vi "working_wendy.vi"() -> ()   [LabVIEW 2015]
doc: "This is the interface, the one VI which loads all the others. Run this one first.\n\n(the line below ensures settings are saved)\n[Red Tweezers Save Settings]"
uses:
  subvis/line_trapping.ctl
  subvis/spot.ctl
  <vilib>/userdefined/High Color/IMAQdx.ctl
  subvis/selection_element.ctl
  subvis/mouse_info.ctl
  <vilib>/imath/engines/lvmath/Plug In/_Char/NIMS_CH_character datatype.ctl
  <vilib>/Analysis/baseanly.llb/Real A x B.vi
  subvis/red_tweezers_globals_INTERNAL_VOLATILE.vi
  subvis/red_tweezers_globals.vi
  <vilib>/imath/engines/lvmath/Plug In/_Char/NIMS_CH_Character RV to String.vi
  <vilib>/imath/engines/lvmath2/RunTimeEngine/BuiltInFunctions/title/NIMS_title.vi
  <vilib>/imathl/engines/lvmath/Functions/Error Handling/Create Error.vi
  <vilib>/imath/engines/lvmath2/RunTimeEngine/BuiltInFunctions/xlimit/NIMS_xlimit.vi
  <vilib>/imath/engines/lvmath2/RunTimeEngine/BuiltInFunctions/ylimit/NIMS_ylimit.vi
  <vilib>/imath/engines/lvmath2/RunTimeEngine/IndexRead/NIMS M($,S).vi
  <instcachedir>/0/NIMS M($,S)_3E5749BBB62E49528D4765A77F1F6D98.lvgen/NIMS M($,S)_3E5749BBB62E49528D4765A77F1F6D98_000.vi
  <vilib>/imath/engines/lvmath2/RunTimeEngine/BuiltInFunctions/plot/NIMS_plot(RM, RM, Str).vi
  <vilib>/imath/engines/lvmath2/RunTimeEngine/ErrorHandling/NIMS_Finalize Error.vi
  <vilib>/Analysis/NI_AALBase.lvlib
  <vilib>/vision/driver/NI_Vision_Acquisition_Software.lvlib
  <vilib>/vision/NI_Vision_Development_Module.lvlib
panel:
  out "Spot Storage":T1[](array[typedef]) {"Amplitude Correction" step=0.1; "Line Trapping"."Phase Gradient" step=0.05; "Line Trapping"."Vector"."x" step=1e-06 format="%#_6p"; "Line Trapping"."Vector"."y" step=1e-06 format="%#_6p"; "Line Trapping"."Vector"."z" step=1e-06 format="%#_6p"; "NA Position"."r" step=1e-06; "NA Position"."y" step=1e-06; "NA Position"."x" step=1e-06; "Position"."z" step=1e-06; "Position"."y" step=1e-06; "Position"."x" step=1e-06; "Phase" step=0.7753; "Intensity" step=0.1}
  out "# selected":i16
  out "Last Pattern":T1[](array[typedef]) {"Amplitude Correction" step=0.1; "Line Trapping"."Phase Gradient" step=0.05; "Line Trapping"."Vector"."x" step=1e-06 format="%#_6p"; "Line Trapping"."Vector"."y" step=1e-06 format="%#_6p"; "Line Trapping"."Vector"."z" step=1e-06 format="%#_6p"; "NA Position"."r" step=1e-06; "NA Position"."y" step=1e-06; "NA Position"."x" step=1e-06; "Position"."z" step=1e-06; "Position"."y" step=1e-06; "Position"."x" step=1e-06; "Phase" step=0.7753; "Intensity" step=0.1}
  out "Plugins":T3(array[cluster])=[{"Name"="ASI Stage", "Folder"=path "C:/Users/Richard Bowman/Dropbox/red_tweezers_1_4_rc4/plugins/ASI Stage.llb", "vi reference"=refnum, "Needs to be run"=TRUE, "Error"={"status"=FALSE, "code"=0, "source"=""}}, {"Name"="iTweezers", "Folder"=path "C:/Users/Richard Bowman/Dropbox/red_tweezers_1_4_rc4/plugins/iTweezers.llb", "vi reference"=refnum, "Needs to be run"=TRUE, "Error"={"status"=FALSE, "code"=0, "source"=""}}, {"Name"="MightexLED", "Folder"=path "C:/Users/Richard Bowman/Dropbox/red_tweezers_1_4_rc4/plugins/MightexLED.llb", "vi reference"=refnum, "Needs to be run"=TRUE, "Error"={"status"=FALSE, "code"=0, "source"=""}}]
  in  "Tab":T4(tab)
  out "Y":dbl
  out "X":dbl
  in  "O Button":bool
  in  "OK Button":bool
  in  "Bubble Size":dbl=50.0002
  out "Hit Indicator":bool
  in  "On":bool
  out "Induce check":bool
  out "Area+ Buffer":dbl
  in  "Area to check":dbl=0.00025
  out "Prev Current Spot":dbl
  out "spots selected 2":i32=4
  out "Spot # Check":dbl
  out "Orig Y SC":dbl
  out "Orig X SC":dbl
  out "ID num check":dbl
  out "Value Check":dbl
  out "ID":dbl[](array[numeric])
  out "Null array":dbl[](array[numeric])
  out "Potential Collisions":dbl
  out "What to Check":dbl[](array[numeric])
  out "String counter":dbl
  out "Counter for String":dbl
  out "Numeric 4":dbl
  out "LCounter":dbl
  out "Numeric 3":dbl
  out "Num":dbl
  out "Old Y":dbl
  out "Old X":dbl
  out "init":dbl
  out "Looper":bool
  in  "Output to SLM":bool
  out "Maximum":dbl
  out "Projected Distance":dbl
  out "Previous Distance":dbl
  out "Group ID #":dbl
  in  "Buffer Zone":dbl=7e-05
  out "# of Spots":dbl
  out "Distance":dbl
  out "Hit":bool
  out "Y Displacement":dbl
  out "X Displacement":dbl
  out "Current Spot #":dbl
  out "spots selected":i32=4
  in  "lock aspect ratio":bool=TRUE
  in  "Size":cluster{"x":dbl, "y":dbl, "z":dbl} {"z" step=1e-06 format="%#_4p"; "y" step=1e-06 format="%#_4p"; "x" step=1e-06 format="%#_4p"}
  in  "Position":cluster{"x":dbl, "y":dbl, "z":dbl}={"x"=1e-06, "y"=-6.3e-06, "z"=0.0} {"z" step=1e-06 format="%#_4p"; "y" step=1e-06 format="%#_4p"; "x" step=1e-06 format="%#_4p"}
  in  "phase":dbl step=0.7753
  in  "Vortex Charge":i8
  in  "Intensity":dbl=1.0 step=0.1
  in  "add to selection":bool
  in  "random position":bool
  in  "new spot":bool
  in  "delete":bool
  in  "rotate":bool
  in  "Rotation Axis":u16(ring)=2 items=["Z", "X", "Y", "Custom"]
  in  "Angle (degrees)":dbl=2.0
  in  "Custom Axis":cluster{dbl, dbl, dbl}
  in  "Spot Shape":enum32{"Normal", "Line", "NA", "Mixed"}(tab)=enum."Mixed"
  in  "Line Trapping":T2 {"Phase Gradient" step=0.05; "Vector"."x" step=1e-06 format="%#_4p"; "Vector"."y" step=1e-06 format="%#_4p"; "Vector"."z" step=1e-06 format="%#_4p"}
  in  "Scale back aperture":dbl=1.1 step=0.1
  in  "Scale BA":bool
  in  "Position on back aperture":cluster{"x":dbl, "y":dbl}={"x"=-5.84327907697451e-18, "y"=0.0} {"y" step=0.1 format="%#_4p"; "x" step=0.1 format="%#_4p"}
  in  "Radius on back aperture":dbl=1.1 step=0.1
  in  "Generate":bool
  in  "Pattern":T5(tab)
  in  "Spots across centre":i32=5
  in  "Reference Array?":bool
  in  "Fraction of SLM":dbl=1.0
  in  "Spots across centre":i32=5
  in  "N":cluster{i32, i32}
  in  "spacing/m":dbl=2.0
  in  "Iterations":i32=10
  out "non-uniformity":dbl(slide)=0.031119223416512406 scale=0.0..0.2
  out "efficiency":dbl(slide)=0.8985936267644501 scale=0.0..1.0
  in  "Optimise":bool
  in  "Reset Phase/Amplitude":bool
  in  "Fall-off/m":dbl=0.00025 min=0.0 step=1e-06 format="%#_4p"
  in  "Abort Plugin":bool
  in  "Plugin:":u16(ring)=1 items=["ASI Stage", "iTweezers", "MightexLED"]
  in  "Save Video":bool
  in  "Global ROI (requires restart)":i32[](array[numeric])=[0, 0, 1280, 512]
  in  "Zoom":bool
  in  "Draw ROI":bool
  in  "Zoom to Fit":bool
  out "Image Information":string="640x480 1.93X 8-bit image 255    (0,0)"
  in  "Camera":T6
  in  "Time per Frame (ms)":dbl
  in  "Edit Sequence Mode":bool
  in  "Manual Edit":bool
  in  "Bubble ID to Empty":dbl
  in  "Clearance Button":bool
  in  "Manual Sequence":bool
  in  "Play Sequence":bool
  in  "Reset":bool
  out "Sequence Instances":dbl
  out "Counter":dbl
  in  "Save State":bool
  out "Sequence On?":bool
  in  "Sequence Order":dbl
  out "Selection/Group":T7[](array[typedef])
  in  "Sequence Storer":T1[][](array[typedef]) {"Amplitude Correction" step=0.1; "Line Trapping"."Phase Gradient" step=0.05; "Line Trapping"."Vector"."x" step=1e-06 format="%#_6p"; "Line Trapping"."Vector"."y" step=1e-06 format="%#_6p"; "Line Trapping"."Vector"."z" step=1e-06 format="%#_6p"; "NA Position"."r" step=1e-06; "NA Position"."y" step=1e-06; "NA Position"."x" step=1e-06; "Position"."z" step=1e-06; "Position"."y" step=1e-06; "Position"."x" step=1e-06; "Phase" step=0.7753; "Intensity" step=0.1}
  in  "Rates":bool
  out "Rates":dbl
  out "LCS":dbl
  in  "Add Additional Frames":bool
  in  "Frame Location":dbl
  in  "Additional Frames Wanted":dbl
  in  "Initiate Creation":bool
  in  "Number of Planned Sequence Frames":dbl
  in  "Max Number of Bubbles":dbl
  in  "Tab Control":enum32{"Line", "Arc"}(tab)
  out "X Rate":dbl
  out "Y Rate":dbl
  out "Degree Rate":dbl
  out "Radians":dbl
  out "Center Y":dbl
  out "Center X":dbl
  in  "Radius X":dbl
  in  "Theta":dbl
  in  "Lock Current Spot":bool
  out "Locked Current Spot":dbl
  out "Numeric":dbl
  out "probe":dbl
  in  "Insert":bool
  in  "Start at Which Frame?":dbl
  out "Original Y":dbl
  out "Original X":dbl
  in  "Mark Original Position":bool
  in  "How Many Frames?":dbl
  out "New Y":dbl
  out "New X":dbl
  out "Spot Storage 2":T1[](array[typedef]) {"Amplitude Correction" step=0.1; "Line Trapping"."Phase Gradient" step=0.05; "Line Trapping"."Vector"."x" step=1e-06 format="%#_6p"; "Line Trapping"."Vector"."y" step=1e-06 format="%#_6p"; "Line Trapping"."Vector"."z" step=1e-06 format="%#_6p"; "NA Position"."r" step=1e-06; "NA Position"."y" step=1e-06; "NA Position"."x" step=1e-06; "Position"."z" step=1e-06; "Position"."y" step=1e-06; "Position"."x" step=1e-06; "Phase" step=0.7753; "Intensity" step=0.1}
  in  "Save":bool
  in  "Load":bool
  in  "Camera Capture":bool
  out "Bubble y":dbl
  out "Bubble x":dbl
  out "Number of Matches Returned":dbl
  out "bottomry":dbl
  out "toply":dbl
  out "bottomrx":dbl
  out "toplx":dbl
  in  "Send Data":bool
  out "Camera 2":T8(plugin-control)
  out "Circles":T9(array[cluster]) {"Position"."Y" format="%.2f"; "Position"."X" format="%.2f"}
  out "Video Frame Rate":dbl(knob)=50.00000000000003 scale=0.0..100.0 scale format="%.1f"
  out "Interface Frame Rate":dbl(knob)=97.23240312927678 scale=0.0..100.0 scale format="%.1f"
  in  "stop":bool=TRUE
  out "1 for original positon":dbl
  out "MOP pressed":bool
  out "MOP pressed After":bool
  out "X Pos every 10 sec":dbl
  out "Elapsed Time":dbl
  out "Sequence Frames To Check":string
  out "Position Indicator":string
  in  "Clear String":bool
  out "String 2":string
  out "Collision Detector":string
  out "Array":dbl[](array[numeric])
  out "Spot Checker":T1[](array[typedef]) {"Amplitude Correction" step=0.1; "Line Trapping"."Phase Gradient" step=0.05; "Line Trapping"."Vector"."x" step=1e-06 format="%#_6p"; "Line Trapping"."Vector"."y" step=1e-06 format="%#_6p"; "Line Trapping"."Vector"."z" step=1e-06 format="%#_6p"; "NA Position"."r" step=1e-06; "NA Position"."y" step=1e-06; "NA Position"."x" step=1e-06; "Position"."z" step=1e-06; "Position"."y" step=1e-06; "Position"."x" step=1e-06; "Phase" step=0.7753; "Intensity" step=0.1}
  out "Image":T8(plugin-control)
  # "Notes:\n\nIf you are doing non-sequence controls,\nthe delete function can be used as intended.\nHowever, do not use the delete function after\nrunning a sequence! Using it will prevent\nthe bubbles from appearing as the\nnumber of spots will change, which is\nessential for the sequence to work (it would\nbe displaying the maximum number of\nbubbles). \n\nIf you happen to delete a bubble, it can be \nrestored by inserting a new spot. Once enough\nspots have been restored, click on manual edit\nto correct the # of spots tracker. It should \nbe restored to where it originally was."
  # "The SLM can be used to shape spots; here you can restrict the NA of a spot (so it comes only from part of the back aperture), or create a line-trap"
  # "The traps do not have any spot-shaping applied (so they should just be diffraction-limited focal spots)."
  # "This shapes the amplitude (and phase) of the beam to create extended line traps.  The \"Phase Gradient\" control allows the Poynting vector to push things along the line.  Unfortunately, some work is needed on the scaling factors so the phase gradient control will need tweaking if the line trap has a nonzero z component."
  # "By default,each spot comes from the whole back aperture.  Here, you can limit a spot to come from a specific part of the back aperture."
  # "The control below allows you to scale the whole back aperture (i.e. the position and size of all the apertures).  It's a one-time operation, i.e. only changes things when you push \"ok\"."
  # "A Combination of line-trapping and NA restriction has been applied to these traps.  You can get at the line trap or NA parameters on the other tabs, switching to the NA tab does not delete the line-trap settings."
  # "This tab generates Shack-Hartmann type holograms, which are often useful when aligning the system, and arrays of spots."
  # "The controls above only work when using the \"IMAQdx with ROI Buttons\" case in the bottom loop.  You can save video regardless of camera code though."
  # "Manual Edit allows a user to\ngo to a specific sequence frame."
  # "To clear the sequence, you must\nclear the array. Right click on sequence\nstorer to do this."
  # "Use this to \"clear\" a \nspecific bubble. If\nworking on a sequence,\nuse this as your delete\nbutton! You can update\nthe view by using manual edit."
  # "Use the reset button\nto clear counter.\nIt becomes necessary\nwhen you clear the array,\nespecially in manual mode."
  # "Use the sequence creator tab to specify the\nnumber of bubbles you want along with\nthe number of frames.\n\nTo save at a specific interval, the sequence\norder can be used to place the state. If used\nto correct something, it will replace the\nentire sequence frame.\n\n\"Sequence On?\" is only used in auto mode."
  # "Frame Location must be\nwhere you want to add\nthe frames to (ie having \n4 as an input would have\nthe additional frames\nstart at array row 5."
  # "Multiple bubbles can  be done with the\nline function. One bubble at a time for the arc\nfunction."
  # "Using the Load/Save function:\n\nRed Tweezers itself is unable to save long \nsequences, but a separate program is able to\naccomplish this. To do this, follow these\nsteps:\n\n1. After creating your sequence, press the save\nbutton below.\n\n2. Then, go to the subvi folder and find\nSequenceSaver.vi.\n\n3. At the control \"Sequence Storer,\" right-click\nthe dimensions part of the array and go to\ndata operations.\n\n4. Press \"Make Current Values Default\" and save\nthe sequence.\n\n5. The next time you load the program, simply\npress load to re-acquire the sequence. You\nwill need to insert the bubbles again, but after\nthe first frame can be recovered by using\nSequenceControl.vi."
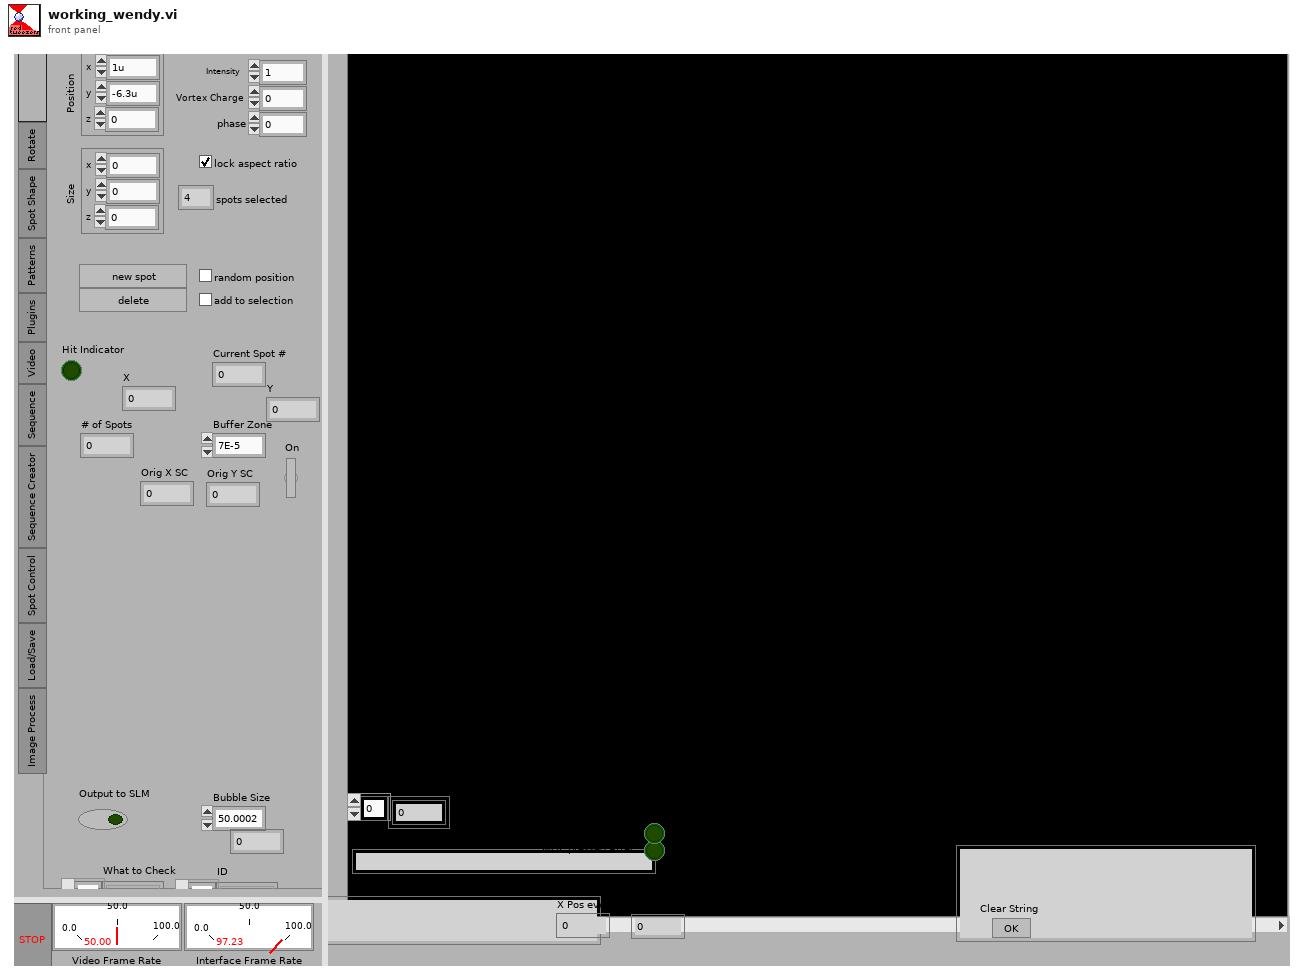
[diagram p1: front panel]
types:
  T1 = typedef "spot.ctl" = cluster{"Position":cluster{"x":dbl, "y":dbl, "z":dbl}, "Intensity":dbl, "Vortex Charge":i8, "Phase":dbl, "NA Position":cluster{"x":dbl, "y":dbl, "r":dbl}, "Line Trapping":T2, "Amplitude Correction":dbl}
  T2 = typedef "line_trapping.ctl" = cluster{"Vector":cluster{"x":dbl, "y":dbl, "z":dbl}, "Phase Gradient":dbl}
  T3 = cluster{"Name":string, "Folder":path, "vi reference":refnum<vi>, "Needs to be run":bool, "Error":errorcluster}[]
  T4 = enum32{"Current Spot", "Rotate", "Spot Shape", "Patterns", "Plugins", "Video", "Sequence", "Sequence Creator", "Spot Control", "Load/Save", "Image Process"}
  T5 = enum32{"HCP Shack-Hartmann", "Square Shack-Hartmann", "Rectangular Grid"}
  T6 = typedef "IMAQdx.ctl" = refnum<k21>
  T7 = typedef "selection_element.ctl" = cluster{"Group ID":i32, "Selected":bool}
  T8 = typedef "IMAQ Image.ctl" = refnum<image>
  T9 = cluster{"Position":cluster{"X":sgl, "Y":sgl}, "Radius":dbl, "Score":dbl}[]
  T10 = typedef "mouse_info.ctl" = cluster{"Button Down":bool, "Dragging":bool, "Position (Image Pixels)":cluster{"X":dbl, "Y":dbl}, "Previous Position (Image Pixels)":cluster{"X":dbl, "Y":dbl}, "Button":u16, "Mods":cluster{"Double Click":bool, "Menu Key":bool}, "PlatMods":cluster{"Shift":bool, "Ctrl":bool, "Alt":bool, "Cmd":bool, "Opt":bool}}
  T11 = typedef "NIMS_CH_character datatype.ctl" = cluster{"Numeric":u8}
  T12 = cluster{"Position":cluster{"x":dbl, "y":dbl, "z":dbl}, "Intensity":dbl, "Vortex Charge":i8, "Phase":dbl, "NA Position":cluster{"x":dbl, "y":dbl, "r":dbl}, "Line Trapping":T2, "Amplitude Correction":dbl}
  T13 = enum16{"Set guide visibility", "Set grid visibility", "Show front panel", "Render on image"}
  T14 = enum32{"Current Spot", "Rotate", "Spot Shape", "Patterns", "Plugins", "Video"}
  T15 = enum16{"Left Button", "Center Button", "Right Button", "Window Close"}
  T16 = typedef "Image Type" = u32
  T17 = cluster{"number: 0 to 1":dbl, "number: 0 to 1":dbl}
  T18 = typedef "NI_Matrix.lvlib/RealMatrix.ctl" = dbl[][]
  T19 = typedef "overlay_element.ctl" = cluster{"Tool":enum16{"Lines", "Oval", "Rectangle", "Text"}, "Points":cluster{"X":dbl, "Y":dbl}[], "Drawing Mode":u32, "Color":u32, "String":string}
  T20 = enum32{"Current Spot", "Rotate", "Spot Shape", "Patterns", "Plugins", "Video", "Particle Tracking", "Clamping", "Blank"}[]
  T21 = typedef "LVMenuShortCut.ctl" = cluster{"include Shift key?":bool, "include Ctrl key?":bool, "shortcut key":string}
  T22 = typedef "LVPoint32TypeDef.ctl" = cluster{"Horizontal":i32, "Vertical":i32}
  T23 = cluster{"Shift":bool, "Ctrl":bool, "Alt":bool, "Cmd":bool, "Opt":bool}
  T24 = cluster{"Button Down":bool, "Dragging":bool, "Mouse Coords (image pixels)":cluster{dbl, dbl}, "Mouse Coords (image pixels)":cluster{dbl, dbl}, "Button":u16, "Mods":cluster{"Double Click":bool, "Menu Key":bool}, "PlatMods":cluster{"Shift":bool, "Ctrl":bool, "Alt":bool, "Cmd":bool, "Opt":bool}}
  T25 = cluster{"Position":cluster{"X":sgl, "Y":sgl}, "Radius":dbl, "Score":dbl}
  T26 = cluster{"[0]":dbl, "[1]":dbl, "[2]":dbl, "[3]":dbl}
  T27 = cluster{"Average Frame Time":dbl, "millisecond timer value":u32}
  T28 = cluster{"Position":cluster{"x":dbl, "y":dbl, "z":dbl}, "Intensity":dbl, "Vortex Charge":i8, "Phase":dbl, "NA Position":cluster{"x":dbl, "y":dbl, "r":dbl}, "Line Trapping":T2, "Amplitude Correction":dbl}[]
  T29 = enum32{"Bad", "Idle", "Run top level", "Running"}
  T30 = typedef "AviRefnum.ctl" = refnum<k1>
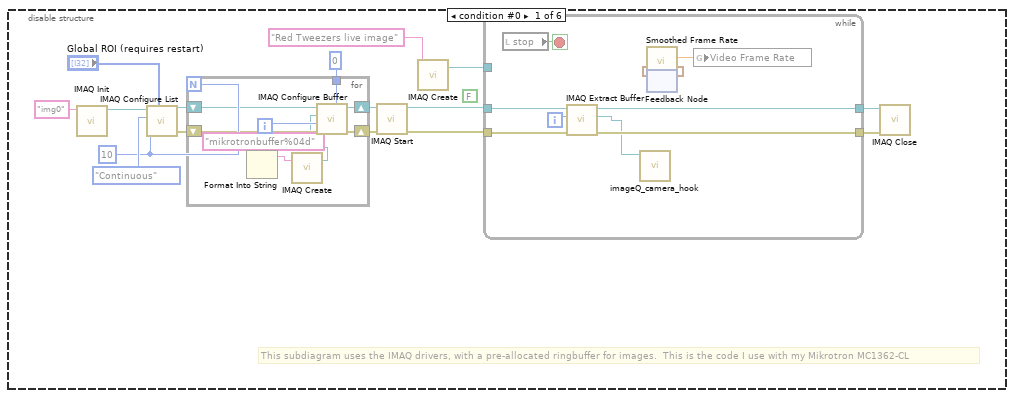
[diagram p3: hidden frame]
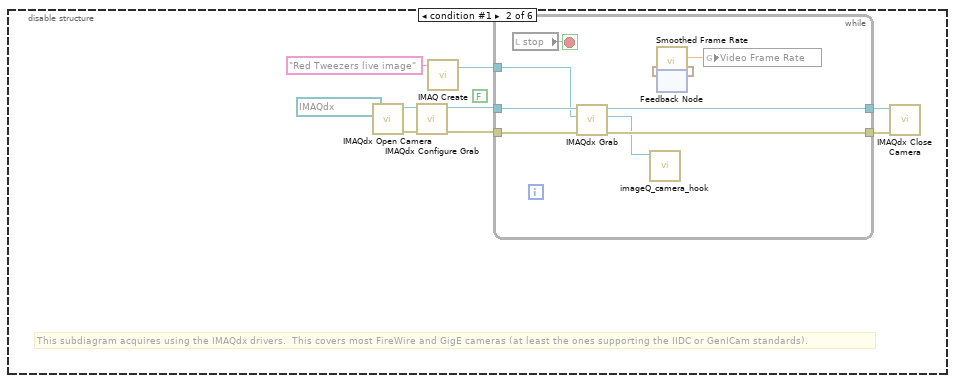
[diagram p4: hidden frame]
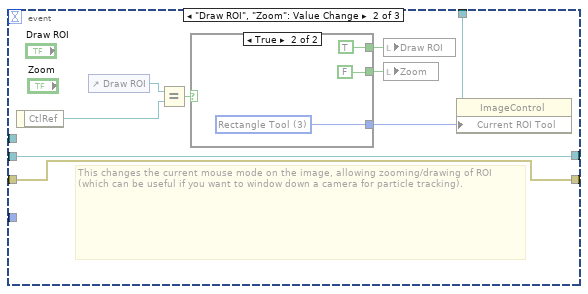
[diagram p5: hidden frame]
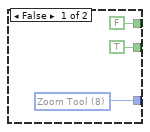
[diagram p6: hidden frame]
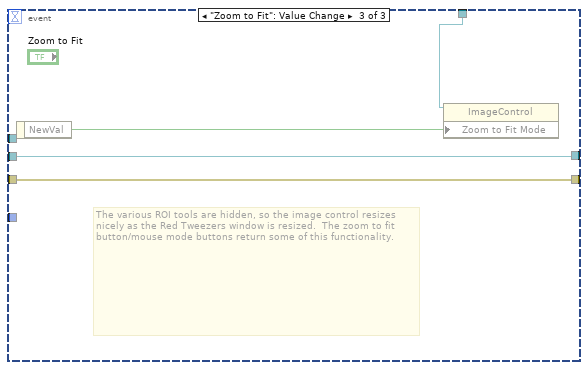
[diagram p7: hidden frame]
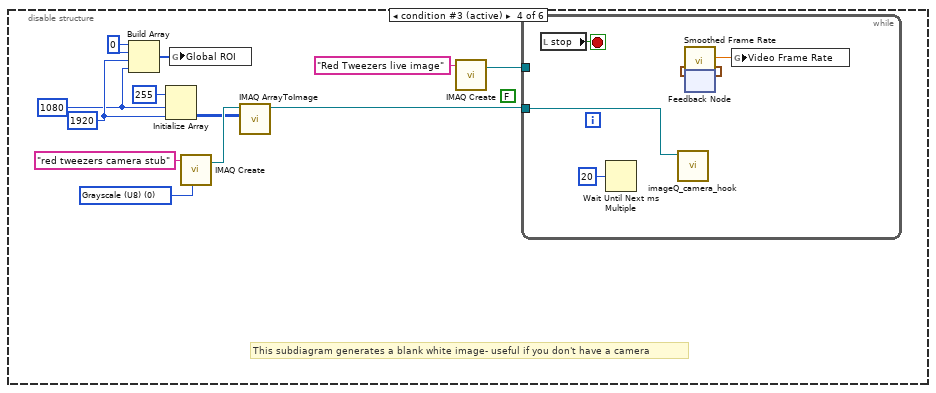
[diagram p8: hidden frame]
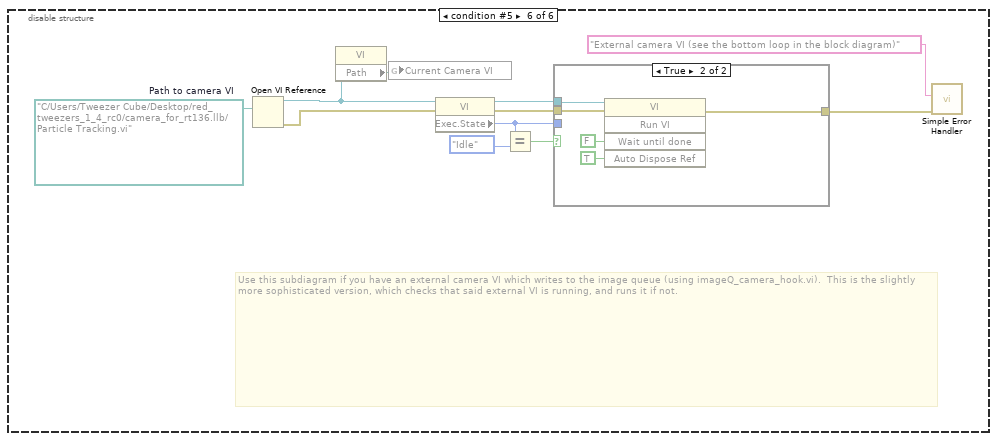
[diagram p10: hidden frame]
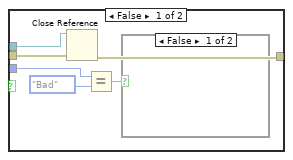
[diagram p11: hidden frame]
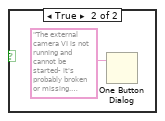
[diagram p12: hidden frame]
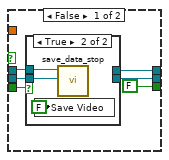
[diagram p13: hidden frame]
diagram:
  w11 = "red_tweezers_display_imageQ" ("Queue Name")
  w23 = T10 {"Button Down"=FALSE, "Dragging"=FALSE, "Position (Image Pixels)"={"X"=0.0, "Y"=0.0}, "Previous Position (Image Pixels)"={"X"=0.0, "Y"=0.0}, "Button"=0, "Mods"={"Double Click"=FALSE, "Menu Key"=FALSE}, "PlatMods"={"Shift"=FALSE, "Ctrl"=FALSE, "Alt"=FALSE, "Cmd"=FALSE, "Opt"=FALSE}}  # Mouse Information
  w24 = refnum<vi> refnum  # Image
  # "The funny looking feedback-node structure is deliberate (if odd).  We want to reload settings from the last used file (stored in the registry) only if this program has not been run since it was last loaded from file/recompiled.  That's why I use an uninitialised shift register: every time the program runs, it increments.  So, if it is zero, this is our first run (or we've been recently recompiled)."
  # "This loop handles the video that is displayed on-screen and saved to file."
  # "Initially, we only register to be told when the user clicks the image"
  # "This is the actual image control"
  # "This is a generic reference.\nIt is just a placeholder, so we can register for events later."
  # "This version of red tweezers uses two coordinate systems: \n1. Real Coordinates - corresponding to physical distances in 3D in microns\n2. Image Coordinates - position on the camera image, relative to the top left of the CURRENT ROI, measured in pixels. If the ROI changes, the relationship between \"real units\" and \"image pixels\" may change, so all values should be stored and presented to the user in REAL units unless there is a good reason to do otherwise."
  n1 = control-ref of="Plugin Pnl"() -> (w20:refnum<vi>)
  n2 = flat-sequence {
    tunnel: [w27] -> w6
    tunnel: w4 -> [_]
    frame #0 {
      n3 = vi-ref "red_tweezers_globals_INTERNAL.vi"() -> (w28:refnum<vi>)
      n4 = property class="VI"(reference=w28) -> ("Path"=w27:path)  [unwired: 1 in, 2 out]
      n5 = global write "red_tweezers_globals_INTERNAL_VOLATILE.vi" "Current Camera VI"(w27) -> ()
    }
  }
  n6 = control-ref of="Plugin:"() -> (w21:refnum<vi>)
  n7 = feedback #1() -> (w14:dbl)  [unwired: 1 in]
  n8 = Equal To 0?(x=w14) -> (x = 0?=w13:bool)
  n9 = Increment(x=w14) -> (x+1=w12:dbl)
  n10 = feedback-in #1(w12) -> ()
  n11 = call "plugins_load.vi"("Sub Panel"=w20, "Plugin Chooser"=w21) -> ("error out"=w15:errorcluster, "Plugins"=w17:T3)  [unwired: 2 in, 2 out]
  "Plugins" <- w17
  n12 = control-ref of="Image"() -> (w5:refnum<vi>)
  n13 = case shown="True" w13 {
    tunnel: w15 -> [_ w29]
    tunnel: [_ w29] -> w4
    frame False {
    }
    frame True {
      n14 = call "settings_load_default_file.vi"("error out"=w29) -> ()
    }
  }
  n15 = flat-sequence {
    tunnel: w4 -> [_]
    tunnel: w2 -> [w31]
    frame #0 {
      # "ensure we don't accidentally start saving video, and run UDP Sender to set up the hologram window."
      n16 = local write "Save Video"(FALSE ("background subtraction")) -> ()
      n17 = call "UDP Sender generic_2.vi"("Spots"=w31) -> ()  [unwired: 2 in, 1 out]
    }
  }
  n18 = global read "red_tweezers_globals.vi" "Selection/Group"() -> (w22:T7[])
  n19 = register-events(w5, w24, w24, w24) -> (reference out=w25:refnum<event-registration>)  [unwired: 2 in, 1 out]
  n20 = global read "red_tweezers_globals.vi" "Spots"() -> (w2:T1[])
  n21 = local write "stop"(FALSE ("STOP")) -> ()
  n22 = call "ensure_selection_matches_spots.vi"("Selection and Groups in"=w22, "Spots"=w2) -> ("Selection and Groups out"=w26:T7[], "Spots (duplicate)"=w1:T1[])  [unwired: 4 in]
  n23 = call "IMAQ Create"("Image Name"=w11) -> ("New Image"=w9:T8)  [unwired: 4 in, 1 out]
  n24 = call "imageQ_create_return_queue.vi"("Queue Name"=w11) -> ("queue out"=w10:refnum<queue>)
  n25 = while {
    shift-right: [w119] -> _
    shift-left: w1 -> [w139]
    shift-right: [w138] -> _
    shift-left: w26 -> [w137]
    shift-right: [w141] -> _
    shift-left: _ -> [w132]
    shift-right: [w140] -> _
    shift-left: _ -> [w131]
    tunnel: w5 -> [w136]
    shift-right: [w130] -> _
    shift-left: w23 -> [w129]
    shift-right: [w133] -> _
    shift-left: w25 -> [w134]
    border: errorcluster {"status"=FALSE, "code"=0, "source"=""} ("error out") -> [_]
    tunnel: [errorcluster {"status"=FALSE, "code"=0, "source"=""} ("error in (no error)")] -> w18
    border: w17 -> [_]
    tunnel: w1 -> [w120]
    stop <- w121 stop-if-true
    w34 = 1
    w43 = 7 items=["Red", "Green", "Blue", "Hue", "Saturation", "Luminance", "Value", "Intensity"] ("Color Plane")
    w47 = T16 0 items=["Grayscale (U8)", "Grayscale (I16)", "Grayscale (SGL)", "Complex (CSG)", "RGB (U32)", "HSL (U32)", "RGB (U64)", "Grayscale (U16)"] ("Image Type")
    # "Don't Need. For Matlab Part."
    # "The function inserts the newly generated sequence for the automatic sequence generator. It also contains the code\nthe code necessary to check whether the bubbles will intersect with each other in the sequence."
    # "This calculates the size of the area including the buffer zone length.\nThe bubble diameter will also be included in the near future."
    # "The statement to the right controls the area that are being chcecked and checks\nwhich bubbles need to be checked.  There are two instances where this activates\nin this case:\n\nWhen a new bubble is selected\nWhen a bubble is deselected, reverting to the last current spot #\n\nThe other case, when the bubble moves out of the area specified, is located\ninside the while loop controlling the bubble movement with a mouse."
    # "Timer function example"
    # "These functions help with the calculations for the sequence generator."
    # "This loads the sequence from the \"saver\" VI. The save function below \"saves\" the sequence into the saver VI."
    # "The VI above is SequenceSaver.vi which contains the\ncode necessary to create a sequence."
    # "This case structure is the Save State structure. This stores\nthe current state of the bubbles (ie position)."
    # "Reset sets the counter back to zero. This is particularly useful \nwhen using the manual sequence."
    # "This case structure helps to continue the sequence.\nThis takes the true case of the Sequence On? function\nor the true case for the Manual Sequence function\nin order to go to the next sequence frame."
    # "This case structure allows for the playing of the sequence.\nThe amount of time it takes to go through the sequence\ncan be edited on the current spot menu."
    # "We only write to the image overlay when we are in one of the tabs, to prevent it disappearing when we are (for example) using the mouse."
    # "These wires control saving undo info. See the VI below's tip strips for details."
    # "Setting these wires to false means:\n(1) dragging moves the selection\n(2) clicking spots changes selection\nset them to true to stop the default mouse behaviour, don't wire them straight through!"
    n26 = event shown="[6] <Image>: Mouse Move" {
      selector: w134 -> [w679 w1351 w1356 w1578 w1606 w1623 w1720 _]
      dyn-events: [w679 w1350 w1356 w1576 w1603 w1624 w1720 _] -> w133
      timeout: 0 -> [_ _ _ _ _ _ _ _]
      tunnel: [w687 _ w1358 w1573 w1608 w1615 w1707 _] -> w141
      tunnel: [w686 _ w1357 w1572 w1607 w1614 w1711 _] -> w140
      tunnel: [w685 _ _ _ _ _ _ _] -> w92
      tunnel: w139 -> [w684 w1346 w1363 w1568 w1601 w1620 w1715 w2038]
      tunnel: [w683 w1346 w1361 w1568 w1601 w1611 w1713 w2038] -> w127
      tunnel: [w682 w1345 w1360 w1557 w1600 w1621 w1703 w2037] -> w126
      tunnel: w137 -> [w681 w1345 w1362 w1557 w1600 w1619 w1714 w2037]
      tunnel: w136 -> [w680 w1347 w1353 w1567 w1604 w1622 w1716 _]
      tunnel: [w678 _ w1355 w1577 T10 {"Button Down"=FALSE, "Dragging"=FALSE, "Position (Image Pixels)"={"X"=0.0, "Y"=0.0}, "Previous Position (Image Pixels)"={"X"=0.0, "Y"=0.0}, "Button"=0, "Mods"={"Double Click"=FALSE, "Menu Key"=FALSE}, "PlatMods"={"Shift"=FALSE, "Ctrl"=FALSE, "Alt"=FALSE, "Cmd"=FALSE, "Opt"=FALSE}} T10 {"Button Down"=FALSE, "Dragging"=FALSE, "Position (Image Pixels)"={"X"=0.0, "Y"=0.0}, "Previous Position (Image Pixels)"={"X"=0.0, "Y"=0.0}, "Button"=0, "Mods"={"Double Click"=FALSE, "Menu Key"=FALSE}, "PlatMods"={"Shift"=FALSE, "Ctrl"=FALSE, "Alt"=FALSE, "Cmd"=FALSE, "Opt"=FALSE}} w1719 _] -> w130
      tunnel: w129 -> [w678 _ w1355 _ _ w1618 w1710 _]
      tunnel: w132 -> [_ _ w1358 w1573 w1608 w1615 w1707 _]
      tunnel: w131 -> [_ _ w1357 w1572 w1607 w1614 w1711 _]
      tunnel: [w677 _ _ _ _ _ _ _] -> w128
      tunnel: [_ _ w1354 _ _ _ TRUE _] -> w125
      tunnel: [_ _ _ TRUE TRUE TRUE FALSE _] -> w124
      tunnel: [TRUE _ _ _ _ _ _ _] -> w122
      tunnel: [_ _ _ _ _ _ _ "stop"] -> w121
      tunnel: w120 -> [_ _ _ _ _ _ w1704 _]
      event Timeout {
        n27 = event-data() -> ()  [unwired: 1 in, 1 out]
        n28 = case shown="\"Current Spot\", Default" "Tab" {
          tunnel: [w703 w971 w1118 w1220 w1301 w1339] -> w683
          tunnel: w684 -> [w700 w973 w1119 w1222 w1301 w1339]
          tunnel: w681 -> [w689 w972 w1116 w1221 w1300 w1338]
          tunnel: [w702 w970 w1117 w1219 w1300 w1338] -> w682
          tunnel: [w690 _ TRUE _ _ _] -> w687
          tunnel: [w690 _ _ _ _ _] -> w686
          tunnel: [_ _ _ FALSE _ _] -> w685
          tunnel: w680 -> [_ _ _ _ _ w1335]
          tunnel: w678 -> [_ _ w1098 _ _ _]
          tunnel: [_ _ w1100 _ _ _] -> w677
          frame "Current Spot", Default {
            w690 = FALSE
            # "The function below contains the code necessary to use the automatic sequence generator to create specific movements. It also helps translate cases where the point is entered in not dragged.\nThis prevents bubbles from intersecting if the bubble is told not to intersect."
            # "If it's out of date, update front panel"
            n29 = call "find_centroid.vi"("Selection and Groups"=w689, "Spots"=w700) -> ("Mean Values"=w698:T1, "size"=w692:cluster{"x":dbl, "y":dbl, "z":dbl}, "centroid"=w693:cluster{"x":dbl, "y":dbl, "z":dbl}, "# selected"=w691:i16)  [unwired: 2 in, 1 out]
            n30 = stacked-sequence {
              tunnel: w691 -> [_ w705]
              frame #0 {
                n31 = local read "spots selected"() -> (→"spots selected 2":i32)
              }
              frame #1 {
                "spots selected" <- w705
              }
            }
            n32 = feedback-in #2(w698) -> ()
            n33 = feedback #2() -> (w699:T1)  [unwired: 1 in]
            n34 = feedback #3() -> (w697:cluster{"x":dbl, "y":dbl, "z":dbl})  [unwired: 1 in]
            n35 = feedback-in #3(w692) -> ()
            n36 = Not Equal?(x=w699, y=w698) -> (x != y?=w696:bool)
            n37 = Not Equal?(x=w697, y=w692) -> (x != y?=w695:bool)
            n38 = Or(x=w696, y=w695) -> (x .or. y?=w694:bool)
            n39 = case shown="True" w694 {
              tunnel: w698 -> [_ w711]
              tunnel: w692 -> [_ w707]
              frame False {
              }
              frame True {
                n40 = Unbundle By Name(w711) -> ("Position"=w706:cluster{"x":dbl, "y":dbl, "z":dbl}, "Intensity"=w709:dbl, "Vortex Charge"=w708:i8, "Phase"=w710:dbl)
                n41 = local write "Size"(w707) -> ()
                n42 = local write "Vortex Charge"(w708) -> ()
                n43 = local write "Intensity"(w709) -> ()
                n44 = local write "Position"(w706) -> ()
                n45 = local write "phase"(w710) -> ()
                n46 = Unbundle By Name(w706) -> ()  [unwired: 2 out]
              }
            }
            n47 = local write "Selection/Group"(w689) -> ()
            n48 = event shown="[3] \"Position\": Value Change" {
              selector: _ -> [_ _ _ _ _ _ _ _]
              dyn-events: _ -> [_ _ _ _ _ _ _ _]
              timeout: 10 -> [_ _ _ _ _ _ _ _]
              tunnel: w700 -> [w713 w717 w731 w754 w858 w903 w929 w952]
              tunnel: w689 -> [w712 w716 w734 w761 w845 w900 w926 w950]
              tunnel: [w713 w715 w732 w753 w846 w901 w927 w951] -> w703
              tunnel: [w712 w714 w733 w761 w845 w900 w926 w950] -> w702
              tunnel: w693 -> [_ _ _ _ w857 _ _ _]
              event Timeout {
                n49 = event-data() -> ()  [unwired: 3 out]
              }
              event "delete": Value Change {
                n50 = event-data() -> ()  [unwired: 7 out]
                n51 = call "delete_selected_spots.vi"("Selection/Group 3"=w716, "Spots 3"=w717) -> ("Selection/Group 2"=w714:T7[], "Spots 2"=w715:T1[])  [unwired: 4 in]
              }
              event "new spot": Value Change {
                # "If we're not adding it to the selection, de-select all the other spots"
                n52 = event-data() -> ()  [unwired: 7 out]
                n53 = call "coords_ROI_currentimage.vi"() -> ("Mono ROI"=w718:i32[])
                n54 = case shown="False" "add to selection" {
                  tunnel: w734 -> [w747 w752]
                  tunnel: [w746 w752] -> w729
                  frame False {
                    n55 = for {
                      tunnel: w747 -> [w750] mode=indexing
                      tunnel: [w751] -> w746 mode=indexing
                      n56 = Unbundle(w750) -> ("Group ID"=w749:i32)  [unwired: 1 out]
                      n57 = Bundle(cluster=w750, "Group ID"=w749, "Selected"=FALSE ("Label.Visible")) -> (w751:T7)
                    }
                  }
                  frame True {
                  }
                }
                n58 = Index Array(array=w718) -> (element #1=w724:i32, element #2=w725:i32, element #3=w723:i32, element #4=w722:i32)  [unwired: 4 in]
                n59 = Bundle("Numeric"=w724, "Numeric"=w725) -> (w719:cluster{"Numeric":i32, "Numeric":i32})  [unwired: 1 in]
                n60 = Bundle("Numeric"=w723, "Numeric"=w722) -> (w721:cluster{"Numeric":i32, "Numeric":i32})  [unwired: 1 in]
                n61 = Subtract(x=w721, y=w719) -> (x-y=w720:cluster{"Numeric":i32, "Numeric":i32})
                n62 = case shown="True" "random position" {
                  tunnel: [w736 w742] -> w727
                  tunnel: w720 -> [_ w738]
                  tunnel: w719 -> [_ w737]
                  frame False {
                    n63 = call "replace_position.vi"("Position"=cluster{"x":dbl, "y":dbl, "z":dbl} {"x"=0.0, "y"=0.0, "z"=0.0}) -> ("Spot"=w736:T1)  [unwired: 1 in, 2 out]
                  }
                  frame True {
                    n64 = Random Number (0-1)() -> (number: 0 to 1=w744:dbl)
                    n65 = Random Number (0-1)() -> (number: 0 to 1=w745:dbl)
                    n66 = Bundle("number: 0 to 1"=w745, "number: 0 to 1"=w744) -> (w743:T17)  [unwired: 1 out]
                    n67 = Multiply(x=w743, y=w738) -> (x*y=w740:cluster{dbl, dbl})
                    n68 = Add(x=w740, y=w737) -> (x+y=w739:cluster{dbl, dbl})
                    n69 = call "coords_image_to_real_currentimage.vi"("Position (pixels on image)"=w739) -> ("Position (real coords)"=w741:cluster{dbl, dbl, "Z":dbl})  [unwired: 9 in]
                    n70 = call "replace_position.vi"("Position"=w741) -> ("Spot"=w742:T1)  [unwired: 1 in, 2 out]
                  }
                }
                n71 = Build Array (concatenate)(w731, w727) -> (w732:T1[])
                n72 = Build Array (concatenate)(w729, cluster{i32, "Label.Visible":bool} {0, "Label.Visible"=TRUE}) -> (w733:T7[])
              }
              event "Position": Value Change {
                # "If the position has changed, translate the spots"
                n73 = event-data() -> ("OldVal"=w759:cluster{"x":dbl, "y":dbl, "z":dbl}, "NewVal"=w760:cluster{"x":dbl, "y":dbl, "z":dbl})  [unwired: 5 out]
                n74 = flat-sequence {
                  tunnel: w761 -> [w765]
                  tunnel: w758 -> [w764]
                  tunnel: w754 -> [w763]
                  tunnel: [w762] -> w755
                  frame #0 {
                    n75 = for {
                      tunnel: w763 -> [w770] mode=indexing
                      tunnel: w765 -> [w767] mode=indexing
                      tunnel: [w769] -> w762 mode=indexing
                      tunnel: w764 -> [w768]
                      n76 = Unbundle(w767) -> ("Selected"=w766:bool)  [unwired: 1 out]
                      n77 = case shown="True" w766 {
                        tunnel: w770 -> [w771 w776]
                        tunnel: [w771 w775] -> w769
                        tunnel: w768 -> [_ w772]
                        frame False {
                        }
                        frame True {
                          n78 = call "extract_position.vi"("Spot"=w776) -> ("Position"=w773:cluster{"x":dbl, "y":dbl, "z":dbl})
                          n79 = Add(x=w773, y=w772) -> (x+y=w774:cluster{"x":dbl, "y":dbl, "z":dbl})
                          n80 = call "replace_position.vi"("Position"=w774, "Spot in"=w776) -> ("Spot"=w775:T1)  [unwired: 2 out]
                        }
                      }
                    }
                  }
                }
                n81 = Subtract(x=w760, y=w759) -> (x-y=w758:cluster{"x":dbl, "y":dbl, "z":dbl})
                n82 = local read "# of Spots"() -> (w757:dbl)
                n83 = stacked-sequence {
                  tunnel: w754 -> [_ w781 _]
                  tunnel: w755 -> [_ w780 _]
                  tunnel: w757 -> [_ w779 _]
                  tunnel: [_ _ w828] -> w756
                  tunnel: w755 -> [_ _ w827]
                  tunnel: w754 -> [_ _ w826]
                  tunnel: [_ _ w825] -> w753
                  frame #0 {
                    n84 = local write "Looper"(FALSE) -> ()
                    "init" <- 0
                  }
                  frame #1 {
                    n85 = for {
                      N: w779 -> [_]
                      tunnel: w781 -> [w786]
                      tunnel: w780 -> [w791]
                      stop <- w792 stop-if-true
                      n86 = local read "init"() -> (w785:dbl)
                      n87 = Index Array(array=w791, index=w785) -> (element=w790:T1)
                      n88 = Index Array(array=w786, index=w785) -> (element=w784:T1)
                      n89 = Unbundle By Name(w790) -> ("Position.x"=w789:dbl, "Position.y"=w788:dbl)
                      n90 = local read "# of Spots"() -> (w787:dbl)
                      n91 = Unbundle By Name(w784) -> ("Position.x"=→"Old X":dbl, "Position.y"=→"Old Y":dbl)
                      n92 = local write "New X"(w789) -> ()
                      n93 = local write "New Y"(w788) -> ()
                      n94 = stacked-sequence {
                        tunnel: w786 -> [w797 _]
                        tunnel: w789 -> [w796 _]
                        tunnel: w788 -> [w795 _]
                        tunnel: w787 -> [w794 _]
                        tunnel: w785 -> [w793 _]
                        frame #0 {
                          n95 = for {
                            N: w794 -> [_]
                            tunnel: w797 -> [w819]
                            tunnel: w796 -> [w818]
                            tunnel: w795 -> [w816]
                            tunnel: w793 -> [w801]
                            i -> [w803]
                            stop <- w802 stop-if-true
                            n96 = Index Array(array=w819, index=w803) -> (element=w820:T1)
                            n97 = Unbundle By Name(w820) -> ("Position.x"=w817:dbl, "Position.y"=w815:dbl)
                            n98 = Subtract(x=w818, y=w817) -> (x-y=w814:dbl)
                            n99 = Subtract(x=w816, y=w815) -> (x-y=w813:dbl)
                            n100 = Square(x=w814) -> (x^2=w812:dbl)
                            n101 = Square(x=w813) -> (x^2=w811:dbl)
                            n102 = local read "# of Spots"() -> (w805:dbl)
                            n103 = Add(x=w812, y=w811) -> (x+y=w810:dbl)
                            n104 = local read "Buffer Zone"() -> (w800:dbl)
                            n105 = Square Root(x=w810) -> (sqrt(x)=w809:dbl)
                            n106 = Multiply(x=2, y=w800) -> (x*y=w798:dbl)
                            n107 = Less?(x=w809, y=w798) -> (x < y?=w807:bool)
                            n108 = Not Equal?(x=w801, y=w803) -> (x != y?=w806:bool)
                            n109 = Equal?(x=w805, y=w803) -> (x = y?=w808:bool)
                            n110 = And(x=w806, y=w807) -> (x .and. y?=w804:bool)
                            "Looper" <- w804
                            n111 = Or(x=w804, y=w808) -> (x .or. y?=w802:bool)
                          }
                        }
                        frame #1 {
                          n112 = local read "Looper"() -> (w821:bool)
                          n113 = case shown="False" w821 {
                            frame False {
                              n114 = local read "init"() -> (w822:dbl)
                              n115 = Add(x=w822, y=1) -> (x+y=w824:dbl)
                              n116 = local write "init"(w824) -> ()
                            }
                            frame True {
                            }
                          }
                        }
                      }
                      n117 = local read "Looper"() -> (w792:bool)
                    }
                  }
                  frame #2 {
                    n118 = local read "Looper"() -> (w829:bool)
                    n119 = case shown="False" w829 {
                      tunnel: w827 -> [w833 _]
                      tunnel: w826 -> [_ w841]
                      tunnel: ["This is an acceptable entry." "ERROR: A bubble will intersect the buffer zone."] -> w828
                      tunnel: [w833 w841] -> w825
                      frame False {
                        n120 = local write "Looper"(FALSE) -> ()
                        n121 = local read "Current Spot #"() -> (w834:dbl)
                        n122 = Index Array(array=w833, index=w834) -> (element=w832:T1)
                        n123 = Unbundle By Name(w832) -> ("Position.x"=w831:dbl, "Position.y"=w830:dbl)
                        n124 = local write "New Y"(w830) -> ()
                        n125 = local write "New X"(w831) -> ()
                      }
                      frame True {
                        # "Restore original position"
                        n126 = local write "Looper"(FALSE) -> ()
                        n127 = local read "Old Y"() -> (w838:dbl)
                        n128 = local read "Old X"() -> (w839:dbl)
                        n129 = local read "Position"() -> (w837:cluster{"x":dbl, "y":dbl, "z":dbl})
                        n130 = Bundle By Name(cluster=w837, "x"=w839, "y"=w838) -> (w840:cluster{"x":dbl, "y":dbl, "z":dbl})
                        n131 = local write "Position"(w840) -> ()
                      }
                    }
                  }
                }
                "Position Indicator" <- w756
              }
              event "Size": Value Change {
                # "If we were constraining the aspect ratio, or preventing a divide by zero, the size control on the FP may be incorrect.  We refresh it in here to stop it displaying a wrong value."
                # "If the size has changed, scale the spots"
                n132 = event-data() -> ("OldVal"=w850:cluster{"x":dbl, "y":dbl, "z":dbl}, "NewVal"=w856:cluster{"x":dbl, "y":dbl, "z":dbl})  [unwired: 5 out]
                n133 = Not Equal?(x=w850, y=w856) -> (x != y?=w849:cluster{"x":bool, "y":bool, "z":bool})
                n134 = Divide(x=w856, y=w850) -> (x/y=w855:cluster{"x":dbl, "y":dbl, "z":dbl})
                n135 = Not Equal To 0?(x=w850) -> (x != 0?=w848:cluster{"x":bool, "y":bool, "z":bool})
                n136 = And(x=w849, y=w848) -> (x .and. y?=w847:cluster{"x":bool, "y":bool, "z":bool})
                n137 = Cluster To Array(cluster=w847) -> (array=w854:bool[])
                n138 = Cluster To Array(cluster=w855) -> (array=w853:dbl[])
                n139 = case shown="True" "lock aspect ratio" {
                  tunnel: w854 -> [w862 w879]
                  tunnel: w853 -> [w861 w877]
                  tunnel: [w859 w869] -> w852
                  frame False {
                    # "We are not constraining the aspect ratio here, so just check we're not introducing NAs"
                    n140 = for {
                      tunnel: w862 -> [w868] mode=indexing
                      tunnel: w861 -> [w864] mode=indexing
                      tunnel: [w866] -> w860 mode=indexing
                      n141 = Not A Number/Path/Refnum?(number/path/refnum=w864) -> (NaN/Path/Refnum?=w865:bool)
                      n142 = Compound Arithmetic op=AND(w868, invert w865) -> (w867:bool)
                      n143 = Select(t=w864, s=w867, f=1.0) -> (s? t:f=w866:dbl)
                    }
                    n144 = Array To Cluster(array=w860) -> (cluster=w859:cluster{"[0]":dbl, "[1]":dbl, "[2]":dbl})
                  }
                  frame True {
                    # "Pick the first element that changed and use it.  Also need to make sure (1) an element did change and (2) everything's valid (no divide by zeros)"
                    n145 = Search 1D Array(1D array=w879, element=TRUE) -> (index of element=w876:i32)  [unwired: 1 in]
                    n146 = Index Array(array=w877, index=w876) -> (element=w872:dbl)
                    n147 = Not A Number/Path/Refnum?(number/path/refnum=w872) -> (NaN/Path/Refnum?=w875:bool)
                    n148 = Less Than 0?(x=w876) -> (x < 0?=w874:bool)
                    n149 = Or(x=w875, y=w874) -> (x .or. y?=w873:bool)
                    n150 = Select(t=1.0, s=w873, f=w872) -> (s? t:f=w870:dbl)
                    n151 = Bundle("x"=w870, "x"=w870, "x"=w870) -> (w869:cluster{"x":dbl, "x":dbl, "x":dbl})  [unwired: 1 in]
                  }
                }
                n152 = for {
                  tunnel: w858 -> [w885] mode=indexing
                  tunnel: w845 -> [w882] mode=indexing
                  tunnel: [w884] -> w846 mode=indexing
                  tunnel: w852 -> [w883]
                  tunnel: w857 -> [w880]
                  n153 = Unbundle(w882) -> ("Selected"=w881:bool)  [unwired: 1 out]
                  n154 = case shown="True" w881 {
                    tunnel: w885 -> [w886 w894]
                    tunnel: [w886 w893] -> w884
                    tunnel: w883 -> [_ w892]
                    tunnel: w880 -> [_ w888]
                    frame False {
                    }
                    frame True {
                      n155 = call "extract_position.vi"("Spot"=w894) -> ("Position"=w890:cluster{"x":dbl, "y":dbl, "z":dbl})
                      n156 = Subtract(x=w890, y=w888) -> (x-y=w891:cluster{"x":dbl, "y":dbl, "z":dbl})
                      n157 = Multiply(x=w891, y=w892) -> (x*y=w889:cluster{"x":dbl, dbl, dbl})
                      n158 = Add(x=w888, y=w889) -> (x+y=w887:cluster{"x":dbl, dbl, dbl})
                      n159 = call "replace_position.vi"("Position"=w887, "Spot in"=w894) -> ("Spot"=w893:T1)  [unwired: 2 out]
                    }
                  }
                }
                n160 = call "find_centroid.vi"("Selection and Groups"=w845, "Spots"=w846) -> ("size"=w844:cluster{"x":dbl, "y":dbl, "z":dbl})  [unwired: 2 in, 4 out]
                n161 = local write "Size"(w844) -> ()
              }
              event "Intensity": Value Change {
                # "When  the user changes intensity, scale all the spots selected so the new mean is correct but keep the ratio between the selected spots.\n\nThe exception to this is when the mean intensity is zero, in which case multiplying makes no sense- in that case we just replace with the new value."
                n162 = event-data() -> ("NewVal"=w895:dbl, "OldVal"=w902:dbl)  [unwired: 5 out]
                n163 = Equal To 0?(x=w902) -> (x = 0?=w898:bool)
                n164 = Not A Number/Path/Refnum?(number/path/refnum=w902) -> (NaN/Path/Refnum?=w897:bool)
                n165 = Or(x=w898, y=w897) -> (x .or. y?=w896:bool)
                n166 = Divide(x=w895, y=w902) -> (x/y=w899:dbl)
                n167 = for {
                  tunnel: w903 -> [w908] mode=indexing
                  tunnel: w900 -> [w910] mode=indexing
                  tunnel: [w907] -> w901 mode=indexing
                  tunnel: w899 -> [w906]
                  tunnel: w896 -> [w905]
                  tunnel: w895 -> [w904]
                  n168 = Unbundle(w910) -> ("Selected"=w909:bool)  [unwired: 1 out]
                  n169 = case shown="True" w909 {
                    tunnel: w908 -> [w911 w918]
                    tunnel: [w911 w915] -> w907
                    tunnel: w906 -> [_ w914]
                    tunnel: w905 -> [_ w913]
                    tunnel: w904 -> [_ w912]
                    frame False {
                    }
                    frame True {
                      n170 = Unbundle By Name(w918) -> ("Intensity"=w916:dbl)
                      n171 = case shown="True" w913 {
                        tunnel: [w921 w922] -> w917
                        tunnel: w916 -> [w920 _]
                        tunnel: w914 -> [w919 _]
                        tunnel: w912 -> [_ w922]
                        frame False {
                          n172 = Multiply(x=w920, y=w919) -> (x*y=w921:dbl)
                        }
                        frame True {
                        }
                      }
                      n173 = Bundle By Name(cluster=w918, "Intensity"=w917) -> (w915:T1)
                    }
                  }
                }
              }
              event "phase": Value Change {
                # "When  the user changes phase, translate the phase of all spots selectedd"
                n174 = event-data() -> ("NewVal"=w924:dbl, "OldVal"=w928:dbl)  [unwired: 5 out]
                n175 = Not A Number/Path/Refnum?(number/path/refnum=w928) -> (NaN/Path/Refnum?=w923:bool)
                n176 = Subtract(x=w924, y=w928) -> (x-y=w925:dbl)
                n177 = for {
                  tunnel: w929 -> [w934] mode=indexing
                  tunnel: w926 -> [w936] mode=indexing
                  tunnel: [w933] -> w927 mode=indexing
                  tunnel: w925 -> [w932]
                  tunnel: w923 -> [w931]
                  tunnel: w924 -> [w930]
                  n178 = Unbundle(w936) -> ("Selected"=w935:bool)  [unwired: 1 out]
                  n179 = case shown="False" w935 {
                    tunnel: w934 -> [w937 w944]
                    tunnel: [w937 w941] -> w933
                    tunnel: w932 -> [_ w940]
                    tunnel: w931 -> [_ w939]
                    tunnel: w930 -> [_ w938]
                    frame False {
                    }
                    frame True {
                      n180 = Unbundle By Name(w944) -> ("Phase"=w942:dbl)
                      n181 = case shown="False" w939 {
                        tunnel: [w947 w948] -> w943
                        tunnel: w942 -> [w946 _]
                        tunnel: w940 -> [w945 _]
                        tunnel: w938 -> [_ w948]
                        frame False {
                          n182 = Add(x=w946, y=w945) -> (x+y=w947:dbl)
                        }
                        frame True {
                        }
                      }
                      n183 = Bundle By Name(cluster=w944, "Phase"=w943) -> (w941:T1)
                    }
                  }
                }
              }
              event "Vortex Charge": Value Change {
                # "When  the user changes l, just set all selected spots to have that value of l."
                n184 = event-data() -> ("NewVal"=w949:i8)  [unwired: 6 out]
                n185 = for {
                  tunnel: w952 -> [w955] mode=indexing
                  tunnel: w950 -> [w957] mode=indexing
                  tunnel: [w954] -> w951 mode=indexing
                  tunnel: w949 -> [w953]
                  n186 = Unbundle(w957) -> ("Selected"=w956:bool)  [unwired: 1 out]
                  n187 = case shown="True" w956 {
                    tunnel: w955 -> [w958 w961]
                    tunnel: [w958 w960] -> w954
                    tunnel: w953 -> [_ w959]
                    frame False {
                    }
                    frame True {
                      n188 = Bundle By Name(cluster=w961, "Vortex Charge"=w959) -> (w960:T1)
                    }
                  }
                }
              }
            }
          }
          frame "Spot Shape" {
            # "We update the spot shape tab only when spots have changed OUTSIDE this tab.  This avoids unnecessary jumping about of the tab control."
            n189 = call "find_centroid.vi"("Selection and Groups"=w972, "Spots"=w973) -> ("Mean Values"=w968:T1)  [unwired: 2 in, 4 out]
            n190 = Wait (ms)(milliseconds to wait=u32 10) -> ()  [unwired: 1 out]
            n191 = call "spots_shape.vi"("Selection and Groups"=w972, "Spots"=w973) -> ("Spot Shape"=w975:enum32{"Normal", "Line", "NA", "Mixed"})  [unwired: 7 in]
            n192 = feedback-in #4(w968) -> ()
            n193 = feedback #4() -> (w969:T1)  [unwired: 1 in]
            n194 = Not Equal?(x=w969, y=w968) -> (x != y?=w974:bool)
            n195 = feedback #5() -> (w964:enum32{"Normal", "Line", "NA", "Mixed"})  [unwired: 1 in]
            n196 = feedback #6() -> (w966:T1)  [unwired: 1 in]
            n197 = Not Equal?(x=w966, y=w968) -> (x != y?=w965:bool)
            n198 = case shown="False" w965 {
              tunnel: w975 -> [_ w1094]
              tunnel: ["Spot Shape" w1094] -> w963
              frame False {
              }
              frame True {
                n199 = local write "Spot Shape"(w1094) -> ()
              }
            }
            n200 = feedback-in #5(w963) -> ()
            n201 = Not Equal?(x=w963, y=w964) -> (x != y?=w962:bool)
            n202 = case shown="\"Normal\", Default" w963 {
              tunnel: w973 -> [w979 w996 w1022 w1092]
              tunnel: w972 -> [w978 w995 w1021 w1091]
              tunnel: [w978 w994 w1019 w1091] -> w970
              tunnel: [w977 w993 w1020 w1092] -> w971
              tunnel: w968 -> [_ w992 w1018 _]
              tunnel: w974 -> [_ w991 w1017 _]
              tunnel: w962 -> [_ w989 w1015 _]
              frame "Normal", Default {
                # "If \"normal\" is selected, don't allow any NA or line-trapping stuff"
                n203 = for {
                  tunnel: w979 -> [w982] mode=indexing
                  tunnel: w978 -> [w981] mode=indexing
                  tunnel: [w983] -> w977 mode=indexing
                  n204 = Unbundle(w981) -> ("Selected"=w980:bool)  [unwired: 1 out]
                  n205 = case shown="True" w980 {
                    tunnel: [w984 w988] -> w983
                    tunnel: w982 -> [w984 w987]
                    frame False {
                    }
                    frame True {
                      n206 = Bundle By Name(cluster=w987, "NA Position"=cluster{"x":dbl, "y":dbl, "r":dbl} {"x"=0.0, "y"=0.0, "r"=1.0} ("x"), "Line Trapping"=T2 {"Vector"={"x"=0.0, "y"=0.0, "z"=0.0}, "Phase Gradient"=0.0}) -> (w988:T1)
                    }
                  }
                }
              }
              frame "Line" {
                # "If it's out of date, update front panel"
                n207 = Or(x=w991, y=w989) -> (x .or. y?=w990:bool)
                n208 = case shown="True" w990 {
                  tunnel: w992 -> [_ w999]
                  frame False {
                  }
                  frame True {
                    n209 = Unbundle By Name(w999) -> ("Line Trapping"=w998:T2)
                    n210 = local write "Line Trapping"(w998) -> ()
                  }
                }
                n211 = event shown="[1] \"Line Trapping\": Value Change" {
                  selector: _ -> [_ _]
                  dyn-events: _ -> [_ _]
                  timeout: 10 -> [_ _]
                  tunnel: w996 -> [w1001 w1005]
                  tunnel: w995 -> [w1000 w1003]
                  tunnel: [w1001 w1004] -> w993
                  tunnel: [w1000 w1003] -> w994
                  event Timeout {
                    n212 = event-data() -> ()  [unwired: 3 out]
                  }
                  event Value Change {
                    # "If the line vector has changed, update it"
                    n213 = event-data() -> ("NewVal"=w1002:T2)  [unwired: 6 out]
                    n214 = for {
                      tunnel: w1005 -> [w1010] mode=indexing
                      tunnel: w1003 -> [w1007] mode=indexing
                      tunnel: [w1009] -> w1004 mode=indexing
                      tunnel: w1002 -> [w1008]
                      n215 = Unbundle(w1007) -> ("Selected"=w1006:bool)  [unwired: 1 out]
                      n216 = case shown="True" w1006 {
                        tunnel: w1010 -> [w1011 w1013]
                        tunnel: [w1011 w1014] -> w1009
                        tunnel: w1008 -> [_ w1012]
                        frame False {
                        }
                        frame True {
                          n217 = Bundle By Name(cluster=w1013, "Line Trapping"=w1012) -> (w1014:T1)
                        }
                      }
                    }
                  }
                }
              }
              frame "NA" {
                n218 = Or(x=w1015, y=w1017) -> (x .or. y?=w1016:bool)
                n219 = case shown="True" w1016 {
                  tunnel: w1018 -> [_ w1027]
                  frame False {
                  }
                  frame True {
                    n220 = Unbundle By Name(w1027) -> ("NA Position"=w1026:cluster{"x":dbl, "y":dbl, "r":dbl})
                    n221 = call "xyz_to_xy.vi"("Position"=w1026) -> ("Position (2D)"=w1025:cluster{"x":dbl, "y":dbl}, "z"=w1024:dbl)  [unwired: 6 out]
                    n222 = local write "Position on back aperture"(w1025) -> ()
                    n223 = local write "Radius on back aperture"(w1024) -> ()
                  }
                }
                n224 = event shown="[3] \"Scale BA\": Value Change" {
                  selector: _ -> [_ _ _ _]
                  dyn-events: _ -> [_ _ _ _]
                  timeout: 10 -> [_ _ _ _]
                  tunnel: w1022 -> [w1029 w1035 w1056 w1078]
                  tunnel: w1021 -> [w1028 w1033 w1053 w1079]
                  tunnel: [w1029 w1034 w1054 w1076] -> w1020
                  tunnel: [w1028 w1033 w1053 w1079] -> w1019
                  event Timeout {
                    n225 = event-data() -> ()  [unwired: 3 out]
                  }
                  event "Position on back aperture": Value Change {
                    # "If the position has changed, translate the spots"
                    n226 = event-data() -> ("OldVal"=w1031:cluster{"x":dbl, "y":dbl}, "NewVal"=w1032:cluster{"x":dbl, "y":dbl})  [unwired: 5 out]
                    n227 = Subtract(x=w1032, y=w1031) -> (x-y=w1030:cluster{"x":dbl, "y":dbl})
                    n228 = for {
                      tunnel: w1035 -> [w1040] mode=indexing
                      tunnel: w1033 -> [w1037] mode=indexing
                      tunnel: [w1039] -> w1034 mode=indexing
                      tunnel: w1030 -> [w1038]
                      n229 = Unbundle(w1037) -> ("Selected"=w1036:bool)  [unwired: 1 out]
                      n230 = case shown="True" w1036 {
                        tunnel: w1040 -> [w1041 w1043]
                        tunnel: [w1041 w1044] -> w1039
                        tunnel: w1038 -> [_ w1045]
                        frame False {
                        }
                        frame True {
                          n231 = Unbundle By Name(w1043) -> ("NA Position"=w1047:cluster{"x":dbl, "y":dbl, "r":dbl})
                          n232 = call "xy_to_xyz.vi"("Position (2D)"=w1045) -> ("Position (3D)"=w1046:cluster{dbl, dbl, dbl})  [unwired: 1 in, 2 out]
                          n233 = Add(x=w1047, y=w1046) -> (x+y=w1042:cluster{dbl, dbl, dbl})
                          n234 = Bundle By Name(cluster=w1043, "NA Position"=w1042) -> (w1044:T1)
                        }
                      }
                    }
                  }
                  event "Radius on back aperture": Value Change {
                    # "When  the user changes intensity, scale all the spots selected so the new mean is correct but keep the ratio between the selected spots.\n\nThe exception to this is when the mean intensity is zero, in which case multiplying makes no sense- in that case we just replace with the new value."
                    n235 = event-data() -> ("NewVal"=w1048:dbl, "OldVal"=w1055:dbl)  [unwired: 5 out]
                    n236 = Equal To 0?(x=w1055) -> (x = 0?=w1051:bool)
                    n237 = Not A Number/Path/Refnum?(number/path/refnum=w1055) -> (NaN/Path/Refnum?=w1050:bool)
                    n238 = Or(x=w1051, y=w1050) -> (x .or. y?=w1049:bool)
                    n239 = Divide(x=w1048, y=w1055) -> (x/y=w1052:dbl)
                    n240 = for {
                      tunnel: w1056 -> [w1061] mode=indexing
                      tunnel: w1053 -> [w1063] mode=indexing
                      tunnel: [w1060] -> w1054 mode=indexing
                      tunnel: w1052 -> [w1059]
                      tunnel: w1049 -> [w1058]
                      tunnel: w1048 -> [w1057]
                      n241 = Unbundle(w1063) -> ("Selected"=w1062:bool)  [unwired: 1 out]
                      n242 = case shown="True" w1062 {
                        tunnel: w1061 -> [w1064 w1071]
                        tunnel: [w1064 w1068] -> w1060
                        tunnel: w1059 -> [_ w1067]
                        tunnel: w1058 -> [_ w1066]
                        tunnel: w1057 -> [_ w1065]
                        frame False {
                        }
                        frame True {
                          n243 = Unbundle By Name(w1071) -> ("NA Position.r"=w1069:dbl)
                          n244 = case shown="False" w1066 {
                            tunnel: [w1074 w1075] -> w1070
                            tunnel: w1069 -> [w1073 _]
                            tunnel: w1067 -> [w1072 _]
                            tunnel: w1065 -> [_ w1075]
                            frame False {
                              n245 = Multiply(x=w1073, y=w1072) -> (x*y=w1074:dbl)
                            }
                            frame True {
                            }
                          }
                          n246 = Bundle By Name(cluster=w1071, "NA Position.r"=w1070) -> (w1068:T1)
                        }
                      }
                    }
                  }
                  event "Scale BA": Value Change {
                    n247 = event-data() -> ()  [unwired: 7 out]
                    n248 = for {
                      tunnel: w1079 -> [w1084] mode=indexing
                      tunnel: w1078 -> [w1082] mode=indexing
                      tunnel: "Scale back aperture" -> [w1081]
                      tunnel: [w1080] -> w1076 mode=indexing
                      n249 = Unbundle(w1084) -> ("Selected"=w1083:bool)  [unwired: 1 out]
                      n250 = case shown="True" w1083 {
                        tunnel: w1082 -> [w1085 w1086]
                        tunnel: w1081 -> [_ w1089]
                        tunnel: [w1085 w1087] -> w1080
                        frame False {
                        }
                        frame True {
                          n251 = Unbundle By Name(w1086) -> ("NA Position"=w1090:cluster{"x":dbl, "y":dbl, "r":dbl})
                          n252 = Multiply(x=w1089, y=w1090) -> (x*y=w1088:cluster{"x":dbl, "y":dbl, "r":dbl})
                          n253 = Bundle By Name(cluster=w1086, "NA Position"=w1088) -> (w1087:T1)
                        }
                      }
                    }
                  }
                }
              }
              frame "Mixed" {
              }
            }
            n254 = call "find_centroid.vi"("Selection and Groups"=w970, "Spots"=w971) -> ("Mean Values"=w967:T1)  [unwired: 2 in, 4 out]
            n255 = feedback-in #6(w967) -> ()
          }
          frame "Rotate" {
            w1105 = u32 0 items=["Frame", "Fill", "Highlight"] ("Drawing Mode")
            w1104 = u32 0 ("Color")
            w1101 = i16 100 ("radius")
            # "It's necessary to check this has changed to stop us unintentionally \"spinning\" the spots..."
            # "Draw the centroid as a spot, then a large circle+cross"
            # "It's important that this loop doesn't go too fast- it hogs the CPU.  However, each tab can have a different loop speed."
            n256 = Unbundle By Name(w1098) -> ("Position (Image Pixels)"=w1114:cluster{"X":dbl, "Y":dbl}, "Previous Position (Image Pixels)"=w1113:cluster{"X":dbl, "Y":dbl}, "Dragging"=w1115:bool)
            n257 = feedback-in #7(w1098) -> ()
            n258 = feedback #7() -> (w1099:T10)  [unwired: 1 in]
            n259 = call "find_centroid.vi"("Selection and Groups"=w1116, "Spots"=w1119) -> ("centroid"=w1112:cluster{"x":dbl, "y":dbl, "z":dbl})  [unwired: 2 in, 4 out]
            n260 = Not Equal?(x=w1098, y=w1099) -> (x != y?=w1096:bool)
            n261 = Wait (ms)(milliseconds to wait=u32 10) -> ()  [unwired: 1 out]
            n262 = And(x=w1096, y=w1115) -> (x .and. y?=w1097:bool)
            n263 = call "coords_real_to_image_currentview.vi"("Position (real coords)"=w1112) -> ("Position (pixels, relative to the top left of the image)"=w1095:cluster{dbl, dbl})  [unwired: 7 in, 1 out]
            n264 = case shown="True" w1097 {
              tunnel: w1119 -> [w1128 w1172]
              tunnel: [w1130 w1171] -> w1118
              tunnel: w1116 -> [w1129 w1173]
              tunnel: [w1129 w1173] -> w1117
              tunnel: w1112 -> [w1127 w1164]
              tunnel: w1114 -> [_ w1163]
              tunnel: w1113 -> [_ w1162]
              tunnel: w1095 -> [_ w1161]
              frame False {
                n265 = event shown="[1] Timeout" {
                  selector: _ -> [_ _]
                  dyn-events: _ -> [_ _]
                  timeout: 10 -> [_ _]
                  tunnel: [w1143 w1160] -> w1130
                  tunnel: w1129 -> [w1142 _]
                  tunnel: w1128 -> [w1141 w1160]
                  tunnel: w1127 -> [w1137 _]
                  event "rotate": Value Change {
                    n266 = event-data() -> ()  [unwired: 6 out]
                    n267 = case shown="3" "Rotation Axis" {
                      tunnel: [cluster{dbl, dbl, dbl} {0.0, 0.0, 1.0} ("Custom Axis") cluster{dbl, dbl, dbl} {1.0, 0.0, 0.0} ("Custom Axis") cluster{dbl, dbl, dbl} {0.0, 1.0, 0.0} ("Custom Axis") "Custom Axis"] -> w1138
                      frame 0, Default {
                        # "Z"
                      }
                      frame 1 {
                        # "X"
                      }
                      frame 2 {
                        # "Y"
                      }
                      frame 3 {
                      }
                    }
                    n268 = call "normalise_3d_vector.vi"("Vector"=w1138) -> ("Unit Vector"=w1140:cluster{dbl, dbl, dbl})  [unwired: 3 out]
                    n269 = Divide(x=6.283185307179586, y=360.0) -> (x/y=w1135:dbl)
                    n270 = Multiply(x="Angle (degrees)", y=w1135) -> (x*y=w1132:dbl)
                    n271 = call "arb_rotation_matrix.vi"("Unit Vector"=w1140, "theta"=w1132) -> ("Real Matrix"=w1144:T18)
                    n272 = for {
                      tunnel: w1142 -> [w1154] mode=indexing
                      tunnel: w1141 -> [w1149] mode=indexing
                      tunnel: [w1150] -> w1143 mode=indexing
                      tunnel: w1137 -> [w1152]
                      tunnel: w1144 -> [w1151]
                      n273 = Unbundle(w1154) -> ("Selected"=w1153:bool)  [unwired: 1 out]
                      n274 = case shown="True" w1153 {
                        tunnel: w1152 -> [_ w1159]
                        tunnel: [w1155 w1158] -> w1150
                        tunnel: w1149 -> [w1155 w1157]
                        tunnel: w1151 -> [_ w1156]
                        frame False {
                        }
                        frame True {
                          n275 = call "apply_matrix_transformation_to_spots.vi"("Transform centre (i.e. transform about this point)"=w1159, "Transformation Matrix (3x3)"=w1156, "Spot In"=w1157) -> ("Spot Out"=w1158:T1)  [unwired: 5 out]
                        }
                      }
                    }
                  }
                  event Timeout {
                    n276 = event-data() -> ()  [unwired: 4 out]
                  }
                }
              }
              frame True {
                # "if the mouse has not moved, stuff will be NaN, so let's make like a leopard and not change our spots"
                # "the magnitude of the change in our direction vector gives the rotation angle in radians"
                # "If it's within 100px of the centroid, pretend the mouse is on the surface of a sphere, and synthesize Z accordingly (z^2=100^2-x^2-y^2).  This allows rotation in 3d :)  The output should always be a unit vector."
                n277 = Build Array(w1163, w1162) -> (w1178:cluster{"X":dbl, "Y":dbl}[])
                n278 = for {
                  tunnel: w1161 -> [w1211]
                  tunnel: w1178 -> [w1207] mode=indexing
                  tunnel: [w1197] -> w1177 mode=indexing
                  n279 = Subtract(x=w1207, y=w1211) -> (x-y=w1202:cluster{dbl, dbl})
                  n280 = Divide(x=w1202, y=100.0 ("x")) -> (x/y=w1203:cluster{dbl, dbl})
                  n281 = Square(x=w1203) -> (x^2=w1210:cluster{dbl, dbl})
                  n282 = Unbundle(w1210) -> (w1208:dbl, w1209:dbl)
                  n283 = Add(x=w1208, y=w1209) -> (x+y=w1199:dbl)
                  n284 = Subtract(x=1.0, y=w1199) -> (x-y=w1205:dbl)
                  n285 = Square Root(x=w1199) -> (sqrt(x)=w1200:dbl)
                  n286 = Greater Than 0?(x=w1205) -> (x > 0?=w1206:bool)
                  n287 = case shown="False" w1206 {
                    tunnel: w1205 -> [_ w1218]
                    tunnel: [0.0 w1217] -> w1196
                    tunnel: w1203 -> [w1215 w1216]
                    tunnel: w1200 -> [w1214 _]
                    tunnel: [w1213 w1216] -> w1198
                    frame False {
                      n288 = Divide(x=w1215, y=w1214) -> (x/y=w1213:cluster{dbl, dbl})
                    }
                    frame True {
                      n289 = Square Root(x=w1218) -> (sqrt(x)=w1217:dbl)
                    }
                  }
                  n290 = call "xy_to_xyz.vi"("z"=w1196, "Position (2D)"=w1198) -> ("Position (3D)"=w1197:cluster{dbl, dbl, dbl})  [unwired: 2 out]
                }
                n291 = Index Array(array=w1177) -> (element #1=w1176:cluster{dbl, dbl, dbl}, element #2=w1167:cluster{dbl, dbl, dbl})  [unwired: 2 in]
                n292 = Add(x=w1176, y=w1167) -> (x+y=w1166:cluster{dbl, dbl, dbl})
                n293 = Subtract(x=w1176, y=w1167) -> (x-y=w1165:cluster{dbl, dbl, dbl})
                n294 = call "cross_product.vi"("b"=w1166, "a"=w1165) -> ("a cross b"=w1175:cluster{dbl, dbl, dbl})
                n295 = call "normalise_3d_vector.vi"("Vector"=w1175) -> ("Unit Vector"=w1174:cluster{dbl, dbl, dbl})  [unwired: 3 out]
                n296 = call "normalise_3d_vector.vi"("Vector"=w1165) -> ("magnitude"=w1169:dbl)  [unwired: 3 out]
                n297 = Not Equal To 0?(x=w1169) -> (x != 0?=w1168:bool)
                n298 = call "arb_rotation_matrix.vi"("Unit Vector"=w1174, "theta"=w1169) -> ("Real Matrix"=w1170:T18)
                n299 = case shown="True" w1168 {
                  tunnel: w1173 -> [_ w1184]
                  tunnel: w1172 -> [w1179 w1183]
                  tunnel: [w1179 w1182] -> w1171
                  tunnel: w1170 -> [_ w1181]
                  tunnel: w1164 -> [_ w1180]
                  frame False {
                  }
                  frame True {
                    n300 = for {
                      tunnel: w1184 -> [w1190] mode=indexing
                      tunnel: w1183 -> [w1187] mode=indexing
                      tunnel: [w1186] -> w1182 mode=indexing
                      tunnel: w1181 -> [w1188]
                      tunnel: w1180 -> [w1185]
                      n301 = Unbundle(w1190) -> ("Selected"=w1189:bool)  [unwired: 1 out]
                      n302 = case shown="True" w1189 {
                        tunnel: [w1191 w1194] -> w1186
                        tunnel: w1187 -> [w1191 w1195]
                        tunnel: w1188 -> [_ w1192]
                        tunnel: w1185 -> [_ w1193]
                        frame False {
                        }
                        frame True {
                          n303 = call "apply_matrix_transformation_to_spots.vi"("Transform centre (i.e. transform about this point)"=w1193, "Transformation Matrix (3x3)"=w1192, "Spot In"=w1195) -> ("Spot Out"=w1194:T1)  [unwired: 5 out]
                        }
                      }
                    }
                  }
                }
              }
            }
            n304 = call "coords_real_to_image_currentview.vi"("Position (real coords)"=w1112) -> ("Position (pixels, relative to the top left of the image)"=w1107:cluster{dbl, dbl}, "z (real coords)"=w1111:dbl)  [unwired: 7 in]
            n305 = expression code="z*1e7+20"(w1111) -> (w1123:dbl)
            n306 = In Range and Coerce(upper limit=100.0, x=w1123, lower limit=2.0) -> (coerced(x)=w1110:dbl)  [unwired: 1 out]
            n307 = Bundle("upper limit"=w1110, "upper limit"=w1110) -> (w1103:cluster{"upper limit":dbl, "upper limit":dbl})  [unwired: 1 in]
            n308 = call "myoverlay_oval.vi"("Color"=w1104, "Drawing Mode"=w1105, "Size"=w1103, "Centre Position (pixels on image)"=w1107) -> ("Overlay Elements Out"=w1109:T19[])  [unwired: 5 in]
            n309 = Bundle("radius"=w1101, "radius"=w1101) -> (w1102:cluster{"radius":i16, "radius":i16})  [unwired: 1 in]
            n310 = call "myoverlay_oval.vi"("Color"=w1104, "Drawing Mode"=w1105, "Size"=w1102, "Centre Position (pixels on image)"=w1107, "Overlay Elements In"=w1109) -> ("Overlay Elements Out"=w1108:T19[])  [unwired: 4 in]
            n311 = Multiply(x=w1101, y=cluster{dbl, dbl}[] [{0.0, 0.0}, {1.0, 0.0}, {0.0, 0.0}, {0.0, 1.0}, {0.0, 0.0}, {-1.0, 0.0}, {0.0, 0.0}, {0.0, -1.0}, {0.0, 0.0}]) -> (x*y=w1120:cluster{dbl, dbl}[])
            n312 = Add(x=w1107, y=w1120) -> (x+y=w1106:cluster{dbl, dbl}[])
            n313 = call "myoverlay_lines.vi"("Color"=w1104, "Drawing Mode"=w1105, "Line Endpoints"=w1106, "Overlay Elements In"=w1108) -> ("Overlay Elements Out"=w1100:T19[])  [unwired: 5 in]
          }
          frame "Patterns" {
            n314 = event shown="[3] \"Optimise\": Value Change" {
              selector: _ -> [_ _ _ _ _]
              dyn-events: _ -> [_ _ _ _ _]
              timeout: u32 10 ("milliseconds to wait") -> [_ _ _ _ _]
              tunnel: [w1237 w1267 w1271 w1274 w1285] -> w1220
              tunnel: [w1236 w1268 w1270 w1277 w1286] -> w1219
              tunnel: w1222 -> [w1235 w1267 w1271 w1275 w1284]
              tunnel: w1221 -> [w1234 w1268 w1270 w1277 w1286]
              event "Generate": Value Change {
                # "If there were previous spots, centre the pattern on the spots"
                n315 = event-data() -> ()  [unwired: 1 in, 1 out]
                n316 = call "find_centroid.vi"("Selection and Groups"=w1234, "Spots"=w1235) -> ("size"=w1230:cluster{"x":dbl, "y":dbl, "z":dbl}, "centroid"=w1226:cluster{"x":dbl, "y":dbl, "z":dbl}, "# selected"=w1232:i16)  [unwired: 2 in, 2 out]
                n317 = Greater?(x=w1232, y=i16 1) -> (0:w1227:bool)
                n318 = case shown="False" w1227 {
                  tunnel: w1230 -> [_ w1253]
                  tunnel: [cluster{"x":dbl, "y":dbl, "z":dbl} {"x"=2e-05, "y"=2e-05, "z"=2e-05} ("size") w1253] -> w1229
                  frame False {
                  }
                  frame True {
                  }
                }
                n319 = case shown="\"HCP Shack-Hartmann\"" "Pattern" {
                  tunnel: [w1255 w1258 w1264] -> w1228
                  tunnel: w1229 -> [_ w1257 _]
                  frame "Square Shack-Hartmann" {
                    n320 = call "patterns_square_shack_hartmann.vi"("N"="Spots across centre") -> ("Spots"=w1255:T1[])
                  }
                  frame "HCP Shack-Hartmann" {
                    n321 = Unbundle By Name(w1257) -> ("x"=w1256:dbl)
                    n322 = call "pattern_hcp_shack_hartmann.vi"("Width"=w1256, "Reference Array?"="Reference Array?", "Fraction of SLM"="Fraction of SLM", "N"="Spots across centre") -> ("Shack-Hartmann Spots"=w1258:T1[])  [unwired: 7 in]
                  }
                  frame "Rectangular Grid" {
                    n323 = call "patterns_rectangular_grid.vi"("spacing/m"="spacing/m", "N"="N") -> ("Spots"=w1264:T1[])
                  }
                }
                n324 = local write "Generate"(FALSE ("Generate")) -> ()
                n325 = case shown="True" w1227 {
                  tunnel: w1228 -> [w1240 w1244]
                  tunnel: w1226 -> [_ w1246]
                  tunnel: [w1240 w1242] -> w1238
                  frame False {
                  }
                  frame True {
                    n326 = call "find_centroid.vi"("Spots"=w1244) -> ("centroid"=w1245:cluster{"x":dbl, "y":dbl, "z":dbl}, "# selected"=→"# selected":i16)  [unwired: 3 in, 3 out]
                    n327 = Subtract(x=w1246, y=w1245) -> (x-y=w1243:cluster{"x":dbl, "y":dbl, "z":dbl})
                    n328 = for {
                      tunnel: w1244 -> [w1249] mode=indexing
                      tunnel: w1243 -> [w1248]
                      tunnel: [w1247] -> w1242 mode=indexing
                      n329 = call "extract_position.vi"("Spot"=w1249) -> ("Position"=w1250:cluster{"x":dbl, "y":dbl, "z":dbl})
                      n330 = Add(x=w1250, y=w1248) -> (x+y=w1251:cluster{"x":dbl, "y":dbl, "z":dbl})
                      n331 = call "replace_position.vi"("Position"=w1251, "Spot in"=w1249) -> ("Spot"=w1247:T1)  [unwired: 2 out]
                    }
                  }
                }
                "Last Pattern" <- w1238
                n332 = call "ensure_selection_matches_spots.vi"("Select All (default: no)"=TRUE ("Select All (default: true)"), "Spots"=w1238) -> ("Selection and Groups out"=w1236:T7[], "Spots (duplicate)"=w1237:T1[])  [unwired: 4 in]
              }
              event "Spots across centre", "Fraction of SLM", "Reference Array?", "N", "spacing/m", "Spots across centre": Value Change {
                n333 = event-data() -> ()  [unwired: 1 in, 1 out]
                n334 = local read "Last Pattern"() -> (w1266:T1[])
                n335 = Equal?(x=w1267, y=w1266) -> (x = y?=w1265:bool)
                n336 = case shown="True" w1265 {
                  selector: w1265 -> [_ w1269]
                  frame False {
                  }
                  frame True {
                    n337 = property on="Generate" class="Bool (strict)"("Val(Sgnl)"=w1269) -> ()  [unwired: 2 in, 2 out]
                  }
                }
              }
              event Timeout {
                n338 = event-data() -> ()  [unwired: 1 in, 1 out]
              }
              event "Optimise": Value Change {
                n339 = event-data() -> ()  [unwired: 1 in, 1 out]
                n340 = for {
                  N: "Iterations" -> [_]
                  tunnel: 203 ("Optimisation Resolution") -> [w1281]
                  shift-right: [w1282] -> w1274
                  shift-left: w1275 -> [w1283]
                  tunnel: "Fall-off/m" -> [w1278]
                  n341 = call "do_gsw_step.vi"("Optimisation Resolution"=w1281, "Sinc Zero"=w1278, "Spots In"=w1283) -> ("non-uniformity"=→"non-uniformity":dbl, "efficiency"=→"efficiency":dbl, "Spots Out"=w1282:T1[])  [unwired: 6 in]
                }
              }
              event "Reset Phase/Amplitude": Value Change {
                n342 = event-data() -> ()  [unwired: 1 in, 1 out]
                n343 = for {
                  tunnel: [w1289] -> w1285 mode=indexing
                  tunnel: w1284 -> [w1290] mode=indexing
                  n344 = Bundle By Name(cluster=w1290, "Phase"=0.0, "Amplitude Correction"=0.0) -> (w1289:T1)
                }
              }
            }
          }
          frame "Plugins" {
            # "The local variable ensures the references are  correct when they make it through to the \"close plugins\" block."
            # "This is the error from loading/unloading VIs on the front panel"
            n345 = control-ref of="Plugin Pnl"() -> (w1294:refnum<vi>)
            n346 = Wait (ms)(milliseconds to wait=u32 10) -> ()  [unwired: 1 out]
            n347 = feedback #8() -> (w1293:T3)
            n348 = feedback #9() -> (w1295:errorcluster)
            n349 = event shown="[1] \"Plugin:\": Value Change" {
              selector: _ -> [_ _ _]
              dyn-events: _ -> [_ _ _]
              timeout: 10 -> [_ _ _]
              tunnel: "Abort Plugin" -> [w1302 _ _]
              tunnel: "Plugin:" -> [w1307 _ w1323]
              tunnel: w1295 -> [w1306 w1321 w1325]
              tunnel: [w1305 w1316 w1324] -> w1296
              tunnel: [w1304 w1317 w1327] -> w1292
              tunnel: w1293 -> [w1308 w1318 w1326]
              tunnel: w1294 -> [_ w1319 _]
              event Timeout {
                n350 = event-data() -> ()  [unwired: 1 in, 2 out]
                n351 = Not(x=w1302) -> (.not. x?=w1303:bool)
                n352 = case shown="True" w1303 {
                  tunnel: w1308 -> [w1310 w1315]
                  tunnel: w1307 -> [_ w1314]
                  tunnel: w1306 -> [w1309 w1313]
                  tunnel: [w1309 w1312] -> w1305
                  tunnel: [w1310 w1311] -> w1304
                  frame False {
                  }
                  frame True {
                    n353 = call "plugins_run.vi"("Error In"=w1313, "Plugin Index"=w1314, "Plugins In"=w1315) -> ("Error Out"=w1312:errorcluster, "Plugins"=w1311:T3)  [unwired: 7 in]
                  }
                }
              }
              event "Plugin:": Value Change {
                n354 = event-data() -> ("NewVal"=w1320:u16)  [unwired: 1 in]
                n355 = call "plugins_switch.vi"("error in"=w1321, "Plugin Pnl"=w1319, "Plugin Index"=w1320, "Plugins In"=w1318) -> ("error out"=w1316:errorcluster, "Plugins Out"=w1317:T3)  [unwired: 4 in]
              }
              event "Abort Plugin": Value Change {
                n356 = event-data() -> ("NewVal"=w1322:bool)  [unwired: 1 in]
                n357 = case shown="True" w1322 {
                  tunnel: [w1329 w1334] -> w1327
                  tunnel: w1326 -> [w1329 w1333]
                  tunnel: w1325 -> [w1328 w1332]
                  tunnel: [w1328 w1331] -> w1324
                  tunnel: w1323 -> [_ w1330]
                  frame False {
                  }
                  frame True {
                    n358 = call "plugins_abort.vi"("Error In"=w1332, "Plugin Index"=w1330, "Plugins In"=w1333) -> ("Error Out"=w1331:errorcluster, "Plugins Out"=w1334:T3)  [unwired: 7 in]
                  }
                }
              }
            }
            n359 = feedback-in #8(w1292) -> ()
            n360 = feedback-in #9(w1296) -> ()
            n361 = local write "Plugins"(w1292) -> ()
          }
          frame "Video" {
            # "All the controls on this tab are in the bottom (camera) loop."
            n362 = Wait (ms)(milliseconds to wait=u32 10) -> ()  [unwired: 1 out]
            n363 = property on="Property Node" class="ImageControl"(reference=w1335) -> ("Image Information String"=→"Image Information":string)  [unwired: 1 in, 2 out]
          }
        }
        n364 = case shown="True" "Clear String" {
          frame False {
          }
          frame True {
            w688 = ""
            n365 = local write "Sequence Frames To Check"(w688) -> ()
            n366 = local write "String 2"(w688) -> ()
          }
        }
      }
      event "Tab": Value Change {
        w1343 = T20 [enum."Video", enum."Particle Tracking"] items=["Current Spot", "Rotate", "Spot Shape", "Patterns", "Plugins", "Video", "Particle Tracking", "Clamping", "Blank"]
        w1348 = refnum<vi> refnum  # Image
        # "This allows us to disable custom mouse-handling for certain tabs.  It can also be done from within the \"mouse down\" event case."
        n367 = event-data() -> ("NewVal"=w1344:T4)  [unwired: 1 in, 3 out]
        n368 = Equal?(x=w1343, y=w1344) -> (x = y?=w1342:bool[])
        n369 = Or Array Elements(Boolean array=w1342) -> (logical OR=w1341:bool)
        n370 = Not(x=w1341) -> (.not. x?=w1340:bool)
        n371 = Select(t=w1347, s=w1340, f=w1348) -> (s? t:f=w1349:refnum<vi>)
        n372 = register-events(reference=w1351, w1349, w1348, w1348, w1348) -> (reference out=w1350:refnum<event-registration>)  [unwired: 1 in, 1 out]
      }
      event Menu Selection (User) {
        n373 = event-data() -> ("ItemTag"=w1359:string, "MenuRef"=w1352:refnum<k9>)  [unwired: 1 in]
        n374 = case shown="\"ToggleSavingData\"" w1359 {
          tunnel: w1363 -> [w1367 w1377 w1386 w1400 w1419 w1423 w1426 w1433 w1440 w1442 w1445 w1474 w1500 w1521 w1532 w1543 w1546 w1548 w1553 w1556]
          tunnel: w1362 -> [w1366 w1376 w1385 w1409 w1418 w1422 w1424 w1431 w1439 w1441 w1444 w1473 w1499 w1520 w1531 w1542 w1545 w1549 w1554 w1555]
          tunnel: [w1367 w1377 w1386 w1400 w1417 w1420 w1426 w1433 w1440 w1442 w1445 w1474 w1500 w1521 w1532 w1543 w1546 w1548 w1553 w1556] -> w1361
          tunnel: [w1366 w1376 w1385 w1409 w1416 w1421 w1425 w1432 w1438 w1443 w1446 w1473 w1499 w1520 w1531 w1542 w1545 w1549 w1554 w1555] -> w1360
          tunnel: [_ _ _ _ TRUE _ _ _ _ _ _ _ _ _ _ _ _ _ _ _] -> w1354
          tunnel: w1353 -> [_ _ _ _ _ _ _ _ _ _ _ w1472 w1498 w1512 _ _ _ _ _ _]
          tunnel: w1352 -> [_ _ _ _ _ _ _ _ _ _ _ w1463 w1492 w1515 w1526 w1537 _ _ _ _]
          frame "ToggleSavingData" {
            # "Data is saved from the middle loop: look there for an explanation."
            n375 = local read "Save Video"() -> (w1365:bool)
            n376 = Not(x=w1365) -> (.not. x?=w1364:bool)
            n377 = local write "Save Video"(w1364) -> ()
          }
          frame "SaveStateToFile" {
            # "Save the current settings (i.e. the values of all the controls in VIs that have [Red Tweezers Save Settings] in their documentation string) to a file."
            n378 = call "File Dialog"("prompt"="Please select a location to save the settings", "button label"="Save", "default name"="red_tweezers_settings.xml", "pattern (all files)"="*.xml" ("pattern label"), "pattern label"="XML Settings Files") -> ("selected path"=w1375:path, "cancelled"=w1368:bool)  [unwired: 7 in, 2 out]
            n379 = Not(x=w1368) -> (.not. x?=w1369:bool)
            n380 = case shown="True" w1369 {
              tunnel: w1375 -> [_ w1379]
              frame False {
              }
              frame True {
                n381 = Path To String(path=w1379) -> (string=w1378:string)
                n382 = call "settings_save_to_file.vi"("XML File Path"=w1379) -> ()  [unwired: 11 in]
                n383 = call "settings_filename_to_registry.vi"("Last Used Settings File"=w1378) -> ()  [unwired: 11 in]
              }
            }
          }
          frame "SaveStateToCurrentFile" {
            # "As SaveStateToFile, but using the current file (i.e. Save not Save As...)."
            n384 = global read "red_tweezers_globals_INTERNAL_VOLATILE.vi" "Current Settings File"() -> (w1384:path)
            n385 = call <vilib>:"Check if File or Folder Exists.vi"("path"=w1384) -> ("file or folder exists?"=w1383:bool, "dup path"=w1382:path)  [unwired: 8 in, 1 out]
            n386 = case shown="True" w1383 {
              selector: w1383 -> [_ w1397]
              tunnel: w1382 -> [_ w1398]
              tunnel: [w1389 w1398] -> w1381
              tunnel: [w1390 w1397] -> w1380
              frame False {
                n387 = call "File Dialog3"("prompt"="Please select a location to save the settings", "button label"="Save", "default name"="red_tweezers_settings.xml", "pattern (all files)"="*.xml" ("pattern label"), "pattern label"="XML Settings Files") -> ("selected path"=w1389:path, "cancelled"=w1396:bool)  [unwired: 7 in, 2 out]
                n388 = Not(x=w1396) -> (.not. x?=w1390:bool)
              }
              frame True {
              }
            }
            n389 = case shown="True" w1380 {
              tunnel: w1381 -> [_ w1388]
              frame False {
              }
              frame True {
                n390 = Path To String(path=w1388) -> (string=w1387:string)
                n391 = call "settings_save_to_file.vi"("XML File Path"=w1388) -> ()  [unwired: 11 in]
                n392 = call "settings_filename_to_registry.vi"("Last Used Settings File"=w1387) -> ()  [unwired: 11 in]
              }
            }
          }
          frame "LoadStateFromFile" {
            # "Load a file, and use it to reset the values of all the front panel controls."
            # "We need to re-run the initialisation stuff in UDP sender after changing settings\n(for example, this synchronises the settings like camera pixel size with the\nrelevant global variable)"
            n393 = call "File Dialog2"("prompt"="Please select a settings file", "button label"="Open", "default name"="red_tweezers_settings.xml", "pattern (all files)"="*.xml" ("pattern label"), "pattern label"="XML Settings Files") -> ("selected path"=w1401:path, "cancelled"=w1408:bool)  [unwired: 7 in, 2 out]
            n394 = Not(x=w1408) -> (.not. x?=w1407:bool)
            n395 = case shown="False" w1407 {
              selector: w1407 -> [w1410 w1411]
              tunnel: w1401 -> [_ w1412]
              tunnel: [w1410 w1411] -> w1399
              frame False {
              }
              frame True {
                n396 = call "settings_load_from_file.vi"("XML File Path"=w1412) -> ()  [unwired: 9 in, 2 out]
                n397 = Path To String(path=w1412) -> (string=w1413:string)
                n398 = call "settings_filename_to_registry.vi"("Last Used Settings File"=w1413) -> ()  [unwired: 11 in]
              }
            }
            n399 = call "UDP Sender generic_2.vi"("re-initialise"=w1399, "Spots"=w1400) -> ()  [unwired: 1 in, 1 out]
          }
          frame "Undo" {
            # "This should get the last undo vector and replace the spots with it :)"
            n400 = call "red_tweezers_UNDO.vi"("Selection/Group"=w1418, "Undo/Store (store, False)"=TRUE, "Spots"=w1419) -> ("Selection/Group Out (Undo only)"=w1416:T7[], "Spots Out (Undo only)"=w1417:T1[])  [unwired: 7 in]
          }
          frame "Delete" {
            n401 = call "delete_selected_spots.vi"("Selection/Group 3"=w1422, "Spots 3"=w1423) -> ("Selection/Group 2"=w1421:T7[], "Spots 2"=w1420:T1[])  [unwired: 4 in]
          }
          frame "SelectAllSpots" {
            n402 = for {
              tunnel: w1424 -> [w1429] mode=indexing
              tunnel: [w1430] -> w1425 mode=indexing
              n403 = Unbundle(w1429) -> ("Group ID"=w1428:i32)  [unwired: 1 out]
              n404 = Bundle(cluster=w1429, "Group ID"=w1428, "Selected"=TRUE ("Label.Visible")) -> (w1430:T7)
            }
          }
          frame "SelectNoSpots" {
            n405 = for {
              tunnel: w1431 -> [w1436] mode=indexing
              tunnel: [w1437] -> w1432 mode=indexing
              n406 = Unbundle(w1436) -> ("Group ID"=w1435:i32)  [unwired: 1 out]
              n407 = Bundle(cluster=w1436, "Group ID"=w1435, "Selected"=FALSE ("Label.Visible")) -> (w1437:T7)
            }
          }
          frame "SelectSpecificSpots" {
            n408 = call "select_by_id.vi"("Selection/Group"=w1439, "Spots"=w1440) -> ("Selection/Group Out"=w1438:T7[])  [unwired: 9 in]
          }
          frame "Group" {
            # "Group the currently selected spots"
            n409 = call "group_selected_spots.vi"("Selection/Group 2"=w1441) -> ("Array"=w1443:T7[])
          }
          frame "Ungroup" {
            # "Ungroup the currently selected spots"
            n410 = for {
              tunnel: [w1450] -> w1446 mode=indexing
              tunnel: w1444 -> [w1449] mode=indexing
              tunnel: 0 -> [w1448]
              n411 = Unbundle(w1449) -> ("Selected"=w1451:bool)  [unwired: 1 out]
              n412 = case shown="False" w1451 {
                tunnel: [w1452 w1455] -> w1450
                tunnel: w1449 -> [w1452 w1454]
                tunnel: w1448 -> [_ w1453]
                frame False {
                }
                frame True {
                  n413 = Unbundle(w1454) -> ("Selected"=w1456:bool)  [unwired: 1 out]
                  n414 = Bundle(cluster=w1454, "Group ID"=w1453, "Selected"=w1456) -> (w1455:T7)
                }
              }
            }
          }
          frame "ZoomIn" {
            w1457 = "ZoomToFit" ("item tag")
            # "turn off \"zoom to fit\""
            n415 = property class="ImageControl"(reference=w1472) -> (reference out=w1466:refnum<vi>, "ZoomSingle"=w1471:cluster{"X":sgl, "Y":sgl}, "Image Center Position"=w1464:cluster{"X":u32, "Y":u32})  [unwired: 1 in, 1 out]
            n416 = Unbundle(w1471) -> ("X"=w1469:sgl)  [unwired: 1 out]
            n417 = Round To Nearest(number=w1469) -> (nearest integer value=w1465:sgl)
            n418 = Greater Than 0?(x=w1465) -> (x > 0?=w1470:bool)
            n419 = case shown="True" w1470 {
              tunnel: w1469 -> [w1479 w1482]
              tunnel: [w1478 w1480] -> w1468
              frame False {
                n420 = Reciprocal(x=w1479) -> (1/x=w1476:sgl)
                n421 = Round Toward +Infinity(x=w1476) -> (ceil(x): smallest int >= x=w1477:sgl)
                n422 = Decrement(x=w1477) -> (x-1=w1475:sgl)
                n423 = Reciprocal(x=w1475) -> (1/x=w1478:sgl)
              }
              frame True {
                n424 = Round Toward -Infinity(1:w1482) -> (0:w1481:sgl)
                n425 = Increment(x=w1481) -> (x+1=w1480:sgl)
              }
            }
            n426 = Bundle(w1468, w1468) -> (w1467:cluster{sgl, sgl})  [unwired: 1 in]
            n427 = property class="ImageControl"(reference=w1466, "ZoomSingle"=w1467, "Image Center Position"=w1464) -> ()  [unwired: 1 in, 2 out]
            n428 = Get Menu Item Info(7:w1457, 11:w1463) -> (1:w1460:bool, 2:w1461:string, 3:w1462:refnum<k9>, 6:w1459:T21)  [unwired: 1 in, 3 out]
            n429 = Set Menu Item Info(4:w1459, 6:FALSE ("checked"), 7:w1457, 9:w1460, 10:w1461, 11:w1462) -> ()  [unwired: 1 in, 2 out]
          }
          frame "ZoomOut" {
            w1486 = "ZoomToFit" ("item tag")
            # "turn off \"zoom to fit\""
            n430 = property class="ImageControl"(reference=w1498) -> (reference out=w1494:refnum<vi>, "ZoomSingle"=w1497:cluster{"X":sgl, "Y":sgl}, "Image Center Position"=w1493:cluster{"X":u32, "Y":u32})  [unwired: 1 in, 1 out]
            n431 = Unbundle(w1497) -> ("X"=w1483:sgl)  [unwired: 1 out]
            n432 = Greater?(x=w1483, y=1.0) -> (0:w1485:bool)
            n433 = case shown="False" w1485 {
              tunnel: w1483 -> [w1507 w1510]
              tunnel: [w1506 w1508] -> w1496
              frame False {
                n434 = Reciprocal(x=w1507) -> (1/x=w1504:sgl)
                n435 = Add(x=w1504, y=sgl 0.01 ("x")) -> (x+y=w1502:sgl)
                n436 = Round Toward -Infinity(1:w1502) -> (0:w1505:sgl)
                n437 = Increment(x=w1505) -> (x+1=w1503:sgl)
                n438 = Reciprocal(x=w1503) -> (1/x=w1506:sgl)
              }
              frame True {
                n439 = Round Toward +Infinity(x=w1510) -> (ceil(x): smallest int >= x=w1509:sgl)
                n440 = Decrement(x=w1509) -> (x-1=w1508:sgl)
              }
            }
            n441 = Bundle(w1496, w1496) -> (w1495:cluster{sgl, sgl})  [unwired: 1 in]
            n442 = property class="ImageControl"(reference=w1494, "ZoomSingle"=w1495, "Image Center Position"=w1493) -> ()  [unwired: 1 in, 2 out]
            n443 = Get Menu Item Info(7:w1486, 11:w1492) -> (1:w1489:bool, 2:w1490:string, 3:w1491:refnum<k9>, 6:w1488:T21)  [unwired: 1 in, 3 out]
            n444 = Set Menu Item Info(4:w1488, 6:FALSE ("checked"), 7:w1486, 9:w1489, 10:w1490, 11:w1491) -> ()  [unwired: 1 in, 2 out]
          }
          frame "ZoomToFit" {
            w1516 = "ZoomToFit" ("item tag")
            # "and make sure the image obeys the result"
            # "Toggle menu checkmark"
            n445 = Get Menu Item Info(7:w1516, 11:w1515) -> (1:w1514:bool, 2:w1518:string, 3:w1519:refnum<k9>, 4:w1513:bool, 6:w1517:T21)  [unwired: 1 in, 2 out]
            n446 = Not(x=w1513) -> (.not. x?=w1511:bool)
            n447 = Set Menu Item Info(4:w1517, 6:w1511, 7:w1516, 9:w1514, 10:w1518, 11:w1519) -> ()  [unwired: 1 in, 2 out]
            n448 = property class="ImageControl"(reference=w1512, "Zoom to Fit Mode"=w1511) -> ()  [unwired: 1 in, 2 out]
          }
          frame "ShowGrid" {
            w1527 = "ShowGrid" ("item tag")
            # "Toggle menu checkmark"
            n449 = Get Menu Item Info(7:w1527, 11:w1526) -> (1:w1525:bool, 2:w1529:string, 3:w1530:refnum<k9>, 4:w1524:bool, 6:w1528:T21)  [unwired: 1 in, 2 out]
            n450 = Not(x=w1524) -> (.not. x?=w1523:bool)
            n451 = Set Menu Item Info(4:w1528, 6:w1523, 7:w1527, 9:w1525, 10:w1529, 11:w1530) -> ()  [unwired: 1 in, 2 out]
            n452 = call "grid_and_guides.vi"("Boolean"=w1523, "Operation"=T13."Set grid visibility") -> ()  [unwired: 9 in, 1 out]
          }
          frame "ShowGuides" {
            w1538 = "ShowGuides" ("item tag")
            # "Toggle menu checkmark"
            n453 = Get Menu Item Info(7:w1538, 11:w1537) -> (1:w1536:bool, 2:w1540:string, 3:w1541:refnum<k9>, 4:w1535:bool, 6:w1539:T21)  [unwired: 1 in, 2 out]
            n454 = Not(x=w1535) -> (.not. x?=w1534:bool)
            n455 = Set Menu Item Info(4:w1539, 6:w1534, 7:w1538, 9:w1536, 10:w1540, 11:w1541) -> ()  [unwired: 1 in, 2 out]
            n456 = call "grid_and_guides.vi"("Boolean"=w1534, "Operation"=T13."Set guide visibility") -> ()  [unwired: 9 in, 1 out]
          }
          frame "ConfigureGridAndGuides" {
            n457 = call "grid_and_guides.vi"("Operation"=T13."Show front panel") -> ()  [unwired: 10 in, 1 out]
          }
          frame "ShowSettings" {
            n458 = call "UDP Sender generic_2.vi"("Show panel"=TRUE, "Spots"=w1548) -> ()  [unwired: 1 in, 1 out]
          }
          frame "CameraSettings" {
            n459 = global read "red_tweezers_globals_INTERNAL_VOLATILE.vi" "Current Camera VI"() -> (w1551:path)
            n460 = Open VI Reference(vi path=w1551) -> (vi reference=w1550:refnum<vi>)  [unwired: 5 in, 1 out]
            n461 = property class="VI"(reference=w1550, "Front Panel.Open"=TRUE ("Front Panel Window:Open")) -> ()  [unwired: 1 in, 2 out]
          }
          frame Default {
          }
        }
      }
      event Mouse Down? {
        # "We don't process clicks when the user is on the video tab, so that we can set ROIs."
        # "When the mouse button goes down over the image, we save where it went down, etc. and wait to see what happens next.  We also register to be told when the mouse leaves the control, goes up, or moves.  \"click\" or \"drag\" are only detected once the mouse moves or goes up."
        n462 = event-data() -> ("Coords"=w1571:T22, "Button"=w1566:u16, "Mods"=w1575:cluster{"Double Click":bool, "Menu Key":bool}, "PlatMods"=w1574:T23)  [unwired: 1 in]
        n463 = call "mouse_to_image_coords.vi"("Mouse Coords (screen/pane units)"=w1571, "Image Control"=w1567) -> ("Cursor is on Display Area"=w1565:bool, "Mouse Coords (image pixels)"=w1570:cluster{dbl, dbl})  [unwired: 4 in]
        n464 = disable-structure shown="Enabled" {
          disable-tunnel: w1566 -> [w1583 _]
          disable-tunnel: w1565 -> [w1581 w1584]
          disable-tunnel: [w1580 w1584] -> w1561
          frame Enabled {
            n465 = Equal?(x=u16 1, y=w1583) -> (x = y?=w1582:bool)
            n466 = And(x=w1581, y=w1582) -> (x .and. y?=w1580:bool)
          }
          frame Disabled {
            # "use other pane to allow right-clicking on image"
          }
        }
        n467 = local read "Tab"() -> (w1562:T4)
        n468 = Not Equal?(x=w1562, y=T14."Video" ("Tab")) -> (x != y?=w1560:bool)
        n469 = And(x=w1561, y=w1560) -> (x .and. y?=w1559:bool)
        n470 = case shown="False" w1559 {
          tunnel: w1578 -> [w1587 w1598]
          tunnel: [T10 {"Button Down"=FALSE, "Dragging"=FALSE, "Position (Image Pixels)"={"X"=0.0, "Y"=0.0}, "Previous Position (Image Pixels)"={"X"=0.0, "Y"=0.0}, "Button"=0, "Mods"={"Double Click"=FALSE, "Menu Key"=FALSE}, "PlatMods"={"Shift"=FALSE, "Ctrl"=FALSE, "Alt"=FALSE, "Cmd"=FALSE, "Opt"=FALSE}} w1597] -> w1577
          tunnel: [w1587 w1594] -> w1576
          tunnel: w1566 -> [_ w1593]
          tunnel: w1575 -> [_ w1592]
          tunnel: w1574 -> [_ w1591]
          tunnel: w1570 -> [_ w1590]
          tunnel: [FALSE TRUE] -> w1569
          tunnel: w1567 -> [_ w1588]
          frame False {
            # "If the user clicked on a scrollbar, ignore it and let LabVIEW handle it. (this keeps the scrollbars working)"
          }
          frame True {
            w1596 = FALSE  # Dragging
            w1595 = TRUE  # Button Down
            n471 = register-events(reference=w1598, w1588, w1588, w1588, w1588) -> (reference out=w1594:refnum<event-registration>)  [unwired: 1 in, 1 out]
            n472 = Bundle("Button Down"=w1595, "Dragging"=w1596, "Mouse Coords (image pixels)"=w1590, "Mouse Coords (image pixels)"=w1590, "Button"=w1593, "Mods"=w1592, "PlatMods"=w1591) -> (w1597:T24)  [unwired: 1 in]
          }
        }
        n473 = Array Size(array=w1557) -> (size(s)=w1558:i32)
        n474 = local write "# of Spots"(w1558) -> ()
        n475 = local write "Selection/Group"(w1557) -> ()
        n476 = event-data("Discard?"=w1569) -> ()  [unwired: 4 in, 1 out]
      }
      event Mouse Leave {
        w1605 = refnum<vi> refnum  # Dummy
        # "When the mouse leaves, we reset things."
        n477 = event-data() -> ()  [unwired: 1 in, 2 out]
        n478 = register-events(reference=w1606, w1604, w1605, w1605, w1605) -> (reference out=w1603:refnum<event-registration>)  [unwired: 1 in, 1 out]
      }
      event Mouse Up {
        w1625 = refnum<vi> refnum  # Dummy
        # "Double clicking adds a spot at the mouse position."
        # "deregister"
        # "If we get here the mouse has gone down and up again.  If we've not moved in between, we have a Click.\nEither way we're no longer interested in mouse leave/move/up events."
        n479 = event-data() -> ("Mods"=w1612:cluster{"Double Click":bool, "Menu Key":bool})  [unwired: 1 in, 5 out]
        n480 = Unbundle By Name(w1618) -> ("Dragging"=w1627:bool)
        n481 = Unbundle By Name(w1612) -> ("Double Click"=w1609:bool)
        n482 = Not(x=w1627) -> (.not. x?=w1626:bool)
        n483 = Not(x=w1614) -> (.not. x?=w1616:bool)
        n484 = And(x=w1626, y=w1616) -> (x .and. y?=w1610:bool)
        n485 = case shown="True" w1610 {
          tunnel: w1618 -> [_ w1633]
          tunnel: w1620 -> [w1628 w1632]
          tunnel: w1619 -> [w1629 w1635]
          tunnel: [w1629 w1634] -> w1621
          tunnel: w1609 -> [_ w1630]
          tunnel: [w1628 w1631] -> w1611
          frame False {
          }
          frame True {
            n486 = case shown="False" w1630 {
              tunnel: w1635 -> [w1642 w1692]
              tunnel: [w1640 w1698] -> w1634
              tunnel: w1632 -> [w1636 w1699]
              tunnel: w1633 -> [w1639 w1694]
              tunnel: [w1636 w1690] -> w1631
              frame False {
                w1646 = 400.0  # 20^2 px
                # "If the user clicked, determine which spots should be selected: if we've clicked a spot/group then select it.  Shift-clicking toggles selection for that spot, and leaves the rest of the selection unchanged."
                # "check we're close enough"
                # "find closest"
                n487 = Unbundle By Name(w1639) -> ("Position (Image Pixels)"=w1638:cluster{"X":dbl, "Y":dbl}, "PlatMods.Shift"=w1637:bool)
                n488 = for {
                  tunnel: [w1682] -> w1644 mode=indexing
                  tunnel: w1638 -> [w1681]
                  tunnel: w1636 -> [w1680] mode=indexing
                  # "calculate distances between mouse position and spot positions"
                  n489 = call "extract_position.vi"("Spot"=w1680) -> ("Position"=w1679:cluster{"x":dbl, "y":dbl, "z":dbl})
                  n490 = call "coords_real_to_image_currentview.vi"("Position (real coords)"=w1679) -> ("Position (pixels, relative to the top left of the image)"=w1678:cluster{dbl, dbl})  [unwired: 7 in, 1 out]
                  n491 = Subtract(x=w1678, y=w1681) -> (x-y=w1685:cluster{dbl, dbl})
                  n492 = Multiply(x=w1685, y=w1685) -> (x*y=w1684:cluster{dbl, dbl})
                  n493 = Cluster To Array(cluster=w1684) -> (array=w1683:dbl[])
                  n494 = Add Array Elements(numeric array=w1683) -> (sum=w1682:dbl)
                }
                n495 = Array Max & Min(array=w1644) -> (min value=w1645:dbl, min index (indices)=w1641:i32)  [unwired: 2 out]
                n496 = Less Or Equal?(x=w1645, y=w1646) -> (x <= y?=w1643:bool)
                n497 = case shown="True" w1643 {
                  tunnel: w1642 -> [w1647 w1654]
                  tunnel: w1641 -> [_ w1648]
                  tunnel: w1637 -> [_ w1650]
                  tunnel: [w1647 w1649] -> w1640
                  frame False {
                    # "If we didn't click a spot, do nothing."
                  }
                  frame True {
                    # "If the spot is in a group, act on all spots in that group, not just the spot we clicked."
                    # "This case statement toggles the selection of the spot/group we clicked, and leaves other spots unchanged if we're holding shift.  Otherwise, we select the spot/group that was clicked and deselect everything else."
                    n498 = stacked-sequence {
                      tunnel: w1648 -> [_ w1656]
                      frame #0 {
                        n499 = local read "Current Spot #"() -> (→"Prev Current Spot":dbl)
                      }
                      frame #1 {
                        "Current Spot #" <- w1656
                      }
                    }
                    n500 = Index Array(array=w1654, index=w1648) -> (element=w1653:T7)
                    n501 = Unbundle(w1653) -> ("Group ID"=w1651:i32)  [unwired: 1 out]
                    n502 = Greater Than 0?(x=w1651) -> (x > 0?=w1652:bool)
                    n503 = for {
                      tunnel: w1654 -> [w1667] mode=indexing
                      tunnel: w1652 -> [w1664]
                      tunnel: w1651 -> [w1663]
                      tunnel: w1648 -> [w1662]
                      tunnel: w1650 -> [w1660]
                      tunnel: [w1658] -> w1649 mode=indexing
                      i -> [w1661]
                      n504 = Unbundle(w1667) -> ("Group ID"=w1657:i32, "Selected"=w1665:bool)
                      n505 = case shown="True" w1664 {
                        tunnel: w1657 -> [_ w1671]
                        tunnel: [w1669 w1673] -> w1659
                        tunnel: w1663 -> [_ w1672]
                        tunnel: w1662 -> [w1670 _]
                        tunnel: w1661 -> [w1668 _]
                        frame False {
                          n506 = Equal?(x=w1668, y=w1670) -> (x = y?=w1669:bool)
                        }
                        frame True {
                          n507 = Equal?(x=w1671, y=w1672) -> (x = y?=w1673:bool)
                        }
                      }
                      n508 = case shown="True" w1660 {
                        tunnel: [w1674 w1675] -> w1666
                        tunnel: w1665 -> [_ w1676]
                        tunnel: w1659 -> [w1674 w1677]
                        frame False {
                        }
                        frame True {
                          n509 = Exclusive Or(1:w1677, 2:w1676) -> (0:w1675:bool)
                        }
                      }
                      n510 = Bundle("Group ID"=w1657, w1666) -> (w1658:cluster{"Group ID":i32, bool})  [unwired: 1 out]
                    }
                  }
                }
              }
              frame True {
                # "convert mouse position to real coords, and add a spot there."
                # "Double-click detected"
                n511 = Unbundle By Name(w1694) -> ("Position (Image Pixels)"=w1693:cluster{"X":dbl, "Y":dbl})
                n512 = for {
                  tunnel: w1692 -> [w1702] mode=indexing
                  tunnel: [w1701] -> w1691 mode=indexing
                  n513 = Bundle(cluster=w1702, "Selected"=FALSE) -> (w1701:T7)  [unwired: 1 in]
                }
                n514 = call "coords_image_to_real_currentimage.vi"("Position (pixels on image)"=w1693) -> ("Position (real coords)"=w1695:cluster{dbl, dbl, "Z":dbl})  [unwired: 9 in]
                n515 = call "replace_position.vi"("Position"=w1695) -> ("Spot"=w1697:T1)  [unwired: 3 in]
                n516 = Build Array (concatenate)(w1699, w1697) -> (w1690:T1[])
                n517 = Build Array (concatenate)(w1691, T7 {"Group ID"=0, "Selected"=TRUE} ("selection_element")) -> (w1698:T7[])
                n518 = Array Size(array=w1690) -> (size(s)=w1689:i32)
                n519 = local write "Induce check"(TRUE) -> ()
                n520 = Subtract(x=w1689, y=1) -> (x-y=w1688:i32)
                n521 = local write "Current Spot #"(w1688) -> ()
              }
            }
          }
        }
        n522 = register-events(reference=w1623, w1622, w1625, w1625, w1625) -> (reference out=w1624:refnum<event-registration>)  [unwired: 1 in, 1 out]
      }
      event Mouse Move {
        n523 = event-data() -> ("Coords"=w1717:T22)  [unwired: 1 in, 2 out]
        n524 = call "mouse_to_image_coords.vi"("Mouse Coords (screen/pane units)"=w1717, "Image Control"=w1716) -> ("Mouse Coords (image pixels)"=w1708:cluster{dbl, dbl})  [unwired: 4 in, 1 out]
        n525 = Not(x=w1707) -> (.not. x?=w1712:bool)
        n526 = case shown="True" w1712 {
          tunnel: w1710 -> [_ w1730]
          tunnel: w1715 -> [w1722 w1732]
          tunnel: w1714 -> [w1721 w1731]
          tunnel: [w1721 w1731] -> w1703
          tunnel: [w1722 w1733] -> w1713
          tunnel: w1708 -> [_ w1724]
          tunnel: w1704 -> [_ w1723]
          frame False {
          }
          frame True {
            # "this is the displacement of the mouse, since the last iteration, in \"real\" coordinates (NB the conversions go before subtracting, as it may involve adding a constant as well as multiplying, which would confuse things as we're only interested in displacements here."
            # "The \"position\" local variable is there just in case we're on the \"current spot\" tab, so that the position updates nicely"
            # "If the user is dragging, translate the spots.\nHolding down shift causes the mouse's motion to be transformed into scaling about the centroid of the spots and rotation about the same point"
            n527 = Unbundle By Name(w1730) -> ("Position (Image Pixels)"=w1725:cluster{"X":dbl, "Y":dbl})
            n528 = call "find_centroid.vi"("Selection and Groups"=w1731, "Spots"=w1732) -> ("centroid"=w1726:cluster{"x":dbl, "y":dbl, "z":dbl})  [unwired: 2 in, 4 out]
            n529 = Unbundle By Name(w1730) -> ("PlatMods.Shift"=w1729:bool)
            n530 = disable-structure shown="Disabled" {
              disable-tunnel: w1726 -> [w1734 _]
              frame Disabled {
                n531 = local write "Position"(w1734) -> ()
              }
              frame Enabled {
              }
            }
            n532 = call "coords_image_to_real_currentimage.vi"("Position (pixels on image)"=w1724) -> ("Position (real coords)"=w1727:cluster{dbl, dbl, "Z":dbl})  [unwired: 9 in]
            n533 = call "coords_image_to_real_currentimage.vi"("Position (pixels on image)"=w1725) -> ("Position (real coords)"=w1728:cluster{dbl, dbl, "Z":dbl})  [unwired: 9 in]
            n534 = case shown="False" w1729 {
              tunnel: [w1739 w2013] -> w1733
              tunnel: w1732 -> [w1745 w2014]
              tunnel: w1731 -> [w1744 w2012]
              tunnel: w1728 -> [w1743 w1999]
              tunnel: w1726 -> [_ w2009]
              tunnel: w1727 -> [w1740 w2000]
              tunnel: w1723 -> [_ _]
              frame False {
                # "Spot Checker passes on information for the bubble collision,system so proper calculations can be made."
                n535 = while {
                  tunnel: w1743 -> [w1784]
                  tunnel: [w1774] -> w1741
                  tunnel: w1740 -> [w1773]
                  i -> [w1767]
                  stop <- w1769 stop-if-true
                  w1759 = 0
                  # "This while loop statement makes sure\nthat every spot gets checked before \nallowing any spot to move."
                  # "Buffer zone controls the amount of space between the\ncenter of a spot compared to the center of another spot.\nThis is used to prevent bubbles from colliding with each other."
                  # "Projected distance calculates the distance between two spots- this is used for when a \"hit\" occurs. If the projected distance becomes larger than the previous distance, the program will assume that the spot is being pulled from the buffer zone and as a result will allow the bubble to exit."
                  # "This subVI leads to the distance function, which outputs the distance between a spot being checked compared to the current spot number."
                  n536 = control-ref of="Value Check"() -> (w1764:refnum<vi>)
                  n537 = control-ref of="ID num check"() -> (w1763:refnum<vi>)
                  n538 = control-ref of="Spot Checker"() -> (w1780:refnum<vi>)
                  n539 = Subtract(x=w1773, y=w1784) -> (x-y=w1774:cluster{dbl, dbl, "Z":dbl})
                  n540 = call "DistanceFunction.vi"("Condition Driver"=FALSE, "Position (real coords)"=w1784, "Current Spot Number"=w1763, "Spot Checker"=w1780, "Spot Number Being Checked"=w1764) -> ("Distance"=w1748:dbl)  [unwired: 6 in]
                  n541 = stacked-sequence {
                    tunnel: w1748 -> [_ w1789]
                    frame #0 {
                      n542 = local read "Distance"() -> (→"Previous Distance":dbl)
                    }
                    frame #1 {
                      "Distance" <- w1789
                    }
                  }
                  n543 = Unbundle(w1774) -> (→"X Displacement":dbl, →"Y Displacement":dbl)  [unwired: 1 out]
                  n544 = control-ref of="ID num check"() -> (w1765:refnum<vi>)
                  n545 = control-ref of="Spot Checker"() -> (w1778:refnum<vi>)
                  n546 = control-ref of="Y Displacement"() -> (w1776:refnum<vi>)
                  n547 = control-ref of="Value Check"() -> (w1766:refnum<vi>)
                  n548 = control-ref of="X Displacement"() -> (w1777:refnum<vi>)
                  n549 = call "ProjectedDistance.vi"("X Displacement"=w1777, "Spot Number Check"=w1766, "Current Spot #"=w1765, "Spot Checker"=w1778, "Y Displacement"=w1776) -> ("Numeric"=→"Projected Distance":dbl)  [unwired: 6 in]
                  n550 = Multiply(x="Buffer Zone", y=2) -> (x*y=w1783:dbl)
                  n551 = local read "ID num check"() -> (w1760:dbl)
                  n552 = local read "Value Check"() -> (w1761:dbl)
                  n553 = local read "Projected Distance"() -> (w1752:dbl)
                  n554 = Equal?(x=w1748, y=0) -> (x = y?=w1749:bool)
                  n555 = case shown="False" w1749 {
                    frame False {
                      n556 = local read "Hit"() -> (w1786:bool)
                      n557 = local write "Hit Indicator"(w1786) -> ()
                    }
                    frame True {
                      "Hit Indicator" <- FALSE
                    }
                  }
                  n558 = Not Equal?(x=w1752, y=0) -> (x != y?=w1750:bool)
                  n559 = Less Or Equal?(x=w1748, y=w1783) -> (x <= y?=w1753:bool)
                  n560 = Equal?(x=w1760, y=w1759) -> (x = y?=w1758:bool)
                  n561 = And(x=w1753, y=w1750) -> (x .and. y?=w1746:bool)
                  "Hit" <- w1746
                  n562 = Equal?(x=w1759, y=w1761) -> (x = y?=w1757:bool)
                  n563 = Not(x=w1746) -> ()  [unwired: 1 out]
                  n564 = And(x=w1758, y=w1757) -> (x .and. y?=w1756:bool)
                  n565 = Or(x=w1746, y=w1756) -> (x .or. y?=w1762:bool)
                  n566 = case shown="True" w1762 {
                    frame False {
                      n567 = stacked-sequence {
                        frame #0 {
                          n568 = local read "Potential Collisions"() -> (w1792:dbl)
                          n569 = local read "Spot # Check"() -> (w1794:dbl)
                          n570 = Subtract(x=w1792, y=1) -> (x-y=w1790:dbl)
                          n571 = Less Or Equal?(x=w1794, y=w1790) -> (x <= y?=w1793:bool)
                          n572 = case shown="True" w1793 {
                            frame False {
                              # "Spot # Check resets if the the number of potential collisons is more than Spot # Check."
                              n573 = local write "Spot # Check"(0) -> ()
                            }
                            frame True {
                              n574 = stacked-sequence {
                                frame #0 {
                                # "Spot # Check increments by 1 every time it is greater than the # of potential collisions."
                                n575 = local read "Spot # Check"() -> (w1798:dbl)
                                n576 = Add(x=w1798, y=1) -> (x+y=→"Spot # Check":dbl)
                                }
                                frame #1 {
                                # "Spot # Check resets if the Spot # Check is eqaul to the # of potential collisions."
                                n577 = local read "Potential Collisions"() -> (w1799:dbl)
                                n578 = local read "Spot # Check"() -> (w1800:dbl)
                                n579 = Equal?(x=w1800, y=w1799) -> (x = y?=w1801:bool)
                                n580 = case shown="True" w1801 {
                                frame False {
                                }
                                frame True {
                                n581 = local write "Spot # Check"(0) -> ()
                                }
                                }
                                }
                                frame #2 {
                                n582 = local read "Spot Checker"() -> (w1816:T1[])
                                n583 = local read "Current Spot #"() -> (w1817:dbl)
                                n584 = local read "Area to check"() -> (w1803:dbl)
                                n585 = Index Array(array=w1816, index=w1817) -> (element=w1815:T1)
                                n586 = local read "Orig Y SC"() -> (w1812:dbl)
                                n587 = Unbundle By Name(w1815) -> ("Position.x"=w1813:dbl, "Position.y"=w1811:dbl)
                                n588 = local read "Orig X SC"() -> (w1814:dbl)
                                n589 = Subtract(x=w1811, y=w1812) -> (x-y=w1804:dbl)
                                n590 = Absolute Value(x=w1804) -> (abs(x)=w1805:dbl)
                                n591 = Subtract(x=w1813, y=w1814) -> (x-y=w1807:dbl)
                                n592 = Greater?(x=w1805, y=w1803) -> (0:w1809:bool)
                                n593 = Absolute Value(x=w1807) -> (abs(x)=w1806:dbl)
                                n594 = Greater?(x=w1806, y=w1803) -> (0:w1808:bool)
                                n595 = Or(x=w1808, y=w1809) -> (x .or. y?=w1810:bool)
                                n596 = case shown="True" w1810 {
                                frame False {
                                }
                                frame True {
                                n597 = stacked-sequence {
                                frame #0 {
                                n598 = local read "Null array"() -> (w1822:dbl[])
                                n599 = local write "What to Check"(w1822) -> ()
                                n600 = local write "ID"(w1822) -> ()
                                n601 = local read "Current Spot #"() -> (w1824:dbl)
                                n602 = local write "Potential Collisions"(0) -> ()
                                n603 = local read "Spot Checker"() -> (w1823:T1[])
                                n604 = Index Array(array=w1823, index=w1824) -> (element=w1825:T1)
                                n605 = Wait (ms)(milliseconds to wait=100) -> ()  [unwired: 1 out]
                                n606 = Unbundle By Name(w1825) -> ("Position.x"=w1819:dbl, "Position.y"=w1820:dbl)
                                n607 = local write "Orig Y SC"(w1820) -> ()
                                n608 = local write "Orig X SC"(w1819) -> ()
                                }
                                frame #1 {
                                # "All this is a  statement checking whether the microrobot is within the area being checked using absolute value statements. The number of potential collisions gets added by 1 every time a bubble is detected within the area."
                                n609 = local read "# of Spots"() -> (w1826:dbl)
                                n610 = for {
                                N: w1826 -> [_]
                                tunnel: w1826 -> [w1831]
                                i -> [w1827]
                                n611 = local read "Selection/Group"() -> (w1830:T7[])
                                n612 = Index Array(array=w1830, index=w1827) -> (element=w1829:T7)
                                n613 = Unbundle By Name(w1829) -> ("Selected"=w1828:bool)
                                n614 = case shown="True" w1828 {
                                tunnel: w1831 -> [_ w1833]
                                tunnel: w1827 -> [_ w1832]
                                frame False {
                                }
                                frame True {
                                n615 = for {
                                N: w1833 -> [_]
                                tunnel: w1832 -> [w1834]
                                i -> [w1835]
                                n616 = local read "Selection/Group"() -> (w1839:T7[])
                                n617 = Index Array(array=w1839, index=w1835) -> (element=w1838:T7)
                                n618 = Unbundle By Name(w1838) -> ("Selected"=w1836:bool)
                                n619 = Not(x=w1836) -> (.not. x?=w1837:bool)
                                n620 = case shown="True" w1837 {
                                tunnel: w1835 -> [_ w1843]
                                tunnel: w1834 -> [_ w1842]
                                tunnel: w1834 -> [_ w1841]
                                frame False {
                                }
                                frame True {
                                n621 = local read "Spot Checker"() -> (w1860:T1[])
                                n622 = Index Array(array=w1860, index=w1843) -> (element=w1861:T1)
                                n623 = Index Array(array=w1860, index=w1842) -> (element=w1859:T1)
                                n624 = Unbundle By Name(w1859) -> ("Position.x"=w1856:dbl, "Position.y"=w1852:dbl)
                                n625 = Unbundle By Name(w1861) -> ("Position.x"=w1853:dbl, "Position.y"=w1849:dbl)
                                n626 = local read "Area+ Buffer"() -> (w1840:dbl)
                                n627 = Subtract(x=w1856, y=w1840) -> (x-y=w1857:dbl)
                                n628 = Greater Or Equal?(x=w1853, y=w1857) -> (x >= y?=w1858:bool)
                                n629 = Add(x=w1852, y=w1840) -> (x+y=w1851:dbl)
                                n630 = Subtract(x=w1852, y=w1840) -> (x-y=w1850:dbl)
                                n631 = Add(x=w1856, y=w1840) -> (x+y=w1854:dbl)
                                n632 = Less Or Equal?(x=w1849, y=w1851) -> (x <= y?=w1848:bool)
                                n633 = Greater Or Equal?(x=w1849, y=w1850) -> (x >= y?=w1847:bool)
                                n634 = Less Or Equal?(x=w1853, y=w1854) -> (x <= y?=w1855:bool)
                                n635 = And(x=w1858, y=w1855) -> (x .and. y?=w1845:bool)
                                n636 = And(x=w1848, y=w1847) -> (x .and. y?=w1846:bool)
                                n637 = And(x=w1845, y=w1846) -> (x .and. y?=w1844:bool)
                                n638 = case shown="True" w1844 {
                                tunnel: w1843 -> [_ _]
                                tunnel: w1843 -> [_ w1863]
                                tunnel: w1841 -> [_ w1862]
                                frame False {
                                }
                                frame True {
                                n639 = stacked-sequence {
                                tunnel: w1863 -> [w1864 _]
                                tunnel: w1862 -> [w1865 _]
                                frame #0 {
                                n640 = local read "Potential Collisions"() -> (w1868:dbl)
                                n641 = local read "What to Check"() -> (w1869:dbl[])
                                n642 = Insert Into Array(array=w1869, index=w1868, new element=w1864) -> (w1870:dbl[])
                                n643 = local read "ID"() -> (w1867:dbl[])
                                n644 = local write "What to Check"(w1870) -> ()
                                n645 = Insert Into Array(array=w1867, index=w1868, new element=w1865) -> (w1866:dbl[])
                                n646 = local write "ID"(w1866) -> ()
                                }
                                frame #1 {
                                n647 = local read "Potential Collisions"() -> (w1873:dbl)
                                n648 = Add(x=w1873, y=1) -> (x+y=w1871:dbl)
                                n649 = local write "Potential Collisions"(w1871) -> ()
                                }
                                }
                                }
                                }
                                }
                                }
                                }
                                }
                                }
                                }
                                }
                                frame #2 {
                                n650 = local read "Current Spot #"() -> (w1874:dbl)
                                n651 = local write "Prev Current Spot"(w1874) -> ()
                                }
                                }
                                }
                                }
                                }
                              }
                            }
                          }
                        }
                        frame #1 {
                          # "This updates the ID and Value being checked at the beginning of IDs and values being checked."
                          n652 = local read "Spot # Check"() -> (w1877:dbl)
                          n653 = local read "What to Check"() -> (w1878:dbl[])
                          n654 = local read "ID"() -> (w1879:dbl[])
                          n655 = Index Array(array=w1879, index=w1877) -> (element=w1876:dbl)
                          n656 = Index Array(array=w1878, index=w1877) -> (element=w1875:dbl)
                          n657 = local write "Value Check"(w1875) -> ()
                          n658 = local write "ID num check"(w1876) -> ()
                        }
                      }
                    }
                    frame True {
                      n659 = stacked-sequence {
                        frame #0 {
                          # "This section activate a case statement which allows us to change the area being checked. Orig X/Y SC holds the position of the area to check and changes after the bubble exits the area beig checked."
                          # "This statement controls the areas selected and finds which bubbles needs to be checked. This activates when the bubble\nmoves out of the area specified."
                          n660 = local read "# of Spots"() -> (w1899:dbl)
                          n661 = local read "Current Spot #"() -> (w1898:dbl)
                          n662 = Subtract(x=w1899, y=1) -> (x-y=w1900:dbl)
                          n663 = Equal?(x=w1898, y=w1900) -> (x = y?=w1896:bool)
                          n664 = case shown="True" w1896 {
                            tunnel: [w1959 w1962] -> w1897
                            frame True {
                              n665 = local read "# of Spots"() -> (w1960:dbl)
                              n666 = Subtract(x=w1960, y=2) -> (x-y=w1959:dbl)
                            }
                            frame False {
                              n667 = local read "# of Spots"() -> (w1961:dbl)
                              n668 = Subtract(x=w1961, y=1) -> (x-y=w1962:dbl)
                            }
                          }
                          "Maximum" <- w1897
                          n669 = local read "Spot Checker"() -> (w1895:T1[])
                          n670 = local read "Current Spot #"() -> (w1894:dbl)
                          n671 = Index Array(array=w1895, index=w1894) -> (element=w1893:T1)
                          n672 = Unbundle By Name(w1893) -> ("Position.x"=w1892:dbl, "Position.y"=w1891:dbl)
                          n673 = local read "Orig Y SC"() -> (w1889:dbl)
                          n674 = local read "Orig X SC"() -> (w1890:dbl)
                          n675 = Subtract(x=w1891, y=w1889) -> (x-y=w1886:dbl)
                          n676 = Subtract(x=w1892, y=w1890) -> (x-y=w1888:dbl)
                          n677 = Absolute Value(x=w1886) -> (abs(x)=w1885:dbl)
                          n678 = Absolute Value(x=w1888) -> (abs(x)=w1887:dbl)
                          n679 = local read "Area to check"() -> (w1881:dbl)
                          n680 = local read "Area to check"() -> (w1880:dbl)
                          n681 = Greater?(x=w1887, y=w1881) -> (0:w1884:bool)
                          n682 = Greater?(x=w1885, y=w1880) -> (0:w1883:bool)
                          n683 = Or(x=w1884, y=w1883) -> (x .or. y?=w1882:bool)
                          n684 = case shown="True" w1882 {
                            frame False {
                            }
                            frame True {
                              n685 = stacked-sequence {
                                frame #0 {
                                # "A small time delay of 100 ms is provided to allow the data to pass throguh properly."
                                n686 = Wait (ms)(milliseconds to wait=100) -> ()  [unwired: 1 out]
                                n687 = local read "Null array"() -> (→"What to Check" →"ID":dbl[])
                                n688 = local read "Spot Checker"() -> (w1907:T1[])
                                n689 = local read "Current Spot #"() -> (w1906:dbl)
                                n690 = Index Array(array=w1907, index=w1906) -> (element=w1905:T1)
                                n691 = Unbundle By Name(w1905) -> ("Position.x"=→"Orig X SC":dbl, "Position.y"=→"Orig Y SC":dbl)
                                "Potential Collisions" <- 0
                                }
                                frame #1 {
                                n692 = local read "# of Spots"() -> (w1910:dbl)
                                n693 = for {
                                N: w1910 -> [_]
                                tunnel: w1910 -> [w1915]
                                i -> [w1911]
                                n694 = local read "Selection/Group"() -> (w1914:T7[])
                                n695 = Index Array(array=w1914, index=w1911) -> (element=w1913:T7)
                                n696 = Unbundle By Name(w1913) -> ("Selected"=w1912:bool)
                                n697 = case shown="True" w1912 {
                                tunnel: w1915 -> [_ w1917]
                                tunnel: w1911 -> [_ w1916]
                                frame False {
                                }
                                frame True {
                                n698 = for {
                                N: w1917 -> [_]
                                tunnel: w1916 -> [w1918]
                                i -> [w1919]
                                n699 = local read "Selection/Group"() -> (w1923:T7[])
                                n700 = Index Array(array=w1923, index=w1919) -> (element=w1922:T7)
                                n701 = Unbundle By Name(w1922) -> ("Selected"=w1920:bool)
                                n702 = Not(x=w1920) -> (.not. x?=w1921:bool)
                                n703 = case shown="True" w1921 {
                                tunnel: w1919 -> [_ w1927]
                                tunnel: w1918 -> [_ w1926]
                                tunnel: w1918 -> [_ w1925]
                                frame False {
                                }
                                frame True {
                                n704 = local read "Spot Checker"() -> (w1944:T1[])
                                n705 = Index Array(array=w1944, index=w1927) -> (element=w1945:T1)
                                n706 = Index Array(array=w1944, index=w1926) -> (element=w1943:T1)
                                n707 = Unbundle By Name(w1943) -> ("Position.x"=w1940:dbl, "Position.y"=w1936:dbl)
                                n708 = Unbundle By Name(w1945) -> ("Position.x"=w1937:dbl, "Position.y"=w1933:dbl)
                                n709 = local read "Area+ Buffer"() -> (w1924:dbl)
                                n710 = Subtract(x=w1940, y=w1924) -> (x-y=w1941:dbl)
                                n711 = Greater Or Equal?(x=w1937, y=w1941) -> (x >= y?=w1942:bool)
                                n712 = Add(x=w1936, y=w1924) -> (x+y=w1935:dbl)
                                n713 = Subtract(x=w1936, y=w1924) -> (x-y=w1934:dbl)
                                n714 = Add(x=w1940, y=w1924) -> (x+y=w1938:dbl)
                                n715 = Less Or Equal?(x=w1933, y=w1935) -> (x <= y?=w1932:bool)
                                n716 = Greater Or Equal?(x=w1933, y=w1934) -> (x >= y?=w1931:bool)
                                n717 = Less Or Equal?(x=w1937, y=w1938) -> (x <= y?=w1939:bool)
                                n718 = And(x=w1942, y=w1939) -> (x .and. y?=w1929:bool)
                                n719 = And(x=w1932, y=w1931) -> (x .and. y?=w1930:bool)
                                n720 = And(x=w1929, y=w1930) -> (x .and. y?=w1928:bool)
                                n721 = case shown="True" w1928 {
                                tunnel: w1927 -> [_ _]
                                tunnel: w1927 -> [_ w1947]
                                tunnel: w1925 -> [_ w1946]
                                frame False {
                                }
                                frame True {
                                n722 = stacked-sequence {
                                tunnel: w1947 -> [w1948 _]
                                tunnel: w1946 -> [w1949 _]
                                frame #0 {
                                n723 = local read "Potential Collisions"() -> (w1952:dbl)
                                n724 = local read "What to Check"() -> (w1953:dbl[])
                                n725 = Insert Into Array(array=w1953, index=w1952, new element=w1948) -> (w1954:dbl[])
                                n726 = local read "ID"() -> (w1951:dbl[])
                                n727 = Insert Into Array(array=w1951, index=w1952, new element=w1949) -> (w1950:dbl[])
                                n728 = local write "What to Check"(w1954) -> ()
                                n729 = local write "ID"(w1950) -> ()
                                }
                                frame #1 {
                                n730 = local read "Potential Collisions"() -> (w1957:dbl)
                                n731 = Add(x=w1957, y=1) -> (x+y=w1955:dbl)
                                n732 = local write "Potential Collisions"(w1955) -> ()
                                }
                                }
                                }
                                }
                                }
                                }
                                }
                                }
                                }
                                }
                                }
                              }
                            }
                          }
                        }
                        frame #1 {
                          n733 = local read "# of Spots"() -> (w1966:dbl)
                          n734 = Not Equal?(x=w1966, y=1) -> (x != y?=w1964:bool)
                          n735 = case shown="True" w1964 {
                            frame False {
                            }
                            frame True {
                              n736 = stacked-sequence {
                                frame #0 {
                                n737 = local read "Potential Collisions"() -> (w1969:dbl)
                                n738 = local read "Spot # Check"() -> (w1971:dbl)
                                n739 = Subtract(x=w1969, y=1) -> (x-y=w1967:dbl)
                                n740 = Less Or Equal?(x=w1971, y=w1967) -> (x <= y?=w1970:bool)
                                n741 = case shown="False" w1970 {
                                frame False {
                                n742 = local write "Spot # Check"(0) -> ()
                                }
                                frame True {
                                }
                                }
                                }
                                frame #1 {
                                n743 = local read "What to Check"() -> (w1977:dbl[])
                                n744 = local read "ID"() -> (w1975:dbl[])
                                n745 = local read "Spot # Check"() -> (w1973:dbl)
                                n746 = Index Array(array=w1977, index=w1973) -> (element=→"Value Check":dbl)
                                n747 = Index Array(array=w1975, index=w1973) -> (element=→"ID num check":dbl)
                                }
                              }
                            }
                          }
                        }
                      }
                    }
                  }
                  n748 = local read "Potential Collisions"() -> (w1754:dbl)
                  n749 = Subtract(x=w1754, y=1) -> (x-y=w1755:dbl)
                  n750 = local read "Hit"() -> (w1772:bool)
                  n751 = Equal?(x=w1767, y=w1755) -> (x = y?=w1771:bool)
                  n752 = Or(x=w1772, y=w1771) -> (x .or. y?=w1769:bool)
                }
                n753 = for {
                  tunnel: w1744 -> [w1991] mode=indexing
                  tunnel: w1745 -> [w1988] mode=indexing
                  tunnel: [w1990] -> w1739 mode=indexing
                  tunnel: w1741 -> [w1989]
                  # "If the projected distance is greater than the\nprevious distance, then the selected spots will move. \nThis situation only occurs if the bubble is about to/crossing \nthe buffer zone of another bubble. \n\nThe selected spots will also move if none of the bubbles\nare near/crossing the buffer zone of another bubble."
                  n754 = local read "Hit"() -> (w1981:bool)
                  n755 = Unbundle By Name(w1988) -> ()  [unwired: 1 out]
                  n756 = local read "Projected Distance"() -> (w1980:dbl)
                  n757 = Unbundle(w1991) -> ("Group ID"=→"Group ID #":i32, "Selected"=w1985:bool)
                  n758 = local read "Previous Distance"() -> (w1983:dbl)
                  n759 = Not(x=w1981) -> (.not. x?=w1979:bool)
                  n760 = Greater?(x=w1980, y=w1983) -> (0:w1982:bool)
                  n761 = And(x=w1981, y=w1982) -> (x .and. y?=w1978:bool)
                  n762 = Or(x=w1979, y=w1978) -> (x .or. y?=w1984:bool)
                  n763 = And(x=w1985, y=w1984) -> (x .and. y?=w1986:bool)
                  n764 = case shown="True" w1986 {
                    tunnel: w1988 -> [w1992 w1996]
                    tunnel: [w1992 w1995] -> w1990
                    tunnel: w1989 -> [_ w1997]
                    frame False {
                      # "otherwise, leave it alone!"
                    }
                    frame True {
                      # "If the spot is selected, move it by the same amount as the mouse"
                      n765 = call "extract_position.vi"("Spot"=w1996) -> ("Position"=w1994:cluster{"x":dbl, "y":dbl, "z":dbl})
                      n766 = Add(x=w1994, y=w1997) -> (x+y=w1993:cluster{dbl, dbl, dbl})
                      n767 = call "replace_position.vi"("Position"=w1993, "Spot in"=w1996) -> ("Spot"=w1995:T1)  [unwired: 2 out]
                    }
                  }
                }
                "Spot Checker" <- w1739
                n768 = local read "Locked Current Spot"() -> (w1735:dbl)
                n769 = Index Array(array=w1739, index=w1735) -> (element=w1738:T1)
                n770 = Unbundle By Name(w1738) -> ("Position.x"=→"New X":dbl, "Position.y"=→"New Y":dbl)  [unwired: 1 out]
                n771 = Array Size(array=w1739) -> (size(s)=→"# of Spots":i32)
              }
              frame True {
                # "coordinate conversion to find the rotation and scaling done by the mouse, about the centroid of the spots"
                n772 = Subtract(x=w1999, y=w2009) -> (x-y=w2018:cluster{dbl, dbl, dbl})
                n773 = Subtract(x=w2000, y=w2009) -> (x-y=w2017:cluster{dbl, dbl, dbl})
                n774 = Unbundle(w2017) -> (w2003:dbl, w2004:dbl)  [unwired: 1 out]
                n775 = Unbundle(w2018) -> (w2008:dbl, w2007:dbl)  [unwired: 1 out]
                n776 = Re/Im To Polar(2:w2004, 3:w2003) -> (0:w2001:dbl, 1:w2002:dbl)
                n777 = Re/Im To Polar(2:w2007, 3:w2008) -> (0:w2005:dbl, 1:w2006:dbl)
                n778 = Divide(x=w2002, y=w2006) -> (x/y=w1998:dbl)
                n779 = Subtract(x=w2001, y=w2005) -> (x-y=w2010:dbl)
                n780 = Bundle(w1998, w1998, w1998) -> (w2020:cluster{dbl, dbl, dbl})  [unwired: 1 out]
                n781 = call "scale_matrix.vi"("Scale Factors"=w2020) -> ("Scale Matrix"=w2016:T18)
                n782 = call "arb_rotation_matrix.vi"("Unit Vector"=cluster{dbl, dbl, dbl} {0.0, 0.0, 1.0}, "theta"=w2010) -> ("Real Matrix"=w2015:T18)
                n783 = call-poly <vilib>:"A x B.vi"("B"=w2015, "A"=w2016) -> ("A x B"=w2011:T18)  [unwired: 1 out]
                n784 = for {
                  tunnel: w2014 -> [w2026] mode=indexing
                  tunnel: [w2025] -> w2013 mode=indexing
                  tunnel: w2012 -> [w2024] mode=indexing
                  tunnel: w2009 -> [w2022]
                  tunnel: w2011 -> [w2021]
                  n785 = Unbundle(w2024) -> ("Selected"=w2023:bool)  [unwired: 1 out]
                  n786 = case shown="True" w2023 {
                    tunnel: w2026 -> [w2027 w2031]
                    tunnel: [w2027 w2030] -> w2025
                    tunnel: w2022 -> [_ w2029]
                    tunnel: w2021 -> [_ w2028]
                    frame False {
                    }
                    frame True {
                      n787 = call "apply_matrix_transformation_to_spots.vi"("Transform centre (i.e. transform about this point)"=w2029, "Transformation Matrix (3x3)"=w2028, "Spot In"=w2031) -> ("Spot Out"=w2030:T1)  [unwired: 5 out]
                    }
                  }
                }
              }
            }
          }
        }
        "Selection/Group" <- w1703
        n788 = Unbundle By Name(w1710) -> ("Position (Image Pixels)"=w1709:cluster{"X":dbl, "Y":dbl})
        n789 = Bundle By Name(cluster=w1710, "Dragging"=TRUE, "Previous Position (Image Pixels)"=w1709, "Position (Image Pixels)"=w1708) -> (w1719:T10)
      }
      event "stop": Value Change {
        n790 = event-data() -> ()  [unwired: 1 in, 4 out]
        n791 = global read "red_tweezers_globals_INTERNAL_VOLATILE.vi" "Current Settings File"() -> (w2035:path)
        n792 = call <vilib>:"Check if File or Folder Exists.vi"("path"=w2035) -> ("file or folder exists?"=w2034:bool)  [unwired: 8 in, 2 out]
        n793 = case shown="False" w2034 {
          tunnel: [w2042 w2046] -> w2036
          frame False {
            n794 = Two Button Dialog(message="Save current settings?", 1:"Don't Save" ("F button name (\"Cancel\")"), 2:"Save As..." ("T button name (\"OK\")")) -> (T button?=w2039:bool)
            n795 = Select(t=T15."Center Button" ("Which Button?"), s=w2039, f=T15."Right Button" ("Which Button?")) -> (s? t:f=w2042:T15)
          }
          frame True {
            n796 = call <vilib>:"Three Button Dialog.vi"("Allow user to close window? (TRUE)"=TRUE, "Window Title (\"\")"="Save Settings?" ("Window Title (\"\")"), "Right Button Text (\"Cancel\")"="No" ("Right Button Text (\"Cancel\")"), "Center Button Text (\"No\")"="Save As..." ("Center Button Text (\"No\")"), "Left Button Text (\"Yes\")"="Save" ("Left Button Text (\"Yes\")"), "message"="Would you like to save the current settings? You can choose to use the current settings file or save to a new location.") -> ("Which Button?"=w2046:T15)  [unwired: 5 in]
          }
        }
        n797 = case shown="\"Center Button\"" w2036 {
          tunnel: [TRUE TRUE FALSE FALSE] -> w2033
          frame "Left Button", Default {
          }
          frame "Center Button" {
            n798 = call "File Dialog5"("prompt"="Please select a location to save the settings", "button label"="Save", "default name"="red_tweezers_settings.xml", "pattern (all files)"="*.xml" ("pattern label"), "pattern label"="XML Settings Files") -> ("selected path"=w2054:path)  [unwired: 7 in, 3 out]
            n799 = global write "red_tweezers_globals_INTERNAL_VOLATILE.vi" "Current Settings File"(w2054) -> ()
          }
          frame "Right Button" {
          }
          frame "Window Close" {
          }
        }
        n800 = global write "red_tweezers_globals_INTERNAL_VOLATILE.vi" "Save Settings On Exit"(w2033) -> ()
      }
    }
    n801 = call "IMAQ Create"("Image Name"="untitled", "Image Type"=w47) -> ("New Image"=w46:T8)  [unwired: 3 in, 1 out]
    n802 = call "Vision Acquisition"() -> ("Image Out"=w44:T8)  [unwired: 26 in, 1 out]
    n803 = local read "Number of Matches Returned"() -> (w37:dbl)
    n804 = case shown="True" "Camera Capture" {
      frame False {
      }
      frame True {
        n805 = local read "Circles"() -> (w149:T9)
        n806 = Index Array(array=w149) -> (element=w148:T25)  [unwired: 1 in]
        n807 = Unbundle(w148) -> ("Position"=w147:cluster{"X":sgl, "Y":sgl})  [unwired: 2 out]
        n808 = Unbundle(w147) -> ("X"=→"Bubble x":sgl, "Y"=→"Bubble y":sgl)
      }
    }
    n809 = Add(x=w37, y=1.0 ("x+y")) -> (x+y=w40:dbl)
    n810 = call "IMAQ ExtractSingleColorPlane"("Color Plane"=w43, "Image Dst"=w46, "Image Src"=w44) -> ("Image Dst Out"=w41:T8)  [unwired: 7 in, 1 out]
    n811 = for {
      N: w40 -> [_]
      tunnel: w41 -> [w286]
      tunnel: [w285] -> w39 mode=indexing
      i -> [w282]
      n812 = local read "Circles"() -> (w298:T9)
      n813 = Number To Decimal String(number=w282) -> (decimal integer string=w281:string)  [unwired: 1 in]
      n814 = Index Array(array=w298) -> (element=w297:T25)  [unwired: 1 in]
      n815 = Unbundle(w297) -> ("Position"=w280:cluster{"X":sgl, "Y":sgl}, "Radius"=w296:dbl)  [unwired: 1 out]
      n816 = Unbundle(w280) -> ("X"=w284:sgl, "Y"=w283:sgl)
      n817 = Subtract(x=w284, y=w296) -> (x-y=→"toplx":dbl)
      n818 = Add(x=w284, y=w296) -> (x+y=→"bottomrx":dbl)
      n819 = Add(x=w283, y=w296) -> (x+y=→"bottomry":dbl)
      n820 = Subtract(x=w283, y=w296) -> (x-y=→"toply":dbl)
      n821 = local read "bottomry"() -> (w288:dbl)
      n822 = local read "bottomrx"() -> (w289:dbl)
      n823 = local read "toply"() -> (w290:dbl)
      n824 = local read "toplx"() -> (w291:dbl)
      n825 = Build Array(w291, w290, w289, w288) -> (w285:dbl[])
      n826 = Array To Cluster(array=w285) -> (cluster=w287:T26)
      n827 = call "IMAQ Overlay Oval"("Bounding Rectangle"=w287, "Image"=w286) -> ("Image Out"=w279:T8)  [unwired: 8 in, 1 out]
      n828 = call "IMAQ Overlay Text"("String"=w281, "Origin"=w280, "Image"=w279) -> ("Image Out"=→"Camera 2":T8)  [unwired: 7 in, 1 out]
    }
    n829 = case shown="True" "Lock Current Spot" {
      frame False {
      }
      frame True {
        n830 = global read "red_tweezers_globals.vi" "Spots"() -> (w602:T1[])
        n831 = local read "Current Spot #"() -> (w603:dbl)
        "Locked Current Spot" <- w603
        n832 = Index Array(array=w602, index=w603) -> (element=w604:T1)
        n833 = local write "LCS"(0) -> ()
        n834 = Unbundle By Name(w604) -> ("Position.x"=w600:dbl, "Position.y"=w599:dbl)
        n835 = local write "Original Y"(w599) -> ()
        n836 = local write "Original X"(w600) -> ()
      }
    }
    n837 = call-poly "IMAQ Detect Shapes"("Image"=w41) -> ("Number of Matches Returned"=→"Number of Matches Returned":i32, "Circles"=→"Circles":T9)  [unwired: 8 in, 1 out]
    n838 = mathscript code="title('Bubble Tracker');\nxlim([0 1920]);\nylim([0 1080]);\nx1=Bubble1(:,1);\ny1= (1080-Bubble1(:,2));\n%x2=Bubble2(:,1);\n%y2= (1080-Bubble2(:,2));\n%x3=Bead(:,1);\n%y3= (1080-Bead(:,2));\nplot(x1, y1, 'go');\n%plot(x1, y1, 'go', x2, y2, 'ro',  x3, y3, 'bd');\n%plot(BeadL(:,1), (1080-BeadL(:,2)), 'go');"("Bubble1"=w39) -> ()  [unwired: 1 in, 1 out]
    n839 = case shown="True" "Mark Original Position" {
      frame False {
      }
      frame True {
        w605 = TRUE
        n840 = local read "1 for original positon"() -> (w607:dbl)
        n841 = local write "Mark Original Position"(FALSE) -> ()
        n842 = Add(x=w607, y=1) -> (x+y=w606:dbl)
        n843 = local write "1 for original positon"(w606) -> ()
        n844 = local read "New X"() -> (→"Original X":dbl)
        n845 = local read "New Y"() -> (→"Original Y":dbl)
        "MOP pressed After" <- w605
        "MOP pressed" <- w605
      }
    }
    n846 = case shown="True" "Rates" {
      frame False {
      }
      frame True {
        n847 = stacked-sequence {
          frame #0 {
            n848 = local read "Tab Control"() -> (w494:enum32{"Line", "Arc"})
            n849 = case shown="\"Line\"" w494 {
              tunnel: "Number of Planned Sequence Frames" -> [w495 w513]
              frame "Arc" {
                n850 = stacked-sequence {
                  tunnel: w495 -> [_ w508 _]
                  frame #0 {
                    n851 = expression code="(x/180.0)*pi" "degrees to radians"("Theta") -> (→"Radians":dbl)
                    n852 = local read "Radians"() -> (w507:dbl)
                    n853 = local read "Original Y"() -> (w501:dbl)
                    n854 = local read "Original X"() -> (w499:dbl)
                    n855 = Cosine(x=w507) -> (cos(x)=w496:dbl)
                    n856 = Sine(x=w507) -> (sin(x)=w498:dbl)
                    n857 = Multiply(x=w496, y="Radius X") -> (x*y=w500:dbl)
                    n858 = Multiply(x="Radius X", y=w498) -> (x*y=w502:dbl)
                    n859 = Subtract(x=w499, y=w500) -> (x-y=→"Center X":dbl)
                    n860 = Subtract(x=w501, y=w502) -> (x-y=→"Center Y":dbl)
                  }
                  frame #1 {
                    n861 = local read "Radians"() -> (w512:dbl)
                    n862 = Subtract(x=w508, y=1) -> (x-y=w510:dbl)
                    n863 = Divide(x=w512, y=w510) -> (x/y=→"Degree Rate":dbl)
                  }
                  frame #2 {
                  }
                }
              }
              frame "Line" {
                n864 = local read "Original X"() -> (w523:dbl)
                n865 = local read "Original Y"() -> (w521:dbl)
                n866 = Subtract(x=w513, y=1) -> (x-y=w515:dbl)
                n867 = local read "New Y"() -> (w520:dbl)
                n868 = local read "New X"() -> (w522:dbl)
                n869 = Subtract(x=w521, y=w520) -> (x-y=w518:dbl)
                n870 = Subtract(x=w523, y=w522) -> (x-y=w519:dbl)
                n871 = Divide(x=w518, y=w515) -> (x/y=→"Y Rate":dbl)
                n872 = Divide(x=w519, y=w515) -> (x/y=→"X Rate":dbl)
              }
            }
          }
          frame #1 {
            n873 = local write "Rates"(0) -> ()
          }
        }
      }
    }
    n874 = case shown="True" "Send Data" {
      frame False {
      }
      frame True {
        # "Pass data from Image Assistant to \nRed Tweezer New X & Y position"
        n875 = local read "Bubble y"() -> (w299:dbl)
        n876 = local read "Bubble x"() -> (w300:dbl)
        n877 = local write "New Y"(w299) -> ()
        n878 = local write "New X"(w300) -> ()
      }
    }
    n879 = local read "Sequence Instances"() -> (w103:dbl)
    n880 = case shown="True" w122 {
      tunnel: w128 -> [_ w673]
      frame False {
      }
      frame True {
        n881 = global write "red_tweezers_globals_INTERNAL.vi" "Image Overlay (extras from control loop)"(w673) -> ()
      }
    }
    n882 = local read "Counter"() -> (w102:dbl)
    n883 = call "red_tweezers_UNDO.vi"("Force Save"=w124, "This change is inconsequential (don't save it)"=w125, "Selection/Group"=w126, "Spots"=w127) -> ()  [unwired: 6 in, 2 out]
    n884 = call "sync_with_globals.vi"("Selection/Group"=w126, "Spots"=w127) -> ("Selection/Group 2"=w138:T7[], "Spots 2"=w89:T1[])  [unwired: 4 in]
    n885 = local read "Sequence Storer"() -> (w98:T1[][])
    n886 = local read "Sequence On?"() -> (w101:bool)
    n887 = local read "Sequence On?"() -> (w116:bool)
    n888 = call "SequenceControl.vi"("Sequence On? 2"=w101, "Counter 2"=w102, "Sequence Instances 2"=w103, "Sequence Storer"=w98) -> ("Time per Frame (ms) 2"=w96:dbl, "Sequence Order 2"=w99:dbl, "Reset 2"=w100:bool, "Sequence Storer 2"=w111:T1[][], "Clearance Button 2"=w110:bool, "Manual Edit 2"=w109:bool, "Save State 2"=w108:bool, "Play Sequence 2"=w105:bool, "Bubble ID to Empty 2"=w104:dbl, "Manual Sequence 2"=w106:bool, "Edit Sequence Mode 2"=w107:bool)  [unwired: 1 in]
    n889 = local write "Play Sequence"(w105) -> ()
    n890 = local write "Bubble ID to Empty"(w104) -> ()
    n891 = local write "Manual Sequence"(w106) -> ()
    n892 = local write "Reset"(w100) -> ()
    n893 = local write "Edit Sequence Mode"(w107) -> ()
    n894 = local write "Clearance Button"(w110) -> ()
    n895 = local write "Sequence Storer"(w111) -> ()
    n896 = local write "Save State"(w108) -> ()
    n897 = local write "Manual Edit"(w109) -> ()
    n898 = Or(x=w116, y="Manual Sequence") -> (x .or. y?=w115:bool)
    n899 = local write "Time per Frame (ms)"(w96) -> ()
    n900 = case shown="False" w115 {
      tunnel: [w643 w648] -> w119
      tunnel: w89 -> [w642 _]
      frame False {
        n901 = Or(x="Manual Edit", y="Edit Sequence Mode") -> (x .or. y?=w641:bool)
        n902 = case shown="False" w641 {
          tunnel: w642 -> [w644 _]
          tunnel: [w644 w645] -> w643
          frame False {
          }
          frame True {
            n903 = local read "Sequence Order"() -> (w646:dbl)
            n904 = local read "Sequence Storer"() -> (w647:T1[][])
            n905 = Index Array(array=w647, index (row)=w646) -> (element=w645:T1[])  [unwired: 1 in]
          }
        }
      }
      frame True {
        n906 = stacked-sequence {
          tunnel: [w650 _] -> w648
          frame #0 {
            n907 = local read "Counter"() -> (w651:dbl)
            n908 = local read "Sequence Storer"() -> (w652:T1[][])
            n909 = Index Array(array=w652, index (row)=w651) -> (element=w650:T1[])  [unwired: 1 in]
            n910 = Wait (ms)(milliseconds to wait="Time per Frame (ms)") -> ()  [unwired: 1 out]
          }
          frame #1 {
            n911 = local read "Sequence Instances"() -> (w654:dbl)
            n912 = local read "Counter"() -> (w657:dbl)
            n913 = Subtract(x=w654, y=1) -> (x-y=w655:dbl)
            n914 = Equal?(x=w657, y=w655) -> (x = y?=w656:bool)
            n915 = case shown="True" w656 {
              frame False {
                n916 = local read "Counter"() -> (w660:dbl)
                n917 = Add(x=w660, y=1) -> (x+y=→"Counter":dbl)
              }
              frame True {
                w661 = FALSE
                n918 = local write "Counter"(0) -> ()
                n919 = local write "Play Sequence"(w661) -> ()
                n920 = local write "Sequence On?"(w661) -> ()
              }
            }
          }
        }
      }
    }
    n921 = case shown="True" "Save State" {
      tunnel: w89 -> [_ w664]
      frame False {
      }
      frame True {
        n922 = local write "Save State"(FALSE) -> ()
        n923 = stacked-sequence {
          tunnel: w664 -> [w665 _]
          frame #0 {
            "Spot Storage" <- w665
          }
          frame #1 {
            n924 = local read "Spot Storage"() -> (w671:T1[])
            n925 = Replace Array Subset(array="Sequence Storer", new element=w671, index (row)="Sequence Order") -> (w669:T1[][])  [unwired: 1 in]
            n926 = Array Size(array=w669) -> (size(s)=w668:i32[])
            n927 = local write "Sequence Storer"(w669) -> ()
            n928 = Index Array(array=w668, index=0) -> (element=→"Sequence Instances":i32)
          }
        }
      }
    }
    n929 = feedback #10() -> (w143:T27)  [unwired: 1 out]
    n930 = call "Smoothed Frame Rate.vi"("Feedback In"=w143) -> ("Feedback Out"=w142:T27, "Frame Rate"=→"Interface Frame Rate":dbl)  [unwired: 1 in, 4 out]
    n931 = feedback-in #10(w142) -> ()
    n932 = local write "Sequence Order"(w99) -> ()
    n933 = case shown="True" "Clearance Button" {
      frame False {
      }
      frame True {
        # "This is the Bubble ID to Empty tool- this \"deletes\" the bubble in a sequence."
        n934 = local read "Sequence Order"() -> (w634:dbl)
        n935 = local read "Sequence Storer"() -> (w635:T1[][])
        n936 = Replace Array Subset(array=w635, new element=T12 {"Position"={"x"=nan, "y"=nan, "z"=nan}, "Intensity"=1.0, "Vortex Charge"=1, "Phase"=1.0, "NA Position"={"x"=0.0, "y"=0.0, "r"=1.0}, "Line Trapping"={"Vector"={"x"=0.0, "y"=0.0, "z"=0.0}, "Phase Gradient"=0.0}, "Amplitude Correction"=0.0} ("Cluster"), index (row)=w634, index (col)="Bubble ID to Empty") -> (w631:T1[][])
        n937 = local write "Sequence Storer"(w631) -> ()
      }
    }
    n938 = Not(x=w92) -> (.not. x?=w93:bool)
    n939 = Not(x="Output to SLM") -> (.not. x?=w94:bool)
    n940 = case shown="True" "Save" {
      frame False {
      }
      frame True {
        n941 = local read "Sequence Storer"() -> (w598:T1[][])
        n942 = call "SequenceSaver.vi"("Sequence Storer"=w598) -> ()  [unwired: 10 in, 1 out]
      }
    }
    n943 = And(x=w94, y=w93) -> (x .and. y?=w97:bool)
    n944 = case shown="True" "Load" {
      frame False {
      }
      frame True {
        n945 = call "SequenceSaver.vi"() -> ("Sequence Storer 2"=w597:T1[][])  [unwired: 11 in]
        n946 = local write "Sequence Storer"(w597) -> ()
      }
    }
    n947 = case shown="True" w97 {
      tunnel: w89 -> [w2063 _]
      frame False {
        n948 = call "UDP Sender generic_2.vi"("Spots"=w2063) -> ()  [unwired: 2 in, 1 out]
      }
      frame True {
      }
    }
    n949 = case shown="True" "Reset" {
      frame False {
      }
      frame True {
        n950 = local write "Counter"(0) -> ()
      }
    }
    n951 = case shown="True" "Add Additional Frames" {
      frame False {
      }
      frame True {
        # "This adds additional frames to the sequence."
        n952 = for {
          N: "Additional Frames Wanted" -> [_]
          i -> [w614]
          n953 = local read "Max Number of Bubbles"() -> (w618:dbl)
          n954 = Add(x=1, y=w614) -> (x+y=w615:i32)
          n955 = Add(x="Frame Location", y=w615) -> (x+y=w616:dbl)
          n956 = Initialize Array(T12 {"Position"={"x"=nan, "y"=nan, "z"=nan}, "Intensity"=1.0, "Vortex Charge"=1, "Phase"=1.0, "NA Position"={"x"=0.0, "y"=0.0, "r"=1.0}, "Line Trapping"={"Vector"={"x"=0.0, "y"=0.0, "z"=0.0}, "Phase Gradient"=0.0}, "Amplitude Correction"=0.0} ("Cluster"), w618) -> (w619:T28)
          n957 = local read "Sequence Storer"() -> (w620:T1[][])
          n958 = Insert Into Array(array=w620, index (row)=w616, new element=w619) -> (w621:T1[][])  [unwired: 1 in]
          n959 = local write "Sequence Storer"(w621) -> ()
        }
      }
    }
    n960 = case shown="True" "Initiate Creation" {
      frame False {
      }
      frame True {
        # "This create the array needed for a sequential\narray."
        n961 = local read "Number of Planned Sequence Frames"() -> (w624:dbl)
        n962 = for {
          N: w624 -> [_]
          tunnel: "Max Number of Bubbles" -> [w625]
          i -> [w628]
          n963 = Initialize Array(T12 {"Position"={"x"=nan, "y"=nan, "z"=nan}, "Intensity"=1.0, "Vortex Charge"=1, "Phase"=1.0, "NA Position"={"x"=0.0, "y"=0.0, "r"=1.0}, "Line Trapping"={"Vector"={"x"=0.0, "y"=0.0, "z"=0.0}, "Phase Gradient"=0.0}, "Amplitude Correction"=0.0} ("Cluster"), w625) -> (w626:T28)
          n964 = local read "Sequence Storer"() -> (w629:T1[][])
          n965 = Insert Into Array(array=w629, index (row)=w628, new element=w626) -> (w630:T1[][])  [unwired: 1 in]
          n966 = local write "Sequence Storer"(w630) -> ()
        }
      }
    }
    n967 = case shown="False" "Play Sequence" {
      frame False {
        n968 = local write "Sequence On?"(FALSE) -> ()
      }
      frame True {
        "Sequence On?" <- TRUE
      }
    }
    n969 = local read "Current Spot #"() -> (w72:dbl)
    n970 = local read "Selection/Group"() -> (w73:T7[])
    n971 = local read "# of Spots"() -> (w88:dbl)
    n972 = Not Equal?(x=w72, y=-1) -> (x != y?=w74:bool)
    n973 = local read "spots selected 2"() -> (w62:i32)
    n974 = Index Array(array=w73, index=w72) -> (element=w71:T7)
    n975 = Unbundle By Name(w71) -> ("Selected"=w70:bool)
    n976 = local read "spots selected"() -> (w63:i32)
    n977 = Not(x=w70) -> (.not. x?=w69:bool)
    n978 = And(x=w69, y=w74) -> (x .and. y?=w64:bool)
    n979 = Less?(x=w63, y=w62) -> (x < y?=w60:bool)
    n980 = case shown="True" "Insert" {
      tunnel: w89 -> [_ w302]
      tunnel: w88 -> [_ w301]
      frame False {
      }
      frame True {
        n981 = for {
          N: w301 -> [_]
          tunnel: w302 -> [w304]
          i -> [w303]
          n982 = stacked-sequence {
            tunnel: w304 -> [w306 w311 _]
            tunnel: w303 -> [_ w307 _]
            frame #0 {
              n983 = local read "Start at Which Frame?"() -> (→"Num":dbl)
              "Spot Storage 2" <- w306
            }
            frame #1 {
              n984 = local read "Selection/Group"() -> (w310:T7[])
              n985 = Index Array(array=w310, index=w307) -> (element=w309:T7)
              n986 = Unbundle By Name(w309) -> ("Selected"=w308:bool)
              n987 = case shown="True" w308 {
                tunnel: w311 -> [_ _]
                frame False {
                }
                frame True {
                  n988 = stacked-sequence {
                    frame #0 {
                      n989 = case shown="\"Line\"" "Tab Control" {
                        frame "Arc" {
                          n990 = local read "How Many Frames?"() -> (w315:dbl)
                          n991 = Subtract(x=w315, y=1) -> (x-y=w313:dbl)
                          n992 = for {
                            N: w315 -> [_]
                            tunnel: w313 -> [w316]
                            i -> [w318]
                            # "What is this ^\n\nFor # of sequence\nframes, don't worry\nabout it"
                            # "How to make position x and y?\nIt's called a cluster, inser the new position to Position.x and Position.y"
                            n993 = Equal?(x=w316, y=w318) -> (x = y?=w317:bool)
                            n994 = case shown="False" w317 {
                              tunnel: [w341 w350] -> w320
                              tunnel: [w340 w349] -> w319
                              tunnel: w318 -> [w337 _]
                              frame False {
                                # "calculating new position"
                                n995 = local read "Degree Rate"() -> (w339:dbl)
                                n996 = Multiply(x=w339, y=w337) -> (x*y=w338:dbl)
                                n997 = Cosine(x=w338) -> (cos(x)=w347:dbl)
                                n998 = Sine(x=w338) -> (sin(x)=w348:dbl)
                                n999 = local read "Radius X"() -> (w346:dbl)
                                n1000 = Multiply(x=w346, y=w348) -> (x*y=w345:dbl)
                                n1001 = Multiply(x=w347, y=w346) -> (x*y=w344:dbl)
                                n1002 = local read "Center X"() -> (w343:dbl)
                                n1003 = local read "Center Y"() -> (w342:dbl)
                                n1004 = Add(x=w343, y=w344) -> (x+y=w341:dbl)
                                n1005 = Add(x=w342, y=w345) -> (x+y=w340:dbl)
                              }
                              frame True {
                                n1006 = global read "red_tweezers_globals.vi" "Spots"() -> (w353:T1[])
                                n1007 = local read "Numeric"() -> (w352:dbl)
                                n1008 = Index Array(array=w353, index=w352) -> (element=w351:T1)
                                n1009 = Unbundle By Name(w351) -> ("Position.x"=w350:dbl, "Position.y"=w349:dbl)
                              }
                            }
                            n1010 = local read "Spot Storage 2"() -> (w336:T1[])
                            n1011 = local read "Numeric"() -> (w335:dbl)
                            n1012 = Index Array(array=w336, index=w335) -> (element=w322:T1)
                            n1013 = local read "Start at Which Frame?"() -> (w324:dbl)
                            n1014 = Bundle By Name(cluster=w322, "Position.x"=w320, "Position.y"=w319) -> (w321:T1)
                            n1015 = local read "How Many Frames?"() -> (w323:dbl)
                            n1016 = Subtract(x=w324, y=w318) -> (x-y=w333:dbl)
                            n1017 = local read "Sequence Storer"() -> (w334:T1[][])
                            n1018 = local read "Numeric"() -> (w329:dbl)
                            n1019 = Add(x=w333, y=w323) -> (x+y=w332:dbl)
                            n1020 = Subtract(x=w332, y=1) -> (x-y=w330:dbl)
                            n1021 = Replace Array Subset(array=w334, new element=w321, index (row)=w330, index (col)=w329) -> (w328:T1[][])
                            n1022 = Array Size(array=w328) -> (size(s)=w327:i32[])
                            n1023 = local write "Sequence Storer"(w328) -> ()
                            n1024 = Index Array(array=w327, index=0) -> (element=w325:i32)
                            n1025 = local write "Sequence Instances"(w325) -> ()
                          }
                        }
                        frame "Line" {
                          n1026 = local read "Rates"() -> (w354:dbl)
                          n1027 = case shown="0" w354 {
                            frame 1, Default {
                              # "This is the automatic sequence generator which allows for the creation of the sequence. This calculates the LAST coordinates of each bubble first\nbefore going for the first few coordinates of the sequence."
                              n1028 = local read "How Many Frames?"() -> (w355:dbl)
                              n1029 = for {
                                N: w355 -> [_]
                                i -> [w367]
                                # "For why do we multiply?"
                                n1030 = local read "Spot Storage 2"() -> (w368:T1[])
                                n1031 = local read "Numeric"() -> (w358:dbl)
                                n1032 = local read "X Rate"() -> (w374:dbl)
                                n1033 = local read "Y Rate"() -> (w373:dbl)
                                n1034 = Index Array(array=w368, index=w358) -> (element=w365:T1)
                                n1035 = Unbundle By Name(w365) -> ("Position.x"=w375:dbl, "Position.y"=w371:dbl)
                                n1036 = Multiply(x=w374, y=w367) -> (x*y=w372:dbl)
                                n1037 = Multiply(x=w373, y=w367) -> (x*y=w366:dbl)
                                n1038 = local read "Start at Which Frame?"() -> (w357:dbl)
                                n1039 = Subtract(x=w375, y=w372) -> (x-y=w370:dbl)
                                n1040 = Subtract(x=w371, y=w366) -> (x-y=w369:dbl)
                                n1041 = Bundle By Name(cluster=w365, "Position.x"=w370, "Position.y"=w369) -> (w360:T1)
                                n1042 = Add(x=w357, y=w367) -> (x+y=w356:dbl)
                                n1043 = local read "Sequence Storer"() -> (w376:T1[][])
                                n1044 = local read "Numeric"() -> (w359:dbl)
                                n1045 = Replace Array Subset(array=w376, new element=w360, index (row)=w356, index (col)=w359) -> (w364:T1[][])
                                n1046 = Array Size(array=w364) -> (size(s)=w363:i32[])
                                n1047 = local write "Sequence Storer"(w364) -> ()
                                n1048 = Index Array(array=w363, index=0) -> (element=w361:i32)
                                n1049 = local write "Sequence Instances"(w361) -> ()
                              }
                            }
                            frame 0 {
                              # "This is the automatic sequence generator which allows for the creation of the sequence. This calculates the LAST coordinates of each bubble first\nbefore going for the first few coordinates of the sequence."
                              n1050 = local read "How Many Frames?"() -> (w377:dbl)
                              n1051 = for {
                                N: w377 -> [_]
                                i -> [w392]
                                # "For why do we multiply?"
                                n1052 = local read "Spot Storage 2"() -> (w394:T1[])
                                n1053 = local read "Numeric"() -> (w378:dbl)
                                n1054 = local read "X Rate"() -> (w400:dbl)
                                n1055 = local read "Y Rate"() -> (w399:dbl)
                                n1056 = Index Array(array=w394, index=w378) -> (element=w385:T1)
                                n1057 = Unbundle By Name(w385) -> ("Position.x"=w401:dbl, "Position.y"=w397:dbl)
                                n1058 = Multiply(x=w400, y=w392) -> (x*y=w398:dbl)
                                n1059 = Multiply(x=w399, y=w392) -> (x*y=w386:dbl)
                                "probe" <- w386
                                n1060 = Subtract(x=w401, y=w398) -> (x-y=w396:dbl)
                                n1061 = Subtract(x=w397, y=w386) -> (x-y=w395:dbl)
                                n1062 = Bundle By Name(cluster=w385, "Position.x"=w396, "Position.y"=w395) -> (w380:T1)
                                n1063 = Subtract(x="Start at Which Frame?", y=w392) -> (x-y=w391:dbl)
                                n1064 = local read "Sequence Storer"() -> (w402:T1[][])
                                n1065 = local read "Numeric"() -> (w379:dbl)
                                n1066 = local read "How Many Frames?"() -> (w390:dbl)
                                n1067 = Add(x=w391, y=w390) -> (x+y=w389:dbl)
                                n1068 = Subtract(x=w389, y=1) -> (x-y=w387:dbl)
                                n1069 = Replace Array Subset(array=w402, new element=w380, index (row)=w387, index (col)=w379) -> (w384:T1[][])
                                n1070 = Array Size(array=w384) -> (size(s)=w383:i32[])
                                n1071 = local write "Sequence Storer"(w384) -> ()
                                n1072 = Index Array(array=w383, index=0) -> (element=w381:i32)
                                n1073 = local write "Sequence Instances"(w381) -> ()
                              }
                            }
                          }
                        }
                      }
                    }
                    frame #1 {
                      n1074 = local read "How Many Frames?"() -> (w403:dbl)
                      n1075 = for {
                        N: w403 -> [_]
                        n1076 = stacked-sequence {
                          frame #0 {
                            n1077 = local read "Sequence Storer"() -> (w406:T1[][])
                            n1078 = local read "Num"() -> (w405:dbl)
                            n1079 = local read "# of Spots"() -> (w409:dbl)
                            n1080 = Index Array(array=w406, index (row)=w405) -> (element=w404:T1[])  [unwired: 1 in]
                            n1081 = Add(x=1, y=w405) -> (x+y=w407:dbl)
                            n1082 = for {
                              N: w409 -> [_]
                              tunnel: w409 -> [w413]
                              tunnel: w407 -> [w412]
                              tunnel: w404 -> [w411]
                              i -> [w410]
                              n1083 = stacked-sequence {
                                tunnel: w413 -> [w415 _]
                                tunnel: w412 -> [w419 _]
                                tunnel: w411 -> [w418 _]
                                tunnel: w410 -> [w417 _]
                                frame #0 {
                                n1084 = local read "LCounter"() -> (w414:dbl)
                                n1085 = Subtract(x=w415, y=w414) -> (x-y=w416:dbl)
                                n1086 = for {
                                N: w416 -> [_]
                                tunnel: w418 -> [w442]
                                tunnel: w417 -> [w423]
                                tunnel: w418 -> [w441]
                                tunnel: w419 -> [w428]
                                i -> [w422]
                                # "This checks whether a bubble intersects with another\nor not."
                                n1087 = local read "LCounter"() -> (w420:dbl)
                                n1088 = Add(x=w420, y=w422) -> (x+y=w421:dbl)
                                "Numeric 4" <- w421
                                n1089 = Index Array(array=w442, index=w421) -> (element=w443:T1)
                                n1090 = Index Array(array=w441, index=w423) -> (element=w444:T1)
                                n1091 = Unbundle By Name(w443) -> ("Position.x"=w439:dbl, "Position.y"=w437:dbl)
                                n1092 = Unbundle By Name(w444) -> ("Position.x"=w440:dbl, "Position.y"=w438:dbl)
                                n1093 = Subtract(x=w438, y=w437) -> (x-y=w435:dbl)
                                n1094 = Subtract(x=w440, y=w439) -> (x-y=w436:dbl)
                                n1095 = Square(x=w435) -> (x^2=w433:dbl)
                                n1096 = Square(x=w436) -> (x^2=w434:dbl)
                                n1097 = local write "Num"(w428) -> ()
                                n1098 = local read "Buffer Zone"() -> (w431:dbl)
                                n1099 = Add(x=w434, y=w433) -> (x+y=w432:dbl)
                                n1100 = Square Root(x=w432) -> (sqrt(x)=w425:dbl)
                                n1101 = Multiply(x=2, y=w431) -> (x*y=w429:dbl)
                                n1102 = Less Or Equal?(x=w425, y=w429) -> (x <= y?=w427:bool)
                                n1103 = Not Equal?(x=w423, y=w421) -> (x != y?=w424:bool)
                                n1104 = And(x=w424, y=w427) -> (x .and. y?=w426:bool)
                                n1105 = case shown="True" w426 {
                                tunnel: w428 -> [_ w445]
                                frame False {
                                }
                                frame True {
                                n1106 = stacked-sequence {
                                tunnel: w445 -> [w456 _]
                                frame #0 {
                                # "This prints the string which displays the information whether there are potential collisions\nor not."
                                n1107 = Subtract(x=w456, y=1) -> (x-y=w455:dbl)
                                n1108 = local read "Array"() -> (w453:dbl[])
                                n1109 = Insert Into Array(array=w453, index=0, new element=w455) -> (w446:dbl[])
                                "Array" <- w446
                                n1110 = Array Size(array=w446) -> (size(s)=w447:i32)
                                n1111 = Number To Decimal String(number=w447) -> (decimal integer string=w452:string)  [unwired: 1 in]
                                n1112 = Concatenate Strings("There are ", w452) -> (w450:string)
                                n1113 = Concatenate Strings(w450, " potential collisions in the sequence. Please examine the array to obtain the sequence numbers that need to be edited.") -> (→"Collision Detector":string)
                                }
                                frame #1 {
                                n1114 = stacked-sequence {
                                frame #0 {
                                n1115 = local read "Array"() -> (w459:dbl[])
                                n1116 = Array Size(array=w459) -> (size(s)=w458:i32)
                                n1117 = for {
                                N: w458 -> [_]
                                tunnel: w458 -> [w461]
                                tunnel: w458 -> [w460]
                                n1118 = stacked-sequence {
                                tunnel: [w479 _] -> _
                                tunnel: w461 -> [w474 _]
                                tunnel: w460 -> [_ _]
                                frame #0 {
                                n1119 = local read "Counter for String"() -> (w478:dbl)
                                n1120 = local read "Array"() -> (w479:dbl[])
                                n1121 = Multiply(x=w474, y=3) -> (x*y=w471:i32)
                                n1122 = Index Array(array=w479, index=w478) -> (element=w469:dbl)
                                n1123 = Subtract(x=w471, y=2) -> (x-y=w464:i32)
                                n1124 = Number To Decimal String(number=w469) -> (decimal integer string=w470:string)  [unwired: 1 in]
                                n1125 = local read "String counter"() -> (w462:dbl)
                                n1126 = local read "String 2"() -> (w476:string)
                                n1127 = Concatenate Strings(w470, ", ") -> (w477:string)
                                n1128 = Greater?(x=w469, y=9) -> (0:w466:bool)
                                n1129 = Add(x=w462, y=w464) -> (x+y=w465:dbl)
                                n1130 = Concatenate Strings(w477, w476) -> (w463:string)
                                "String 2" <- w463
                                n1131 = case shown="True" w466 {
                                frame False {
                                }
                                frame True {
                                n1132 = local read "String counter"() -> (w480:dbl)
                                n1133 = Add(x=w480, y=1) -> (x+y=→"String counter":dbl)
                                }
                                }
                                n1134 = Replace Substring(2:w465, 5:w463) -> (0:w468:string)  [unwired: 2 in, 1 out]
                                n1135 = local write "Sequence Frames To Check"(w468) -> ()
                                }
                                frame #1 {
                                n1136 = local read "Counter for String"() -> (w483:dbl)
                                n1137 = Add(x=w483, y=1) -> (x+y=w485:dbl)
                                n1138 = local write "Counter for String"(w485) -> ()
                                }
                                }
                                }
                                }
                                frame #1 {
                                w486 = 0
                                n1139 = local write "String counter"(w486) -> ()
                                "Counter for String" <- w486
                                }
                                }
                                }
                                }
                                }
                                }
                                "Numeric 3" <- w428
                                }
                                }
                                frame #1 {
                                n1140 = local read "LCounter"() -> (w487:dbl)
                                n1141 = Add(x=w487, y=1) -> (x+y=→"LCounter":dbl)
                                }
                              }
                            }
                          }
                          frame #1 {
                            n1142 = local write "LCounter"(0) -> ()
                          }
                        }
                      }
                    }
                    frame #2 {
                      n1143 = local write "LCounter"(0) -> ()
                    }
                  }
                }
              }
              "Numeric" <- w307
            }
            frame #2 {
              n1144 = local write "Insert"(FALSE) -> ()
            }
          }
        }
      }
    }
    n1145 = And(x=w60, y=w64) -> (x .and. y?=w65:bool)
    n1146 = case shown="True" w65 {
      frame False {
      }
      frame True {
        n1147 = local read "# of Spots"() -> (w532:dbl)
        n1148 = for {
          N: w532 -> [_]
          i -> [w534]
          stop <- w533 stop-if-true
          n1149 = local read "Selection/Group"() -> (w536:T7[])
          n1150 = Index Array(array=w536, index=w534) -> (element=w535:T7)
          n1151 = Unbundle By Name(w535) -> ("Selected"=w533:bool)
          n1152 = case shown="True" w533 {
            tunnel: w534 -> [_ w538]
            frame False {
            }
            frame True {
              n1153 = local write "Current Spot #"(w538) -> ()
              "Induce check" <- TRUE
            }
          }
        }
      }
    }
    n1154 = local read "spots selected"() -> (w75:i32)
    n1155 = local read "spots selected 2"() -> (w76:i32)
    n1156 = local read "Prev Current Spot"() -> (w84:dbl)
    n1157 = local read "Current Spot #"() -> (w85:dbl)
    n1158 = Not Equal?(x=w85, y=w84) -> (x != y?=w83:bool)
    n1159 = Greater?(x=w76, y=w75) -> (0:w77:bool)
    n1160 = local read "Induce check"() -> (w66:bool)
    n1161 = Or(x=w83, y=w77) -> (x .or. y?=w68:bool)
    n1162 = Or(x=w68, y=w66) -> (x .or. y?=w67:bool)
    n1163 = case shown="True" w67 {
      frame False {
      }
      frame True {
        n1164 = stacked-sequence {
          frame #0 {
            # "A small 100 ms delay is given to provide enough time for the data to be processed properly."
            n1165 = local read "Null array"() -> (w544:dbl[])
            n1166 = local write "What to Check"(w544) -> ()
            n1167 = local write "ID"(w544) -> ()
            n1168 = local read "Current Spot #"() -> (w546:dbl)
            n1169 = local write "Potential Collisions"(0) -> ()
            n1170 = local read "Spot Checker"() -> (w545:T1[])
            n1171 = Index Array(array=w545, index=w546) -> (element=w547:T1)
            n1172 = Wait (ms)(milliseconds to wait=10) -> ()  [unwired: 1 out]
            n1173 = Unbundle By Name(w547) -> ("Position.x"=w541:dbl, "Position.y"=w542:dbl)
            n1174 = local write "Orig Y SC"(w542) -> ()
            n1175 = local write "Orig X SC"(w541) -> ()
            n1176 = local write "Induce check"(FALSE) -> ()
          }
          frame #1 {
            n1177 = local read "# of Spots"() -> (w548:dbl)
            n1178 = for {
              N: w548 -> [_]
              tunnel: w548 -> [w553]
              i -> [w549]
              n1179 = local read "Selection/Group"() -> (w552:T7[])
              n1180 = Index Array(array=w552, index=w549) -> (element=w551:T7)
              n1181 = Unbundle By Name(w551) -> ("Selected"=w550:bool)
              n1182 = case shown="True" w550 {
                tunnel: w553 -> [_ w555]
                tunnel: w549 -> [_ w554]
                frame False {
                }
                frame True {
                  n1183 = for {
                    N: w555 -> [_]
                    tunnel: w554 -> [w556]
                    i -> [w557]
                    # "If the bubble is not selected, find difference of bubble to bubble\nbeing checked"
                    n1184 = local read "Selection/Group"() -> (w561:T7[])
                    n1185 = Index Array(array=w561, index=w557) -> (element=w560:T7)
                    n1186 = Unbundle By Name(w560) -> ("Selected"=w558:bool)
                    n1187 = Not(x=w558) -> (.not. x?=w559:bool)
                    n1188 = case shown="True" w559 {
                      tunnel: w557 -> [_ w565]
                      tunnel: w556 -> [_ w564]
                      tunnel: w556 -> [_ w563]
                      frame False {
                      }
                      frame True {
                        n1189 = local read "Spot Checker"() -> (w582:T1[])
                        n1190 = Index Array(array=w582, index=w565) -> (element=w583:T1)
                        n1191 = Index Array(array=w582, index=w564) -> (element=w581:T1)
                        n1192 = Unbundle By Name(w581) -> ("Position.x"=w578:dbl, "Position.y"=w574:dbl)
                        n1193 = Unbundle By Name(w583) -> ("Position.x"=w575:dbl, "Position.y"=w571:dbl)
                        n1194 = local read "Area+ Buffer"() -> (w562:dbl)
                        n1195 = Subtract(x=w578, y=w562) -> (x-y=w579:dbl)
                        n1196 = Greater Or Equal?(x=w575, y=w579) -> (x >= y?=w580:bool)
                        n1197 = Add(x=w574, y=w562) -> (x+y=w573:dbl)
                        n1198 = Subtract(x=w574, y=w562) -> (x-y=w572:dbl)
                        n1199 = Add(x=w578, y=w562) -> (x+y=w576:dbl)
                        n1200 = Less Or Equal?(x=w571, y=w573) -> (x <= y?=w570:bool)
                        n1201 = Greater Or Equal?(x=w571, y=w572) -> (x >= y?=w569:bool)
                        n1202 = Less Or Equal?(x=w575, y=w576) -> (x <= y?=w577:bool)
                        n1203 = And(x=w580, y=w577) -> (x .and. y?=w567:bool)
                        n1204 = And(x=w570, y=w569) -> (x .and. y?=w568:bool)
                        n1205 = And(x=w567, y=w568) -> (x .and. y?=w566:bool)
                        n1206 = case shown="True" w566 {
                          tunnel: w565 -> [_ _]
                          tunnel: w565 -> [_ w585]
                          tunnel: w563 -> [_ w584]
                          frame False {
                          }
                          frame True {
                            n1207 = stacked-sequence {
                              tunnel: w585 -> [w586 _]
                              tunnel: w584 -> [w587 _]
                              frame #0 {
                                n1208 = local read "Potential Collisions"() -> (w590:dbl)
                                n1209 = local read "What to Check"() -> (w591:dbl[])
                                n1210 = Insert Into Array(array=w591, index=w590, new element=w586) -> (w592:dbl[])
                                n1211 = local read "ID"() -> (w589:dbl[])
                                n1212 = local write "What to Check"(w592) -> ()
                                n1213 = Insert Into Array(array=w589, index=w590, new element=w587) -> (w588:dbl[])
                                n1214 = local write "ID"(w588) -> ()
                              }
                              frame #1 {
                                n1215 = local read "Potential Collisions"() -> (w595:dbl)
                                n1216 = Add(x=w595, y=1) -> (x+y=w593:dbl)
                                n1217 = local write "Potential Collisions"(w593) -> ()
                              }
                            }
                          }
                        }
                      }
                    }
                  }
                }
              }
            }
          }
          frame #2 {
            n1218 = local read "Current Spot #"() -> (w596:dbl)
            n1219 = local write "Prev Current Spot"(w596) -> ()
          }
        }
      }
    }
    n1220 = local read "Buffer Zone"() -> (w81:dbl)
    n1221 = Multiply(x=w81, y=2) -> (x*y=w82:dbl)
    n1222 = Add(x="Area to check", y=w82) -> (x+y=→"Area+ Buffer":dbl)
    n1223 = feedback #11() -> (w54:dbl)  [unwired: 1 in]
    n1224 = Equal?(x=w54, y=10000) -> (x = y?=w55:bool)
    n1225 = call "Elapsed Time"("Reset"=w55) -> ("Elapsed Time (s)"=w53:dbl, "Time has Elapsed"=w58:bool)  [unwired: 11 in, 6 out]
    "Elapsed Time" <- w53
    n1226 = feedback-in #11(w53) -> ()
    n1227 = And(x="On", y=w58) -> (x .and. y?=w59:bool)
    n1228 = case shown="True" w59 {
      frame False {
      }
      frame True {
        n1229 = local read "Position"() -> (w531:cluster{"x":dbl, "y":dbl, "z":dbl})
        n1230 = Unbundle By Name(w531) -> ("x"=→"X Pos every 10 sec":dbl)
      }
    }
    n1231 = case shown="True" "OK Button" {
      frame False {
      }
      frame True {
        n1232 = script code="clear all;\nclc;\n\ng = gigecam('169.254.154.83');\n\ng.PixelFormat= 'BayerGR8'\n\nimg = snapshot(g);\n\nimshow(img);"() -> ()  [unwired: 1 in, 1 out]
      }
    }
    n1233 = case shown="True" "O Button" {
      frame False {
      }
      frame True {
        n1234 = script code="%\n    rslt = Hough1_data(img);\n\n    % Frame translation\n    %- omit this as of now \n    \n    % Control method\n    increment = 10; %assuming the diamiter of the agent around 20 pic \n    \n    %- NewLoc = [x,y] whose unit is px\n    %- update new location based on current location obtained by the camera\n    NewLoc(1)= rslt(1);\n    NewLoc(2)= rslt(2);\n    \n    \n    % Update microrobot location with NewLoc\n    % the single robot would move to oblique downword\n    \n    % wait seconds"() -> ("NewLoc"=w527:dbl[])  [unwired: 1 in, 1 out]
        n1235 = Index Array(array=w527, index=1) -> (element=→"Y":dbl)
        n1236 = Index Array(array=w527, index=0) -> (element=→"X":dbl)
      }
    }
    "Rates" <- w34
    "LCS" <- w34
  }
  n1237 = flat-sequence {
    tunnel: w6 -> [w2066]
    tunnel: w5 -> [w2065]
    tunnel: [w2064] -> w3
    frame #0 {
      n1238 = disable-structure shown="\"IMAQdx with ROI tool buttons (default)\"" {
        disable-tunnel: w2066 -> [_ _ _ _ _ _]
        disable-tunnel: w2065 -> [_ _ w2124 _ _ _]
        disable-tunnel: [_ _ w2123 _ _ _] -> w2064
        frame condition #0 {
          w2068 = u32 10 ("Number of buffers")
          (unwired) FALSE ("background subtraction")
          # "This subdiagram uses the IMAQ drivers, with a pre-allocated ringbuffer for images.  This is the code I use with my Mikrotron MC1362-CL"
          n1239 = call <vilib>:"IMAQ Init.vi"("Interface Name"="img0") -> ("IMAQ Session Out"=w2075:refnum<k11>)  [unwired: 9 in, 1 out]
          n1240 = call <vilib>:"IMAQ Configure List.vi"("Region of interest"="Global ROI (requires restart)", "Number of buffers"=w2068, "Continuous?"=enum16{"One-Shot", "Continuous"}."Continuous", "IMAQ Session In"=w2075) -> ("error out"=w2069:errorcluster, "IMAQ Session Out"=w2071:refnum<k11>)  [unwired: 6 in]
          n1241 = for {
            N: w2068 -> [_]
            tunnel: 0 ("Channel") -> [w2088]
            shift-right: [w2091] -> w2073
            shift-left: w2069 -> [w2087]
            shift-right: [w2090] -> w2072
            shift-left: w2071 -> [w2089]
            i -> [w2086]
            n1242 = Format Into String(format string="mikrotronbuffer%04d", w2086) -> (resulting string=w2084:string)  [unwired: 2 in, 1 out]
            n1243 = call "IMAQ Create"("Image Name"=w2084) -> ("New Image"=w2083:T8)  [unwired: 4 in, 1 out]
            n1244 = call <vilib>:"IMAQ Configure Buffer.vi"("Channel"=w2088, "error in (no error)"=w2087, "Buffer Number"=w2086, "Image In"=w2083, "IMAQ Session In"=w2089) -> ("error out"=w2091:errorcluster, "IMAQ Session Out"=w2090:refnum<k11>)  [unwired: 5 in]
          }
          n1245 = call <vilib>:"IMAQ Start.vi"("error in (no error)"=w2073, "IMAQ Session In"=w2072) -> ("error out"=w2079:errorcluster, "IMAQ Session Out"=w2080:refnum<k11>)  [unwired: 8 in]
          n1246 = call "IMAQ Create"("Image Name"="Red Tweezers live image") -> ("New Image"=w2081:T8)  [unwired: 3 in, 2 out]
          n1247 = while {
            tunnel: w2080 -> [w2099]
            tunnel: w2079 -> [w2098]
            tunnel: w2081 -> [_]
            tunnel: [w2100] -> w2077
            tunnel: [w2093] -> w2078
            i -> [w2095]
            stop <- w2101 stop-if-true
            n1248 = local read "stop"() -> (w2101:bool)
            n1249 = call <vilib>:"IMAQ Extract Buffer.vi"("error in (no error)"=w2098, "Buffer to extract"=w2095, "IMAQ Session In"=w2099) -> ("error out"=w2093:errorcluster, "Image Out"=w2092:T8, "IMAQ Session Out"=w2100:refnum<k11>)  [unwired: 3 in, 3 out]
            n1250 = call "imageQ_camera_hook.vi"("Image"=w2092) -> ()  [unwired: 11 in]
            n1251 = feedback #12() -> (w2096:T27)  [unwired: 1 in]
            n1252 = call "Smoothed Frame Rate.vi"("Feedback In"=w2096) -> ("Feedback Out"=w2097:T27, "Frame Rate"=w2094:dbl)  [unwired: 1 in, 4 out]
            n1253 = feedback-in #12(w2097) -> ()
            n1254 = global write "red_tweezers_globals_INTERNAL_VOLATILE.vi" "Video Frame Rate"(w2094) -> ()
          }
          n1255 = call <vilib>:"IMAQ Close.vi"("error in (no error)"=w2078, "IMAQ Session In"=w2077) -> ()  [unwired: 9 in, 1 out]
        }
        frame condition #1 {
          (unwired) FALSE ("background subtraction")
          # "This subdiagram acquires using the IMAQdx drivers.  This covers most FireWire and GigE cameras (at least the ones supporting the IIDC or GenICam standards)."
          n1256 = call <vilib>:"IMAQdx Open Camera.vi"("Session In"=T6 "dalsaGenie") -> ("error out"=w2104:errorcluster, "Session Out"=w2103:T6)  [unwired: 9 in]
          n1257 = call <vilib>:"IMAQdx Configure Grab.vi"("error in"=w2104, "Session In"=w2103) -> ("error out"=w2105:errorcluster, "Session Out"=w2106:T6)  [unwired: 8 in]
          n1258 = call "IMAQ Create"("Image Name"="Red Tweezers live image") -> ("New Image"=w2109:T8)  [unwired: 3 in, 2 out]
          n1259 = while {
            tunnel: w2106 -> [w2118]
            tunnel: w2105 -> [w2117]
            tunnel: w2109 -> [w2111]
            tunnel: [w2119] -> w2107
            tunnel: [w2113] -> w2108
            stop <- w2120 stop-if-true
            n1260 = local read "stop"() -> (w2120:bool)
            n1261 = call <vilib>:"IMAQdx Grab.vi"("error in"=w2117, "Image In"=w2111, "Session In"=w2118) -> ("error out"=w2113:errorcluster, "Image Out"=w2112:T8, "Session Out"=w2119:T6)  [unwired: 5 in, 1 out]
            n1262 = call "imageQ_camera_hook.vi"("Image"=w2112) -> ()  [unwired: 11 in]
            n1263 = feedback #13() -> (w2115:T27)  [unwired: 1 in]
            n1264 = call "Smoothed Frame Rate.vi"("Feedback In"=w2115) -> ("Feedback Out"=w2116:T27, "Frame Rate"=w2114:dbl)  [unwired: 1 in, 4 out]
            n1265 = feedback-in #13(w2116) -> ()
            n1266 = global write "red_tweezers_globals_INTERNAL_VOLATILE.vi" "Video Frame Rate"(w2114) -> ()
          }
          n1267 = call <vilib>:"IMAQdx Close Camera.vi"("error in"=w2108, "Session In"=w2107) -> ()  [unwired: 9 in, 1 out]
        }
        frame condition #2 {
          # "This subdiagram acquires using the IMAQdx drivers.  This covers most FireWire and GigE cameras (at least the ones supporting the IIDC or GenICam standards)."
          n1268 = call <vilib>:"IMAQdx Open Camera.vi"("Session In"="Camera") -> ("error out"=w2132:errorcluster, "Session Out"=w2131:T6)  [unwired: 9 in]
          n1269 = call <vilib>:"IMAQdx Configure Grab.vi"("error in"=w2132, "Session In"=w2131) -> ("error out"=w2128:errorcluster, "Session Out"=w2129:T6)  [unwired: 8 in]
          n1270 = call "IMAQ Create"("Image Name"="Red Tweezers live image") -> ("New Image"=w2126:T8)  [unwired: 3 in, 2 out]
          n1271 = call "IMAQdx_get_ROI.vi"("Session In"=w2129) -> ("ROI"=w2125:u32[], "Session Out"=w2127:T6)  [unwired: 8 in]
          n1272 = while {
            shift-right: [w2141] -> w2121
            shift-left: w2128 -> [w2142]
            shift-right: [w2138] -> w2122
            shift-left: w2127 -> [w2139]
            tunnel: w2126 -> [w2137]
            tunnel: w2125 -> [w2136]
            tunnel: w2124 -> [w2135]
            tunnel: [w2134] -> w2123
            stop <- w2148 stop-if-true
            n1273 = event shown="[0] Timeout" {
              selector: _ -> [_ _ _]
              dyn-events: _ -> [_ _ _]
              timeout: 0 -> [_ _ _]
              tunnel: w2142 -> [w2155 w2162 w2177]
              tunnel: [w2154 w2162 w2177] -> w2141
              tunnel: w2139 -> [w2153 w2163 w2178]
              tunnel: [w2152 w2163 w2178] -> w2138
              tunnel: w2137 -> [w2151 _ _]
              tunnel: w2136 -> [w2150 _ _]
              tunnel: w2135 -> [_ w2161 w2176]
              event Timeout {
                w2149 = 0  # timeout in ms
                # "Use a timeout of a few hundred ms if you want to acquire just fast enough to update the image- or a timeout of zero to run the camera at full speed."
                # "This VI sends the image to the loop above for display.\nIt's better to do this than to display here, because it separates the camera loop from the front panel a bit, and increases speed without sacrificing responsiveness of the UI.  Of course, using the event structure removes some of those benefits- but it is possible to write a high-performance camera loop with fast particle tracking, and still use this mechanism to display images without slowing down acquisition."
                # "If we're not dealing with other events, acquire from the camera."
                n1274 = event-data() -> ("Time"=w2160:u32)  [unwired: 1 in]
                n1275 = call <vilib>:"IMAQdx Grab.vi"("error in"=w2155, "Image In"=w2151, "Session In"=w2153) -> ("error out"=w2154:errorcluster, "Image Out"=w2157:T8, "Session Out"=w2152:T6)  [unwired: 5 in, 1 out]
                n1276 = call "IMAQ Clear Overlay"("Image"=w2157) -> ("Image Out"=w2156:T8)  [unwired: 9 in, 1 out]
                n1277 = Multiply(x=w2160, y=u32 1000) -> (x*y=w2158:u32)
                n1278 = call "imageQ_camera_hook.vi"("timeout in ms (0=don't wait if there are no requests)"=w2149, "Timestamp/us"=w2158, "ROI"=w2150, "Image"=w2156) -> ()  [unwired: 8 in]
              }
              event "Draw ROI", "Zoom": Value Change {
                # "This changes the current mouse mode on the image, allowing zooming/drawing of ROI (which can be useful if you want to window down a camera for particle tracking)."
                n1279 = event-data() -> ("CtlRef"=w2168:refnum<vi>)  [unwired: 1 in]
                n1280 = control-ref of="Draw ROI"() -> (w2169:refnum<vi>)
                n1281 = Equal?(x=w2169, y=w2168) -> (x = y?=w2167:bool)
                n1282 = case shown="True" w2167 {
                  tunnel: [w2172 w2175] -> w2166
                  tunnel: [TRUE ("stop") FALSE ("stop")] -> w2164
                  tunnel: [FALSE ("Update Indicators?") TRUE ("Update Indicators?")] -> w2165
                  frame False {
                    w2172 = u32 8 items=["Zoom Tool"=8, "Selection Tool"=0, "Pan Tool"=9, "Point Tool"=1, "Line Tool"=2, "Rectangle Tool"=3, "Rotated Rectangle Tool"=12, "Polyline Tool"=10, "Polygon Tool"=5, "Freehand Tool"=11, "Closed Freehand Tool"=6, "Ellipse Tool"=4, "Annulus Tool"=7] ("Current ROI Tool")
                  }
                  frame True {
                    w2175 = u32 3 items=["Zoom Tool"=8, "Selection Tool"=0, "Pan Tool"=9, "Point Tool"=1, "Line Tool"=2, "Rectangle Tool"=3, "Rotated Rectangle Tool"=12, "Polyline Tool"=10, "Polygon Tool"=5, "Freehand Tool"=11, "Closed Freehand Tool"=6, "Ellipse Tool"=4, "Annulus Tool"=7] ("Current ROI Tool")
                  }
                }
                n1283 = local write "Draw ROI"(w2165) -> ()
                n1284 = local write "Zoom"(w2164) -> ()
                n1285 = property on="Property Node" class="ImageControl"(reference=w2161, "Current ROI Tool"=w2166) -> ()  [unwired: 1 in, 2 out]
              }
              event "Zoom to Fit": Value Change {
                # "The various ROI tools are hidden, so the image control resizes nicely as the Red Tweezers window is resized.  The zoom to fit button/mouse mode buttons return some of this functionality."
                n1286 = event-data() -> ("NewVal"=w2179:bool)  [unwired: 1 in]
                n1287 = property on="Property Node" class="ImageControl"(reference=w2176, "Zoom to Fit Mode"=w2179) -> ()  [unwired: 1 in, 2 out]
              }
            }
            n1288 = feedback #14() -> (w2147:T27)  [unwired: 1 in]
            n1289 = call "Smoothed Frame Rate.vi"("Feedback In"=w2147, "Alpha"=0.05) -> ("Feedback Out"=w2146:T27, "Frame Rate"=w2143:dbl)  [unwired: 4 out]
            n1290 = feedback-in #14(w2146) -> ()
            n1291 = global write "red_tweezers_globals_INTERNAL_VOLATILE.vi" "Video Frame Rate"(w2143) -> ()
            n1292 = local read "stop"() -> (w2144:bool)
            n1293 = Unbundle By Name(w2141) -> ("status"=w2134:bool)
            n1294 = Or(x=w2134, y=w2144) -> (x .or. y?=w2148:bool)
          }
          n1295 = call <vilib>:"IMAQdx Close Camera.vi"("error in"=w2121, "Session In"=w2122) -> ()  [unwired: 9 in, 1 out]
        }
        frame condition #3 (active) {
          w2181 = 0 ("element")
          w2183 = 1920 ("dimension size")
          w2182 = 1080 ("dimension size")
          w2184 = T16 0 items=["Grayscale (U8)", "Grayscale (I16)", "Grayscale (SGL)", "Complex (CSG)", "RGB (U32)", "HSL (U32)", "RGB (U64)", "Grayscale (U16)"] ("Image Type")
          (unwired) FALSE ("background subtraction")
          # "This subdiagram generates a blank white image- useful if you don't have a camera"
          n1296 = Build Array(w2181, w2181, w2183, w2182) -> (w2180:i32[])
          n1297 = Initialize Array(u8 255 ("element"), w2182, w2183) -> (w2185:u8[][])
          n1298 = global write "red_tweezers_globals_INTERNAL.vi" "Global ROI"(w2180) -> ()
          n1299 = call "IMAQ Create"("Image Name"="red tweezers camera stub", "Image Type"=w2184) -> ("New Image"=w2186:T8)  [unwired: 2 in, 2 out]
          n1300 = call "IMAQ ArrayToImage"("Image Pixels (U8)"=w2185, "Image"=w2186) -> ("Image Out"=w2189:T8)  [unwired: 8 in, 1 out]
          n1301 = call "IMAQ Create"("Image Name"="Red Tweezers live image") -> ("New Image"=w2190:T8)  [unwired: 3 in, 2 out]
          n1302 = while {
            tunnel: w2189 -> [w2193]
            tunnel: w2190 -> [_]
            stop <- w2197 stop-if-true
            n1303 = local read "stop"() -> (w2197:bool)
            n1304 = Wait Until Next ms Multiple(millisecond multiple=u32 20) -> ()  [unwired: 1 out]
            n1305 = call "imageQ_camera_hook.vi"("Image"=w2193) -> ()  [unwired: 11 in]
            n1306 = feedback #15() -> (w2195:T27)  [unwired: 1 in]
            n1307 = call "Smoothed Frame Rate.vi"("Feedback In"=w2195) -> ("Feedback Out"=w2196:T27, "Frame Rate"=w2194:dbl)  [unwired: 1 in, 4 out]
            n1308 = feedback-in #15(w2196) -> ()
            n1309 = global write "red_tweezers_globals_INTERNAL_VOLATILE.vi" "Video Frame Rate"(w2194) -> ()
          }
        }
        frame condition #4 {
          # "Use this subdiagram if you have an external camera VI which writes to the image queue (using imageQ_camera_hook.vi)"
        }
        frame condition #5 {
          w2198 = path "C:/Users/Tweezer Cube/Desktop/red_tweezers_1_4_rc0/camera_for_rt136.llb/Particle Tracking.vi"  # Path to camera VI
          # "Use this subdiagram if you have an external camera VI which writes to the image queue (using imageQ_camera_hook.vi).  This is the slightly more sophisticated version, which checks that said external VI is running, and runs it if not."
          n1310 = Open VI Reference(vi path=w2198) -> (vi reference=w2199:refnum<vi>, error out=w2201:errorcluster)  [unwired: 5 in]
          n1311 = property class="VI"(reference=w2199) -> ("Path"=w2200:path)  [unwired: 1 in, 2 out]
          n1312 = global write "red_tweezers_globals_INTERNAL_VOLATILE.vi" "Current Camera VI"(w2200) -> ()
          n1313 = property class="VI"(reference=w2199, error in=w2201) -> (reference out=w2206:refnum<vi>, error out=w2205:errorcluster, "Exec.State"=w2203:T29)
          n1314 = Equal?(x=w2203, y=T29."Idle") -> (x = y?=w2207:bool)
          n1315 = case shown="True" w2207 {
            tunnel: w2206 -> [w2211 w2220]
            tunnel: w2205 -> [w2210 w2217]
            tunnel: [w2209 w2216] -> w2202
            tunnel: w2203 -> [w2213 _]
            frame False {
              n1316 = Close Reference(reference=w2211, error in (no error)=w2210) -> (error out=w2209:errorcluster)
              n1317 = Equal?(x=w2213, y=T29."Bad") -> (x = y?=w2212:bool)
              n1318 = case shown="False" w2212 {
                frame False {
                }
                frame True {
                  n1319 = One Button Dialog(message="The external camera VI is not running and cannot be started- it's probably broken or missing.  Check the static/dynamically loaded VI reference in the bottom loop on the block diagram.") -> ()  [unwired: 1 in, 1 out]
                }
              }
            }
            frame True {
              n1320 = invoke class="VI" method="Run VI"(reference=w2220, error in=w2217, "Wait until done"=FALSE ("Wait Until Done"), "Auto Dispose Ref"=TRUE ("Auto Dispose Reference")) -> (error out=w2216:errorcluster)  [unwired: 1 in, 4 out]
            }
          }
          n1321 = call <vilib>:"Simple Error Handler.vi"("error source (\" \")"="External camera VI (see the bottom loop in the block diagram)" ("error source (\" \")"), "error in (no error)"=w2202) -> ()  [unwired: 3 in, 5 out]
        }
      }
    }
  }
  n1322 = while {
    tunnel: w9 -> [w2238]
    shift-right: [w2237] -> w8
    shift-left: w10 -> [w2239]
    shift-right: [w2234] -> _
    shift-left: _ -> [w2227]
    shift-right: [w2233] -> _
    shift-left: _ -> [w2231]
    shift-right: [w2232] -> _
    shift-left: FALSE ("Saving") -> [w2228]
    stop <- w2236 stop-if-true
    w2225 = u32 50 ("millisecond multiple")
    # "Start/stop saving data, if necessary"
    n1323 = Divide(x=u32 1000, y=w2225) -> (x/y=w2223:dbl)
    n1324 = Wait Until Next ms Multiple(millisecond multiple=w2225) -> ()  [unwired: 1 out]
    n1325 = call "imageQ_dequeue.vi"("timeout in ms (-1)"=2000, "Return queue"=w2239, "Image Dst"=w2238) -> ("Timestamp/us"=w2229:u64, "Return queue out"=w2237:refnum<queue>, "Image Dst Out"=w2240:T8, "timed out?"=w2243:bool, "ROI"=w2222:u64[])  [unwired: 4 in]
    n1326 = Not(x=w2243) -> (.not. x?=w2241:bool)
    n1327 = case shown="True" w2241 {
      tunnel: w2240 -> [_ w2277]
      tunnel: w2231 -> [w2270 w2280]
      tunnel: w2228 -> [_ w2274]
      tunnel: [w2270 w2275] -> w2230
      tunnel: w2229 -> [_ w2278]
      tunnel: w2227 -> [w2271 w2279]
      tunnel: [w2271 w2276] -> w2226
      tunnel: w2222 -> [_ w2273]
      frame False {
      }
      frame True {
        n1328 = global read "red_tweezers_globals_INTERNAL.vi" "Image Overlay (extras from control loop)"() -> (w2288:T19[])
        n1329 = case shown="True" w2274 {
          tunnel: w2280 -> [w2289 w2291]
          tunnel: w2279 -> [w2290 w2297]
          tunnel: w2278 -> [_ w2296]
          tunnel: w2277 -> [_ w2295]
          tunnel: [w2290 w2294] -> w2276
          tunnel: [w2289 w2293] -> w2275
          frame False {
          }
          frame True {
            n1330 = call "save_data_save.vi"("Image"=w2295, "Timestamp"=w2296, "Avi Refnum"=w2291, "Data refnum"=w2297) -> ("error out"=w2292:errorcluster, "Avi Refnum (duplicate)"=w2293:T30, "Data refnum (duplicate)"=w2294:refnum<file>)  [unwired: 5 in]
            n1331 = case shown="Error" w2292 {
              selector: w2292 -> [_ w2299]
              frame No Error {
              }
              frame Error {
                n1332 = call <vilib>:"Clear Errors.vi"("error in (no error)"=w2299) -> ()  [unwired: 5 in, 2 out]
                n1333 = local write "Save Video"(FALSE ("Save")) -> ()
              }
            }
          }
        }
        n1334 = global write "red_tweezers_globals_INTERNAL.vi" "Global ROI"(w2273) -> ()
        n1335 = global read "red_tweezers_globals_INTERNAL_VOLATILE.vi" "Tracked Spot Positions (3D)"() -> (w2281:cluster{"x":dbl, "y":dbl, "Z":dbl}[])
        n1336 = global read "red_tweezers_globals.vi" "Selection/Group"() -> (w2287:T7[])
        n1337 = global read "red_tweezers_globals.vi" "Spots"() -> (w2286:T1[])
        n1338 = call "overlay_positions.vi"("Positions"=w2281, "Image"=w2277) -> ("Image 2"=w2283:T8)  [unwired: 9 in]
        n1339 = call "render_overlay_elements.vi"("Image Overlay (extras from control loop)"=w2288, "Image"=w2283) -> ("Image Out"=w2285:T8)  [unwired: 5 in]
        n1340 = call "grid_and_guides.vi"("Operation"=T13."Render on image", "Image"=w2285) -> ("Image Out"=w2272:T8)  [unwired: 9 in]
        n1341 = call "overlay_spots_on_image.vi"("Selection and Groups"=w2287, "Spots"=w2286, "image"=w2272) -> ("Image"=→"Image":T8)  [unwired: 3 in, 1 out]
      }
    }
    n1342 = global read "red_tweezers_globals_INTERNAL_VOLATILE.vi" "Video Frame Rate"() -> (→"Video Frame Rate":dbl)
    n1343 = case shown="True" "Save Video" {
      tunnel: [w2246 w2261] -> w2234
      tunnel: [w2245 w2255] -> w2233
      tunnel: [FALSE ("Saving") w2260] -> w2232
      tunnel: w2228 -> [w2249 w2259]
      tunnel: w2230 -> [w2247 w2258]
      tunnel: w2226 -> [w2248 w2257]
      tunnel: w2223 -> [_ w2256]
      frame False {
        n1344 = case shown="True" w2249 {
          tunnel: w2248 -> [w2251 w2254]
          tunnel: w2247 -> [w2250 w2253]
          tunnel: [w2251 _] -> w2246
          tunnel: [w2250 _] -> w2245
          frame False {
          }
          frame True {
            n1345 = local write "Save Video"(FALSE ("Save")) -> ()
            n1346 = call "save_data_stop.vi"("Avi Refnum"=w2253, "Data refnum"=w2254) -> ()  [unwired: 10 in]
          }
        }
      }
      frame True {
        n1347 = case shown="False" w2259 {
          selector: w2259 -> [_ w2269]
          tunnel: [w2266 w2267] -> w2261
          tunnel: [w2265 w2268] -> w2255
          tunnel: [w2262 w2269] -> w2260
          tunnel: w2258 -> [_ w2268]
          tunnel: w2257 -> [_ w2267]
          tunnel: w2256 -> [w2264 _]
          frame False {
            n1348 = call "save_data_start.vi"("Save Video"=TRUE, "Frames Per Second"=w2264) -> ("Saving"=w2262:bool, "Avi Refnum"=w2265:T30, "Data Refnum"=w2266:refnum<file>)  [unwired: 3 in]
            n1349 = local write "Save Video"(w2262) -> ()
          }
          frame True {
          }
        }
      }
    }
    n1350 = local read "stop"() -> (w2236:bool)
  }
  n1351 = Release Queue(queue=w8) -> ()  [unwired: 2 in, 3 out]
  n1352 = case shown="True" w3 {
    frame False {
    }
    frame True {
      n1353 = One Button Dialog(message="Warning: there was a camera error.  You may need to restart Red Tweezers.") -> ()  [unwired: 1 in, 1 out]
    }
  }
  n1354 = flat-sequence {
    tunnel: w18 -> [w2305]
    tunnel: w17 -> [_]
    frame #0 {
      # "This autosaves when we stop.  The sequence structures are necessary so that:\n1. loading settings doesn't stop the VI\n2. plugins are still open (and hence saved) when we save settings"
      n1355 = local read "Plugins"() -> (w2308:T3)
      n1356 = global read "red_tweezers_globals_INTERNAL_VOLATILE.vi" "Current Settings File"() -> (w2302:path)
      n1357 = global read "red_tweezers_globals_INTERNAL_VOLATILE.vi" "Save Settings On Exit"() -> (w2301:bool)
      n1358 = flat-sequence {
        tunnel: w2305 -> [w2311]
        tunnel: [w2311] -> w2304
        frame #0 {
          n1359 = local write "stop"(FALSE ("STOP")) -> ()
        }
      }
      n1360 = case shown="True" w2301 {
        tunnel: w2302 -> [_ w2316]
        tunnel: w2304 -> [w2313 w2314]
        tunnel: [w2313 w2314] -> w2303
        frame False {
        }
        frame True {
          n1361 = Path To String(path=w2316) -> (string=w2315:string)
          n1362 = call "settings_save_to_file.vi"("XML File Path"=w2316) -> ()  [unwired: 11 in]
          n1363 = call "settings_filename_to_registry.vi"("Last Used Settings File"=w2315) -> ()  [unwired: 11 in]
        }
      }
      n1364 = flat-sequence {
        tunnel: w2303 -> [w2309]
        tunnel: [w2309] -> _
        frame #0 {
          n1365 = local write "stop"(TRUE ("STOP")) -> ()
        }
      }
      n1366 = control-ref of="Plugin Pnl"() -> (w2306:refnum<vi>)
      n1367 = control-ref of="Plugin:"() -> (w2307:refnum<vi>)
      n1368 = call "plugins_unload.vi"("error in (no error)"=w2303, "Plugins"=w2308, "Sub Panel"=w2306, "Plugin Chooser"=w2307) -> ()  [unwired: 2 in, 2 out]
    }
  }
